vi "Rb_HSRL_v1.0_15m_res.vi"() -> ()   [LabVIEW 2012]
uses:
  C:/Users/H2ODial/Desktop/Shared Telescope WV DIAL Code/Libraries and VIs/PowerMeterCommands.dll
  Shared Telescope WV DIAL Code/Libraries and VIs/PowerMeterCommands.dll
  <vilib>/DAQmx/write.llb/DAQmx Write (Digital 1D Bool NChan 1Samp 1Line).vi
  <vilib>/DAQmx/miscellaneous.llb/DAQmx Fill In Error Info.vi
  <vilib>/Analysis/baseanly.llb/Mean (DBL).vi
  NCAR_DIAL_Labview/AMCS_Data.vi
  Libraries and VIs/Scalar_Data.vi
  <vilib>/Analysis/NI_AALBase.lvlib
  Libraries and VIs/Scalar_Data_2.vi
  Libraries and VIs/Scalar_Data_4.vi
  Libraries and VIs/Scalar_Data_3.vi
  Shared Telescope WV DIAL Code/bristol/CLDevIFace.dll
panel:
  out "FileHour":i32=22
  out "L_Count":i32=314
  out "background start":u32=534
  in  "Tab Control 2":enum32{"WV ND narrow", "WV ND wide"}(tab)=enum."WV ND wide"
  out "RingBuffer offline near":dbl[][](array[numeric])
  out "RingBuffer aerosol near":dbl[][](array[numeric])
  in  "?":T1(tab)=enum."NRB combined"
  out "NRB":dbl[][](graph) caption="Water Vapor Number Density"
  out "NRB 2":dbl[][](graph)=[[0.0006041726529339577, 3.7193787603040805e-05, 3.074896066816216e-05, 4.770145553696684e-05, 7.251392535345536e-05, 0.00010516026017191158, 0.00015207278442684095, 0.00021703896370834744, 0.0002984480988834696, 0.0004093343578366007, 0.0005470560080267362, 0.0007198538987867779, 0.0009396502763554047, 0.0012021835436913518, 0.0015364865779630445, 0.0019279361150240316, 0.0024003604564710023, 0.0029556420530327627, 0.0035799089491286695, 0.004304541171244636, 0.005152810472118787, 0.006171071816967221, 0.007336763695905082, 0.008707520567026136, 0.01017449514748215, 0.011772772340331295, 0.013524884389137577, 0.015341812039428549, 0.017348824658566273, 0.019475636480752727, 0.021601086546037672, 0.02380481304574997, 0.02608445492869741, 0.028360551643139206, 0.030718590319288325, 0.03312680937217094, 0.03549024795270195, 0.03783837645383283, 0.04012219712763372, 0.04250981000176668, 0.044828450558781714, 0.04728053416880318, 0.04984268526006494, 0.0521315574013464, 0.054573984158249905, 0.056762556916223, 0.05892610037044928, 0.06119757571231991, 0.06332053027960594, 0.06531927169904322, 0.06723106201969582, 0.06903054395432445, 0.07061647240492175, 0.07213854154224807, 0.07357196076661428, 0.07475226903500741, 0.07624919928103521, 0.07759010121579418, 0.07885548967938193, 0.08021621669987343, 0.08124765580213601, 0.08236653158699134, 0.08351094727159601, 0.08432126957213373, 0.08514676662031577, 0.08597626589255665, 0.08673988804567571, 0.08759949974634346, 0.08848399450328287, 0.08900381219190334, 0.08964787073734286, 0.09025115411555623, 0.0905283068966542, 0.09100012458273404, 0.09150901738585414, 0.09198604872632336, 0.0926586625260569, 0.09306452132773692, 0.093021602216273, 0.09320383514439438, 0.09329282371608977, 0.09357354518332203, 0.09398320828554164, 0.09438699769115352, 0.09413753694666852, 0.0948052588692632, 0.09497790750110588, 0.09484330743286604, 0.09549799508818226, 0.09539843311384517, 0.0952913565982388, 0.09554342190445454, 0.09553947780494176, 0.09582968317978471, 0.09564115749371307, 0.09505642155282434, 0.09429336706098984, 0.09303860704925615, 0.09201905868900799, 0.09062923434706588, 0.08859052388200775, 0.086006286091639, 0.08369404052031999, 0.081904721905929, 0.08004872100022047, 0.07932582904533776, 0.07850488045233898, 0.07784248370481489, 0.07829820113146535, 0.07817718456168067, 0.07868973099619218, 0.07879420259145382, 0.07842026241447664, 0.07835326207404376, 0.07809468028201165, 0.0790833403261559, 0.08104750888680619, 0.08316741131844003, 0.08645617173459792, 0.08894810268275583, 0.09069525008709582, 0.09186830492409764, 0.09167542640721689, 0.09117907609911939, 0.09078044847825219, 0.0904888883269004, 0.0912124641535658, 0.09221245667395658, 0.09271218317409123, 0.09268672550587362, 0.09164929678500609, 0.08909246838104862, 0.08740150716625646, 0.08551898874896055, 0.08341063493914702, 0.08382395459947903, 0.08281486876215985, 0.08138348106905442, 0.0805959394968051, 0.07742003267120832, 0.07494432120303063, 0.07401315583274465, 0.07247425509566857, 0.07240541265691175, 0.07215582852133233, 0.07207907831538843, 0.07189867090225423, 0.0718332040569795, 0.07213153070685697, 0.07161625534702555, 0.07195959596703647, 0.07149272375067008, 0.07135829810518599, 0.07136001159711242, 0.06990104011744806, 0.06987630922547103, 0.06884467447215356, 0.06823257080581079, 0.06883796260577212, 0.06847144325865764, 0.06734517260711312, 0.06723714193820494, 0.06649908929073146, 0.0674060028804214, 0.06927035231342661, 0.06945789501223798, 0.06966274036787448, 0.0681759990175523, 0.06646660267888853, 0.06525933579552161, 0.06363030761253068, 0.0636144997860727, 0.06369191189378652, 0.06441653257646081, 0.06368179845135223, 0.06213643625440458, 0.06089832506358413, 0.058320573481011655, 0.05967725558532747, 0.05856115358251668, 0.059599703986508296, 0.06033573116455784, 0.058409429492027175, 0.058959839825009026, 0.05696379786517486, 0.05560617195512912, 0.056196112405437204, 0.05634353266040761, 0.05628868456217053, 0.05702440299877362, 0.057239692366992695, 0.05587078750756856, 0.05534171474675636, 0.055016014721345825, 0.05398698695389306, 0.0524964636530886, 0.05166880356011147, 0.05003552152440533, 0.049562020331489515, 0.051877112560926565, 0.052172088817809284, 0.053955908621857, 0.052575656190183465, 0.052057255845492936, 0.0507955882759869, 0.04955602257520721, 0.04952174173150179, 0.049791947433534794, 0.05217084485092792, 0.05144685259985514, 0.05331642431809782, 0.05177469378292136, 0.0487257070373867, 0.04890825602438813, 0.048007045410234074, 0.04818622012199576, 0.04925269626343131, 0.04986393338341831, 0.04860105322071905, 0.04921830012224699, 0.047579260972547464, 0.04679108166071056, 0.0467185509232381, 0.04452202248017214, 0.04540124359150138, 0.04585235124493015, 0.04346851158339598, 0.044830276331367304, 0.04543989298598568, 0.046021190551811586, 0.05002834379151057, 0.05047225805881103, 0.04992168026796387, 0.05085616627991155, 0.05200288053238239, 0.05056443855849414, 0.05122981806572211, 0.048885205277262665, 0.04850397541077456, 0.049441989710825654, 0.05049665877316022, 0.05028550089234136, 0.04661988565933452, 0.046645547880938255, 0.04409610958554134, 0.04525258959471702, 0.04696949495607038, 0.04345277024830872, 0.04512310015573092, 0.045748802174906754, 0.04352087638982649, 0.04574143111706206, 0.04373205593808596, 0.04099138210775028, 0.04224107988946424, 0.0395090076562992, 0.04089183484076426, 0.039065056758817274, 0.03448044280507904, 0.036642233230026584, 0.037975871955755, 0.03841786645234208, 0.04211606108025334, 0.04010127474954111, 0.03315324269857886, 0.03494805507331391, 0.03495744695494245, 0.03731190452688696, 0.042163250407491894, 0.04046697866940592, 0.041967686312648037, 0.037319330850630696, 0.036587053106327226, 0.035683334046114845, 0.03445271926835893, 0.03868934714245255, 0.035046751585014836, 0.03685275429097781, 0.03175210231453753, 0.030612837961132663, 0.03176195345327498, 0.027334033309638617, 0.029180900182185707, 0.02865840834546146, 0.024692599756547362, 0.028846881603003485, 0.027710252601683617, 0.0271463616451785, 0.033031871807972034, 0.031118426063762063, 0.035516450652314735, 0.0317593270937277, 0.02880259484360031, 0.02686866254588606, 0.02147381320339014, 0.02149965025192153, 0.022990151503239253, 0.026388513939612456, 0.02545578038086694, 0.025429119622728674, 0.025822281802900048, 0.02524468180256883, 0.02599054050380181, 0.02516669386087913, 0.02551090205112066, 0.0203265957298277, 0.021475081022554975, 0.021043561469039938, 0.018364628869036184, 0.018720587552500965, 0.019901261768221604, 0.02518438548755014, 0.023718103872757065, 0.024130962125967614, 0.019356525904050494, 0.019242576033774845, 0.01957557879878532, 0.019690045998715985, 0.025537381219061506, 0.024257920468234218, 0.024400361376299314, 0.027260112185394682, 0.027839296598898382, 0.023670078435408172, 0.026458849617683574, 0.02633082198123516, 0.022440984172402617, 0.025358281578316287, 0.02435685979145898, 0.02086607078842593, 0.02210307355877256, 0.01943913047031024, 0.01620527149342513, 0.015202754031733812, 0.01257869794949909, 0.015539979726883455, 0.020184590849572564, 0.017759487388499917, 0.018095561255307153, 0.019384571063333245, 0.01416927084808891, 0.022379157570552637, 0.021876468088369096, 0.02077252637847875, 0.02169764331999801, 0.01876314467011202, 0.0209715149156249, 0.017664916654813154, 0.01546464729070044, 0.01566523945804065, 0.014033903002535698, 0.015233910748532533, 0.012385388752067525, 0.009629681175184958, 0.013262514404387455, 0.01472585101517507, 0.022860933244986854, 0.01748948056632007, 0.016504772276149934, 0.014739152225579666, 0.013476648779599306, 0.01845678009403428, 0.018438586402626633, 0.01851612245573369, 0.01511492613370712, 0.020725919810791443, 0.021614056828372277, 0.021868012999440557, 0.023056145435887954, 0.019819022220186062, 0.016583566922346558, 0.014259915677188135, 0.014781268644322328, 0.011182714408497697, 0.011242594967649835, 0.011534969341718871, 0.011972716867189292, 0.013145154589079836, 0.0030906909114922, 0.004609917525458331, 0.0023149795690942843, 0.009454679429801037, 0.020204932639349964, 0.020539446622713443, 0.02466588261751272, 0.011530946627061736, 0.010373812669827698, 0.005177157268376568, 0.003228309463408691, 0.006730392042262006, 0.011105804742031536, 0.01586251718023354, 0.01935602818797239, 0.019936541321503114, 0.008129118486826823, 0.00778377301546927, 0.0003695124616010089, 0.0028732570424632874, 0.012698627123804679, 0.01267471247361873, 0.016643302663523693, 0.019205150480841312, 0.017684577735701913, 0.014449418836640792, 0.01857936241213829, 0.016534205784404298, 0.018657449525901922, 0.01680389187275702, 0.012839133123909214, 0.018074054220304253, 0.014337587540227013, 0.019196167150429416, 0.02017712086168147, 0.007772012350720519, 0.0059856542235612225, 0.0038658020976381434, -0.001211610038685749, 0.0026588266984640006, 0.002847873136112622, 0.002249503156204727, 0.008668141762090026, 0.00846548962847913, 0.01304702938436645, 0.015423065838504587, 0.010911465180731727, 0.0033580279321079533, 0.003590210561130783, 0.0030718746874166254, 0.007018008289627999, 0.012689008733428571, 0.007456705774423298, 0.01200651375887071, 0.008501755137950942, 0.00984800132224176, 0.00951336801095635, 0.008255509107674029, 0.006602229251177009, 0.014846995387272353, 0.010322551017957794, 0.00957424583546323, 0.008570230825333694, -0.0007369830016869763, 0.00680268776517046, 0.004007758037186643, 0.006954645963076217, 0.01081781398041212, 0.007108510226707795, 0.012325990209815242, 0.0018346543299594294, -0.00037566565141508926, 0.004190834566108668, -0.0011997075029852179, 0.00673857284784521, 0.010833018626010922, 0.010616180758992915, 0.015351985425832304, 0.017135478061334263, 0.01203975331201191, 0.011880803878362706, 0.011256476345111953, 0.013963647147185716, 0.017863253979310968, 0.01966297280690196, 0.009625081362139031, 0.009192833987779899, 0.015358617240372094, 0.0105862084342294, 0.014150967427764961, 0.012243469345682755, 0.005579922613068284, 0.008803739750438582, 0.004976648336493482, -0.007196315088714143, -0.002796200190110646, -0.0037143500570671287, -0.009521900470303567, -0.0035795151876628945, -0.004554081320388369, -0.00821791805383435, 0.0026015707836290103, 0.009097049423122174, 0.010831762895684778, 0.0109619495385428, 0.011927030178565896, 0.008991275634743796, -0.011478753776895502, -0.01247874025183937, -0.011029890702884463, -0.003565405364506508, 0.011895765754890056, 0.011372105838269473, 0.015263863660221434, 0.006383491336105966, 0.010130143622349968, 0.006882790646430292, -0.004858604026684928, 0.0064874976298614625, -0.004128047613836712, -0.009509548145192852, -0.009502053209695252, -0.022234993005451315, -0.01931000662420272, -0.005874456818578927, -0.006315267117716475, -0.008994568192146921, -0.015201162198915527, -0.022184083454656965, -0.020457589329755464, -0.014696020060882452, -0.024180811697773256, -0.011593475504387623, -0.006086556637311528, -0.009618166637100878, 0.009543898366423168, 0.000282820096403412, -0.0068626538978823195, -0.0008862976099987548, 0.0006290824873365674, 0.009509153013947958, 0.020803085654100693, 0.020932738797131138, 0.02051562415751724, 0.016898339042232292, 0.0055821066209041465, -0.0019204781033461552, 0.003907145183148379, 0.0072943343329344035, 0.0166375814124623, 0.019281108318633014, 0.005223412722166723, -0.007293186459080129, -0.011118978208631936, -0.009345301699687556, -0.003757171178932974, -0.004215485642780951, -0.009162281740601998, -0.007827510266829383, -0.009415758624697988, -0.0006715741260478119, 0.012237677793137763, 0.007980966893190502, 0.00637449302918737, -0.0031311666539790184, -0.005196056738576728, -0.009120032689758912, -0.013698691351727845, -0.006455449361784827, -0.009988370510691364, -0.0028155123857298227, 0.0040232697379379186, 0.01775830173503018, 0.014095098329617138, 0.019981436111423515, 0.013777111307489744, -0.0016681673270184326, 0.0, 0.0, 0.0, 0.0, 0.0]] caption="Water Vapor Number Density"
  out "raw counts":dbl[][](graph) caption="Water Vapor Number Density"
  out "raw counts near":dbl[][](graph)=[[34181.4, 389.4, 74.39999999999998, 49.39999999999998, 69.39999999999998, 41.39999999999998, 4.399999999999977, 78.39999999999998, 56.39999999999998, 68.39999999999998, 86.39999999999998, 87.39999999999998, 85.39999999999998, 91.39999999999998, 89.39999999999998, 124.39999999999998, 116.39999999999998, 123.39999999999998, 174.39999999999998, 149.39999999999998, 134.39999999999998, 203.39999999999998, 221.39999999999998, 214.39999999999998, 233.39999999999998, 280.4, 299.4, 303.4, 334.4, 322.4, 349.4, 397.4, 334.4, 436.4, 350.4, 392.4, 421.4, 412.4, 467.4, 451.4, 448.4, 474.4, 461.4, 416.4, 460.4, 484.4, 416.4, 476.4, 478.4, 449.4, 450.4, 422.4, 451.4, 425.4, 432.4, 412.4, 430.4, 379.4, 396.4, 386.4, 358.4, 346.4, 334.4, 335.4, 331.4, 319.4, 313.4, 329.4, 280.4, 275.4, 282.4, 302.4, 302.4, 294.4, 263.4, 285.4, 264.4, 317.4, 242.39999999999998, 221.39999999999998, 240.39999999999998, 273.4, 213.39999999999998, 228.39999999999998, 218.39999999999998, 212.39999999999998, 240.39999999999998, 180.39999999999998, 209.39999999999998, 199.39999999999998, 198.39999999999998, 200.39999999999998, 162.39999999999998, 180.39999999999998, 227.39999999999998, 199.39999999999998, 148.39999999999998, 151.39999999999998, 146.39999999999998, 178.39999999999998, 144.39999999999998, 158.39999999999998, 146.39999999999998, 120.39999999999998, 132.39999999999998, 125.39999999999998, 140.39999999999998, 94.39999999999998, 78.39999999999998, 106.39999999999998, 128.39999999999998, 114.39999999999998, 93.39999999999998, 89.39999999999998, 78.39999999999998, 78.39999999999998, 80.39999999999998, 102.39999999999998, 107.39999999999998, 86.39999999999998, 64.39999999999998, 84.39999999999998, 74.39999999999998, 84.39999999999998, 79.39999999999998, 123.39999999999998, 104.39999999999998, 59.39999999999998, 98.39999999999998, 99.39999999999998, 65.39999999999998, 77.39999999999998, 95.39999999999998, 47.39999999999998, 56.39999999999998, 51.39999999999998, 83.39999999999998, 59.39999999999998, 91.39999999999998, 59.39999999999998, 55.39999999999998, 37.39999999999998, 43.39999999999998, 38.39999999999998, 58.39999999999998, 73.39999999999998, 50.39999999999998, 77.39999999999998, 38.39999999999998, 70.39999999999998, 46.39999999999998, 27.399999999999977, 53.39999999999998, 31.399999999999977, 44.39999999999998, 66.39999999999998, 42.39999999999998, -0.6000000000000227, 31.399999999999977, 21.399999999999977, 54.39999999999998, 34.39999999999998, 41.39999999999998, 22.399999999999977, 41.39999999999998, 73.39999999999998, 22.399999999999977, 67.39999999999998, 21.399999999999977, 12.399999999999977, 29.399999999999977, 57.39999999999998, 79.39999999999998, 46.39999999999998, 11.399999999999977, 48.39999999999998, 3.3999999999999773, 16.399999999999977, 43.39999999999998, 43.39999999999998, 18.399999999999977, 39.39999999999998, 50.39999999999998, 10.399999999999977, 30.399999999999977, 37.39999999999998, 32.39999999999998, 26.399999999999977, 2.3999999999999773, 3.3999999999999773, 17.399999999999977, -3.6000000000000227, 19.399999999999977, 25.399999999999977, 18.399999999999977, 16.399999999999977, -6.600000000000023, 45.39999999999998, 30.399999999999977, 39.39999999999998, 38.39999999999998, 34.39999999999998, 0.39999999999997726, 17.399999999999977, 35.39999999999998, 9.399999999999977, 23.399999999999977, 9.399999999999977, 11.399999999999977, 10.399999999999977, 33.39999999999998, 41.39999999999998, 13.399999999999977, 25.399999999999977, 23.399999999999977, 17.399999999999977, -6.600000000000023, 7.399999999999977, 1.3999999999999773, 2.3999999999999773, 19.399999999999977, -1.6000000000000227, 9.399999999999977, 7.399999999999977, 30.399999999999977, -8.600000000000023, 50.39999999999998, 18.399999999999977, -4.600000000000023, 23.399999999999977, 45.39999999999998, 18.399999999999977, 24.399999999999977, 25.399999999999977, 20.399999999999977, -2.6000000000000227, 15.399999999999977, 22.399999999999977, 11.399999999999977, 6.399999999999977, 18.399999999999977, -7.600000000000023, 11.399999999999977, 7.399999999999977, -2.6000000000000227, 21.399999999999977, 55.39999999999998, 1.3999999999999773, -9.600000000000023, 5.399999999999977, 22.399999999999977, 8.399999999999977, 26.399999999999977, 19.399999999999977, 1.3999999999999773, 20.399999999999977, 10.399999999999977, 10.399999999999977, 16.399999999999977, 32.39999999999998, 8.399999999999977, -6.600000000000023, 27.399999999999977, 1.3999999999999773, -4.600000000000023, 5.399999999999977, 28.399999999999977, 18.399999999999977, -5.600000000000023, 17.399999999999977, 0.39999999999997726, -0.6000000000000227, 3.3999999999999773, 21.399999999999977, 17.399999999999977, -7.600000000000023, 16.399999999999977, 32.39999999999998, 48.39999999999998, 23.399999999999977, 4.399999999999977, 8.399999999999977, 14.399999999999977, 14.399999999999977, -1.6000000000000227, 22.399999999999977, -8.600000000000023, -9.600000000000023, 14.399999999999977, 5.399999999999977, 3.3999999999999773, 12.399999999999977, -25.600000000000023, 3.3999999999999773, -11.600000000000023, 6.399999999999977, 4.399999999999977, 12.399999999999977, -2.6000000000000227, 3.3999999999999773, 25.399999999999977, 55.39999999999998, -3.6000000000000227, 1.3999999999999773, 3.3999999999999773, -2.6000000000000227, -2.6000000000000227, -13.600000000000023, 5.399999999999977, 16.399999999999977, 30.399999999999977, 42.39999999999998, -11.600000000000023, 6.399999999999977, 9.399999999999977, 55.39999999999998, 8.399999999999977, -23.600000000000023, 13.399999999999977, 10.399999999999977, -23.600000000000023, -7.600000000000023, -6.600000000000023, 1.3999999999999773, 23.399999999999977, 10.399999999999977, -5.600000000000023, 3.3999999999999773, -35.60000000000002, 28.399999999999977, -19.600000000000023, -10.600000000000023, 9.399999999999977, -26.600000000000023, 8.399999999999977, -15.600000000000023, -9.600000000000023, 17.399999999999977, 3.3999999999999773, 3.3999999999999773, -8.600000000000023, 41.39999999999998, 24.399999999999977, -2.6000000000000227, 31.399999999999977, 19.399999999999977, 9.399999999999977, -8.600000000000023, -19.600000000000023, 3.3999999999999773, -20.600000000000023, -8.600000000000023, -17.600000000000023, 12.399999999999977, -14.600000000000023, -34.60000000000002, 24.399999999999977, 17.399999999999977, 5.399999999999977, 5.399999999999977, 15.399999999999977, 3.3999999999999773, 4.399999999999977, 12.399999999999977, 6.399999999999977, -18.600000000000023, 2.3999999999999773, -17.600000000000023, 15.399999999999977, 39.39999999999998, 20.399999999999977, -8.600000000000023, 2.3999999999999773, 15.399999999999977, 21.399999999999977, 3.3999999999999773, 6.399999999999977, 6.399999999999977, 15.399999999999977, -17.600000000000023, -33.60000000000002, -2.6000000000000227, 0.39999999999997726, 3.3999999999999773, -19.600000000000023, -3.6000000000000227, 23.399999999999977, 15.399999999999977, 0.39999999999997726, -10.600000000000023, -2.6000000000000227, 6.399999999999977, 0.39999999999997726, 6.399999999999977, -8.600000000000023, 9.399999999999977, -14.600000000000023, -8.600000000000023, -3.6000000000000227, 2.3999999999999773, 9.399999999999977, 15.399999999999977, 0.39999999999997726, -6.600000000000023, 9.399999999999977, -19.600000000000023, -28.600000000000023, 16.399999999999977, 38.39999999999998, 26.399999999999977, 2.3999999999999773, -30.600000000000023, -5.600000000000023, -3.6000000000000227, -5.600000000000023, 9.399999999999977, -6.600000000000023, 2.3999999999999773, 5.399999999999977, -13.600000000000023, 17.399999999999977, -0.6000000000000227, 4.399999999999977, -22.600000000000023, 5.399999999999977, -23.600000000000023, 14.399999999999977, -9.600000000000023, -44.60000000000002, -12.600000000000023, -3.6000000000000227, -14.600000000000023, 3.3999999999999773, -14.600000000000023, -3.6000000000000227, -6.600000000000023, 19.399999999999977, 47.39999999999998, 28.399999999999977, 26.399999999999977, -12.600000000000023, 5.399999999999977, -47.60000000000002, 19.399999999999977, 14.399999999999977, 47.39999999999998, -35.60000000000002, -25.600000000000023, -9.600000000000023, -19.600000000000023, -23.600000000000023, 8.399999999999977, 2.3999999999999773, -4.600000000000023, -10.600000000000023, 6.399999999999977, 0.39999999999997726, -22.600000000000023, 2.3999999999999773, 29.399999999999977, 20.399999999999977, 23.399999999999977, 20.399999999999977, 2.3999999999999773, -6.600000000000023, 10.399999999999977, 2.3999999999999773, -16.600000000000023, -18.600000000000023, -7.600000000000023, -29.600000000000023, 21.399999999999977, -7.600000000000023, -27.600000000000023, 3.3999999999999773, 18.399999999999977, 31.399999999999977, 2.3999999999999773, -29.600000000000023, 29.399999999999977, -15.600000000000023, 18.399999999999977, 44.39999999999998, -31.600000000000023, 16.399999999999977, 0.39999999999997726, -32.60000000000002, 5.399999999999977, -19.600000000000023, -5.600000000000023, -12.600000000000023, -12.600000000000023, 20.399999999999977, -39.60000000000002, 16.399999999999977, -1.6000000000000227, 26.399999999999977, 23.399999999999977, -24.600000000000023, 12.399999999999977, 18.399999999999977, 9.399999999999977, -8.600000000000023, 7.399999999999977, 8.399999999999977, 5.399999999999977, 6.399999999999977, -0.6000000000000227, -4.600000000000023, -12.600000000000023, 16.399999999999977, -3.6000000000000227, -31.600000000000023, -23.600000000000023, 17.399999999999977, 25.399999999999977, 17.399999999999977, 11.399999999999977, -7.600000000000023, -14.600000000000023, 6.399999999999977, 3.3999999999999773, 20.399999999999977, 12.399999999999977, -5.600000000000023, -26.600000000000023, -31.600000000000023, 11.399999999999977, 26.399999999999977, -19.600000000000023, -14.600000000000023, 8.399999999999977, 6.399999999999977, 2.3999999999999773, -16.600000000000023, 17.399999999999977, 10.399999999999977, 0.39999999999997726, -4.600000000000023, 27.399999999999977, -20.600000000000023, -1.6000000000000227, 40.39999999999998, 16.399999999999977, -22.600000000000023, -22.600000000000023, -22.600000000000023, -14.600000000000023, -19.600000000000023, -1.6000000000000227, 18.399999999999977, -23.600000000000023, -10.600000000000023, 12.399999999999977, -3.6000000000000227, 4.399999999999977, -10.600000000000023, 39.39999999999998, 8.399999999999977, 0.0]] caption="Water Vapor Number Density"
  out "HSRL combined Smoothed":dbl[](array[numeric])=[8698.912832369948, 146.95618497109825, 54.04867052023122, 47.1671676300578, 45.88971098265895, 46.214855491329466, 49.099248554913295, 53.648381502890174, 58.2856647398844, 64.74809248554915, 71.50965317919076, 79.06167630057804, 87.92728323699421, 96.98797687861271, 107.9691907514451, 119.05734104046243, 131.28855491329483, 144.17728323699424, 156.71052023121388, 170.0356647398844, 184.5920231213873, 201.3940462427746, 219.0284393063584, 238.69028901734106, 256.98797687861276, 274.87236994219654, 292.76832369942196, 308.74953757225427, 325.4200578034682, 341.3087861271676, 354.47930635838145, 366.5631213872831, 377.6483815028902, 386.7668786127167, 395.29289017341034, 402.8969364161849, 408.60069364161836, 412.9894219653178, 415.7350867052022, 418.71341040462414, 420.26832369942184, 422.39115606936406, 424.8001156069363, 424.3434682080924, 424.6989595375722, 422.7423121387282, 420.3897109826588, 418.60069364161836, 415.63682080924843, 411.7943352601154, 407.40705202312125, 402.39838150289006, 396.28132947976866, 389.99375722543346, 383.43739884393057, 375.8290173410404, 370.04433526011553, 363.7032947976878, 357.23508670520226, 351.4084971098265, 344.3781502890173, 337.9720809248554, 331.89693641618493, 324.7509826589595, 317.940289017341, 311.404161849711, 304.882485549133, 298.93306358381506, 293.27988439306364, 286.65416184971104, 280.6700578034683, 274.78132947976883, 268.1440462427746, 262.32179190751447, 256.8160115606937, 251.42005780346824, 246.73508670520232, 241.51543352601158, 235.3463583815029, 229.9619653179191, 224.54578034682083, 219.77265895953764, 215.4576300578035, 211.2712138728324, 205.79578034682083, 202.47063583815032, 198.2119653179191, 193.46774566473994, 190.45618497109828, 186.06167630057809, 181.79867052023124, 178.3449132947977, 174.52988439306358, 171.36080924855494, 167.4489595375723, 162.98364161849713, 158.36658959537573, 153.09491329479772, 148.38104046242773, 143.23942196531792, 137.26687861271677, 130.67150289017343, 124.70907514450869, 119.71341040462428, 114.78855491329479, 111.61947976878612, 108.41283236994221, 105.51976878612717, 104.20040462427747, 102.1584971098266, 100.98508670520232, 99.32323699421967, 97.11225433526013, 95.33624277456647, 93.37815028901736, 92.93739884393064, 93.62381502890173, 94.45040462427747, 96.54000000000002, 97.67294797687862, 97.95184971098269, 97.59924855491332, 95.81890173410406, 93.77121387283239, 91.87526011560695, 90.13393063583814, 89.43017341040462, 89.00387283236994, 88.1050289017341, 86.7321965317919, 84.45907514450866, 80.86658959537573, 78.14549132947977, 75.32757225433525, 72.38826589595377, 71.68161849710984, 69.79000000000002, 67.5949132947977, 65.98219653179193, 62.482196531791935, 59.63104046242776, 58.064566473988464, 56.06601156069365, 55.23797687861273, 54.29144508670521, 53.493757225433534, 52.63682080924856, 51.88104046242774, 51.39982658959537, 50.355028901734094, 49.92872832369941, 48.95473988439305, 48.226416184971086, 47.60358381502889, 46.03132947976877, 45.427283236994214, 44.18884393063583, 43.24375722543351, 43.08046242774566, 42.317456647398835, 41.10647398843929, 40.53566473988438, 39.600693641618484, 39.65271676300577, 40.256763005780336, 39.881040462427734, 39.52121387283236, 38.219190751445076, 36.82179190751444, 35.729306358381486, 34.43161849710981, 34.024104046242755, 33.67294797687859, 33.66572254335258, 32.90271676300576, 31.740867052023102, 30.758208092485532, 29.12670520231212, 29.472080924855476, 28.600693641618484, 28.787109826589578, 28.82323699421964, 27.59924855491328, 27.557341040462415, 26.337687861271668, 25.434508670520227, 25.43017341040462, 25.226416184971093, 24.93595375722543, 24.996647398843926, 24.82901734104046, 23.98364161849711, 23.511098265895953, 23.132485549132944, 22.46774566473988, 21.625260115606935, 21.068901734104045, 20.19751445086705, 19.805895953757222, 20.524104046242776, 20.435953757225434, 20.925838150289017, 20.19028901734104, 19.79578034682081, 19.128150289017345, 18.480751445086707, 18.29, 18.213410404624277, 18.901271676300578, 18.461965317919077, 18.95184971098266, 18.230751445086707, 16.996647398843933, 16.901271676300578, 16.435953757225434, 16.34491329479769, 16.55300578034682, 16.605028901734105, 16.037109826589592, 16.09346820809248, 15.417167630057804, 15.025549132947976, 14.868034682080925, 14.042890173410404, 14.193179190751442, 14.207630057803465, 13.350693641618497, 13.648381502890173, 13.713410404624277, 13.768323699421968, 14.837687861271679, 14.840578034682085, 14.553005780346824, 14.698959537572257, 14.902716763005781, 14.368034682080925, 14.43450867052023, 13.658497109826587, 13.438843930635837, 13.584797687861272, 13.75965317919075, 13.589132947976879, 12.495202312138726, 12.399826589595376, 11.626705202312138, 11.834797687861274, 12.184508670520232, 11.181618497109827, 11.518323699421964, 11.584797687861272, 10.93306358381503, 11.399826589595378, 10.813121387283237, 10.055895953757226, 10.281329479768786, 9.5414450867052, 9.798670520231212, 9.288554913294798, 8.135375722543353, 8.579017341040462, 8.823236994219654, 8.85791907514451, 9.636820809248555, 9.106473988439305, 7.47208092485549, 7.817456647398842, 7.761098265895953, 8.222080924855492, 9.22208092485549, 8.785664739884393, 9.044335260115606, 7.983641618497109, 7.769768786127167, 7.522658959537571, 7.210520231213872, 8.038554913294796, 7.2293063583815025, 7.547225433526012, 6.456184971098265, 6.180173410404624, 6.3665895953757214, 5.44028901734104, 5.766878612716763, 5.623815028901734, 4.811676300578035, 5.581907514450867, 5.324682080924855, 5.180173410404623, 6.25965317919075, 5.856473988439305, 6.638265895953755, 5.895491329479768, 5.310231213872832, 4.920057803468207, 3.905606936416185, 3.88393063583815, 4.125260115606936, 4.703294797687861, 4.506763005780346, 4.47208092485549, 4.511098265895953, 4.381040462427745, 4.480751445086704, 4.310231213872831, 4.34057803468208, 3.4359537572254326, 3.6064739884393053, 3.511098265895953, 3.0443352601156066, 3.083352601156069, 3.2567630057803467, 4.0949132947976885, 3.8319075144508674, 3.873815028901734, 3.0876878612716756, 3.0501156069364157, 3.0833526011560686, 3.0819075144508665, 3.9720809248554914, 3.7495375722543347, 3.7480924855491327, 4.161387283236994, 4.223526011560693, 3.5689017341040463, 3.964855491329479, 3.921502890173409, 3.32179190751445, 3.7307514450867045, 3.561676300578034, 3.0327745664739876, 3.193179190751444, 2.7914450867052016, 2.313121387283236, 2.1570520231213863, 1.7741040462427735, 2.178728323699421, 2.8131213872832372, 2.460520231213873, 2.492312138728324, 2.6541618497109827, 1.928728323699421, 3.028439306358381, 2.9431791907514446, 2.778439306358381, 2.885375722543352, 2.4807514450867045, 2.7567630057803463, 2.308786127167629, 2.0096531791907504, 2.0241040462427735, 1.80300578034682, 1.9460693641618487, 1.5732369942196525, 1.216300578034681, 1.6657225433526004, 1.8391329479768779, 2.8391329479768777, 2.159942196531791, 2.0269942196531776, 1.8001156069364148, 1.6368208092485537, 2.2293063583815016, 2.2148554913294785, 2.211965317919074, 1.7957803468208082, 2.4489595375722537, 2.5399999999999996, 2.555895953757225, 2.6801734104046235, 2.291445086705201, 1.9070520231213859, 1.6310404624277446, 1.6816184971098254, 1.2654335260115595, 1.2654335260115595, 1.291445086705201, 1.3333526011560681, 1.4561849710982648, 0.34057803468208026, 0.505317919075144, 0.25242774566473924, 1.0255491329479767, 2.1801734104046235, 2.204739884393063, 2.6339306358381496, 1.2249710982658948, 1.0963583815028892, 0.5443352601156056, 0.33768786127167505, 0.7004046242774554, 1.1498265895953745, 1.6339306358381491, 1.983641618497109, 2.0327745664739876, 0.8246820809248548, 0.7856647398843923, 0.03710982658959415, 0.28710982658959416, 1.262543352601155, 1.2538728323699408, 1.638265895953756, 1.8810404624277444, 1.7235260115606925, 1.401271676300577, 1.7928901734104037, 1.5876878612716754, 1.7827745664739876, 1.5978034682080917, 1.2148554913294785, 1.7018497109826582, 1.343468208092485, 1.7899999999999994, 1.8723699421965312, 0.7177456647398832, 0.5501156069364149, 0.35358381502890057, -0.11028901734104167, 0.24086705202312014, 0.2567630057803456, 0.20184971098265772, 0.7741040462427735, 0.7524277456647388, 1.1541618497109816, 1.3579190751445076, 0.9561849710982646, 0.29289017341040346, 0.31167630057803347, 0.2654335260115595, 0.6035838150289005, 1.0862427745664727, 0.6353757225433513, 1.018323699421964, 0.7177456647398832, 0.827572254335259, 0.7957803468208081, 0.6873988439306347, 0.5472254335260104, 1.2249710982658946, 0.8478034682080914, 0.7827745664739871, 0.6975144508670509, -0.059710982658960646, 0.5486705202312125, 0.32179190751444964, 0.5558959537572241, 0.8608092485549121, 0.5631213872832358, 0.9720809248554901, 0.14404624277456524, -0.029364161849712148, 0.3261271676300566, -0.09294797687861393, 0.5197687861271664, 0.8319075144508659, 0.8116763005780334, 1.1686127167630045, 1.2986705202312128, 0.9084971098265884, 0.8926011560693629, 0.842023121387282, 1.0399999999999987, 1.3246820809248543, 1.4518497109826578, 0.7076300578034669, 0.6729479768786115, 1.1194797687861262, 0.7683236994219643, 1.0226589595375712, 0.8810404624277448, 0.39982658959537454, 0.6281502890173398, 0.35358381502890046, -0.5091329479768798, -0.19699421965318042, -0.2605780346820822, -0.6652023121387295, -0.24901734104046358, -0.31549132947977, -0.5669364161849723, 0.17872832369942074, 0.6223699421965305, 0.7379768786127158, 0.743757225433525, 0.8058959537572246, 0.6050289017341031, -0.7692485549132959, -0.8328323699421976, -0.7331213872832381, -0.2360115606936427, 0.7842196531791895, 0.7466473988439294, 0.9980924855491318, 0.41572254335259995, 0.6570520231213861, 0.4446242774566462, -0.3126011560693654, 0.41572254335259995, -0.2634682080924868, -0.604508670520232, -0.6016184971098275, -1.4021965317919085, -1.2128901734104056, -0.36751445086705326, -0.39352601156069483, -0.5582658959537584, -0.9397687861271687, -1.3660693641618509, -1.2547976878612728, -0.8978612716763018, -1.4715606936416195, -0.7027745664739893, -0.3675144508670528, -0.5784971098265903, 0.5717919075144497, 0.016878612716761776, -0.40797687861271803, -0.0524855491329492, 0.037109826589594136, 0.5587861271676288, 1.2177456647398832, 1.2206358381502878, 1.1917341040462417, 0.9778612716762993, 0.32179190751444964, -0.11028901734104168, 0.2235260115606924, 0.41572254335259995, 0.9446242774566462, 1.0905780346820797, 0.29433526011560573, -0.4094219653179203, -0.6218497109826602, -0.5206936416184984, -0.20855491329479886, -0.23312138728323822, -0.504797687861273, -0.42965317919075263, -0.5149132947976891, -0.03658959537572379, 0.6642774566473977, 0.43161849710982536, 0.3434682080924843, -0.16809248554913425, -0.2779190751445099, -0.4860115606936429, -0.727341040462429, -0.3415028901734116, -0.5264739884393075, -0.14786127167630178, 0.21052023121387162, 0.9258381502890162, 0.7321965317919064, 1.0342196531791896, 0.7105202312138718, -0.0857225433526024]
  out "HSRL combined":dbl[](array[numeric])=[8700.534921465967, 148.02575916230356, 54.68642670157071, 48.36803664921469, 46.66548429319374, 47.40795811518327, 50.00808900523563, 53.89945026178015, 58.77379581151838, 64.78721204188487, 71.63505235602099, 79.05651832460737, 87.69755235602096, 97.21424083769634, 108.05390052356017, 119.27608638743452, 131.62065445026175, 144.76823298429318, 157.34480366492153, 171.9154842931938, 186.94918848167544, 202.46653141361264, 220.06273560209425, 238.01626963350787, 256.41352094240835, 274.43773560209416, 292.1386518324606, 309.2695418848166, 325.5741884816751, 341.67562827225095, 355.7276570680624, 368.3045549738215, 379.9374083769629, 389.7620157068058, 398.64486910994714, 406.1612303664916, 412.1811910994759, 416.97405759162257, 421.1370157068058, 424.00121727748643, 425.7302748691095, 427.1327617801042, 427.53852094240784, 427.44002617800993, 426.87850785340265, 425.7551439790571, 424.18511780104666, 422.1641753926697, 419.192971204188, 415.2862303664916, 410.56502617800993, 405.65763089005185, 399.4681675392665, 393.6082198952875, 387.2957198952875, 380.28950261780057, 374.59807591622985, 368.10691099476384, 361.8889790575911, 356.0303403141356, 349.29473821989484, 342.43577225130855, 335.6314528795809, 328.4233376963349, 321.78164921465947, 315.36934554973806, 308.57582460732965, 302.14290575916215, 295.55749999999983, 289.22831151832446, 283.2927748691098, 276.9020680628271, 270.29866492146584, 264.31306282722505, 258.0525916230367, 252.55291884816756, 247.75252617801047, 242.33531413612565, 237.26332460732988, 232.08204188481676, 227.0381937172775, 222.06306282722514, 217.32418848167535, 212.73125654450257, 207.86607329842928, 204.05717277486912, 199.5653534031414, 195.2027879581152, 191.2283115183247, 186.66450261780113, 183.03688481675402, 179.05226439790584, 175.33171465968593, 171.63047120418852, 167.68871727748694, 163.6566492146597, 159.17268324607332, 154.23485602094246, 148.95573298429326, 143.51397905759165, 137.4756937172775, 131.7335471204188, 126.44853403141354, 121.4825654450261, 117.31797120418842, 113.227002617801, 109.52117801047117, 106.67693717277484, 104.20704188481672, 102.45147905759158, 100.49205497382195, 98.4933638743455, 96.95573298429316, 95.54212041884817, 95.18446335078535, 95.7387827225131, 96.78982984293194, 98.14617801047119, 100.12850785340312, 101.38341623036648, 101.96947643979055, 101.88603403141359, 100.43609947643976, 98.48191099476438, 96.40075916230364, 94.29899214659687, 92.42890052356022, 90.72569371727752, 87.99238219895292, 85.29015706806288, 81.83891361256552, 78.135052356021, 75.56077225130896, 73.17628272251314, 71.21456806282728, 69.53721204188487, 67.79081151832466, 65.56895287958122, 63.62000000000006, 61.32484293193723, 59.36509162303672, 57.96195026178016, 56.20769633507858, 55.336295811518376, 54.32091623036654, 53.30324607329847, 52.79670157068067, 52.1144371727749, 51.280013089005266, 50.230929319371754, 49.23649214659689, 48.18544502617804, 47.12000000000003, 46.3971596858639, 45.472748691099504, 44.45769633507855, 43.701151832460745, 43.11149214659687, 42.834332460733, 42.30553664921467, 41.73092931937173, 40.884397905759165, 39.962931937172776, 39.5244502617801, 39.03001308900524, 38.582041884816746, 37.86836387434555, 37.12785340314136, 36.50448952879581, 36.107238219895294, 35.611819371727755, 34.96391361256545, 34.30979057591624, 33.462277486911, 32.58400523560209, 31.833678010471207, 30.992709424083774, 30.568298429319377, 30.19297120418848, 29.993363874345555, 29.7090052356021, 28.86901832460733, 28.326806282722515, 27.5673167539267, 26.94002617801047, 26.738455497382194, 26.401740837696334, 26.01103403141361, 25.61967277486911, 24.974712041884807, 24.475693717277473, 24.39061518324606, 23.882761780104698, 23.498599476439782, 23.47078534031413, 22.50416230366492, 22.25252617801047, 22.050301047120417, 21.472748691099476, 21.55684554973822, 21.611164921465967, 21.25318062827225, 20.75547120418848, 20.395196335078538, 20.11116492146597, 19.68740837696335, 19.63734293193717, 19.740418848167536, 19.108874345549737, 18.785248691099476, 18.309136125654447, 18.019541884816746, 17.91352094240837, 18.157630890052353, 18.12785340314136, 17.66319371727748, 17.166793193717275, 16.85200261780104, 16.499253926701567, 16.64486910994764, 16.571897905759158, 16.067971204188478, 15.925628272251306, 15.224057591623033, 15.109528795811514, 14.935445026178005, 14.232238219895287, 14.11836387434555, 14.009397905759162, 13.93282722513089, 14.277395287958113, 14.505471204188478, 14.32746073298429, 14.427264397905756, 14.38603403141361, 14.196897905759162, 14.164829842931939, 13.643232984293196, 13.87098167539267, 13.69657068062827, 13.832696335078534, 14.041465968586387, 13.581714659685863, 13.238782722513088, 12.775431937172772, 12.465876963350786, 12.159267015706806, 11.912539267015708, 11.65435863874346, 11.586295811518331, 11.469476439790581, 11.203769633507857, 10.766924083769634, 10.462604712041884, 10.081387434554973, 10.092185863874342, 10.345130890052355, 10.157303664921464, 9.909267015706806, 9.633416230366493, 9.207369109947644, 8.854620418848167, 8.946897905759162, 8.75678010471204, 8.778704188481676, 9.008416230366493, 8.841858638743457, 8.941335078534031, 8.822552356020942, 8.74859947643979, 8.80455497382199, 8.48714659685864, 8.3569109947644, 8.132107329842933, 8.021832460732986, 8.224057591623039, 8.008416230366493, 7.714568062827226, 7.342840314136127, 7.087604712041886, 7.282303664921468, 7.138324607329844, 6.8614921465968575, 6.732565445026175, 6.0254319371727725, 5.94526178010471, 5.876871727748691, 5.729620418848169, 5.885706806282724, 5.831714659685863, 6.335314136125655, 6.232565445026178, 6.096112565445026, 5.912866492146596, 5.4534424083769615, 5.585968586387433, 5.935117801047119, 6.033612565445026, 5.7427094240837695, 5.232565445026176, 4.967840314136122, 4.801282722513085, 4.8929057591623, 4.58204188481675, 4.609201570680625, 4.558808900523557, 4.738128272251305, 5.137997382198949, 4.859528795811514, 4.678573298429315, 4.178246073298426, 3.8978141361256506, 3.6661387434554933, 3.6196727748691053, 3.9393717277486866, 4.286230366492142, 4.380143979057587, 4.1442146596858604, 3.726675392670153, 3.449188481675389, 3.1023298429319337, 3.2957198952879554, 3.539175392670154, 3.4046858638743416, 3.764306282722509, 3.7593979057591578, 3.5849869109947594, 3.802591623036644, 3.2852486910994725, 2.9887827225130854, 2.9691492146596827, 2.5699345549738193, 2.929882198952876, 3.0244502617801, 3.3143717277486866, 3.5201963350785292, 3.6779188481675344, 3.7158769633507807, 3.539175392670153, 3.4020680628272215, 3.023141361256541, 3.085314136125651, 3.1343979057591578, 3.183481675392666, 3.0463743455497343, 3.0234685863874304, 2.9603141361256506, 2.585968586387431, 2.734528795811515, 2.89388743455497, 2.6870811518324578, 2.9534424083769597, 2.7250392670157035, 2.2067146596858627, 2.400431937172773, 2.51037958115183, 2.5437565445026147, 2.6952617801047087, 2.618036649214657, 2.212931937172774, 2.462277486910993, 2.469803664921464, 2.2306020942408358, 2.1429057591623017, 2.0290314136125644, 2.1645026178010456, 2.160248691099475, 2.234201570680627, 2.1396335078534023, 1.9269371727748685, 1.8860340314136117, 1.9747120418848156, 1.8395680628272242, 1.6759554973821984, 1.737801047120418, 1.705405759162303, 1.8071727748691089, 1.7669240837696327, 1.5467015706806284, 1.408612565445027, 1.2633246073298443, 1.2927748691099485, 1.5499738219895294, 1.6445418848167537, 2.0270680628272233, 2.033285340314135, 1.6232722513088995, 1.255471204188481, 1.0535732984293196, 1.2031151832460731, 1.409267015706806, 1.5120157068062823, 1.476348167539267, 1.1507591623036648, 1.1847905759162305, 1.2832853403141367, 1.1003664921465977, 1.1537041884816766, 0.6864267015706816, 0.8408769633507862, 0.9828926701570679, 1.4390445026177998, 1.8146989528795803, 1.3899607329842922, 1.1834816753926702, 0.7636518324607341, 0.8611649214659693, 1.1586125654450272, 1.245000000000001, 1.7122774869109945, 1.460641361256544, 1.386361256544502, 1.5588089005235588, 1.1150916230366492, 1.263979057591623, 1.3951963350785344, 1.3755628272251308, 1.3133900523560207, 1.2803403141361254, 1.283285340314136, 1.1098560209424089, 1.1412696335078538, 1.0071073298429325, 1.1890445026178007, 1.3572382198952875, 1.0283769633507849, 1.0323036649214652, 0.68217277486911, 0.49172774869109975, 0.9900916230366493, 1.0957853403141362, 1.4292277486910994, 1.3611649214659687, 1.364437172774869, 1.2626701570680625, 1.0928403141361254, 1.169738219895288, 0.8048821989528799, 0.542120418848168, 0.44264397905759206, 0.5254319371727751, 0.7083507853403146, 1.2230759162303666, 1.3035732984293193, 1.096439790575916, 1.0977486910994765, 0.5745157068062832, 0.5434293193717283, 0.28492146596858703, 0.3559293193717281, 0.9590052356020944, 0.8441492146596857, 1.3412041884816754, 0.9138481675392668, 0.698534031413613, 0.6085471204188485, 0.23518324607329866, 0.622945026178011, 0.737801047120419, 0.3003010471204191, 0.6694109947643979, 0.6301439790575916, 0.6170549738219899, 0.961623036649215, 0.7358376963350796, 0.7456544502617811, 0.4472251308900531, 0.7214397905759171, 0.6991884816753933, 0.7597251308900528, 0.9004319371727756, 0.822879581151833, 0.7086780104712047, 0.6432329842931941, 0.6157460732984297, 0.4207198952879582, 0.5535732984293196, 0.6599214659685868, 0.5313219895287962, 0.5735340314136129, 0.6445418848167543, 0.43577225130890074, 0.3114267015706809, 0.17922774869109975, 0.29146596858638796, 0.310772251308901, 0.36541884816753967, 0.6298167539267021, 0.4459162303664925, 0.5431020942408382, 0.9066492146596867, 1.135052356020943, 0.8166623036649218, 0.6955890052356023, 0.3974869109947642, 0.03753926701570678, 0.5352486910994768, 0.6291623036649219, 0.7862303664921471, 0.9050130890052361, 0.8343324607329846, 0.8205890052356023, 0.7829581151832467, 0.7456544502617806, 0.30062827225130934, -0.15617801047120328, -0.3227356020942403, -0.22096858638743397, 0.13407068062827276, 0.41384816753926723, 0.4128664921465971, 0.14912303664921486, 0.1900261780104715, 0.2643062827225134, 0.19035340314136154, 0.2656151832460736, 0.23256544502617804, 0.2973560209424084, 0.5810602094240841, 0.7472905759162309, 0.9940183246073303, 0.9223560209424089, 1.068298429319372, 0.8811256544502618, 0.3549476439790577, 0.28786649214659693, 0.3392408376963343, 0.5120157068062817, 0.9285732984293185, 1.0925130890052348, 0.8824345549738221, 0.6985340314136127, 0.40763089005235625, 0.19166230366492157, -0.23471204188481642, -0.421557591623036, 0.0002356020942409498, 0.10854712041884829, 0.5574999999999999, 0.7322382198952877, 0.3726178010471207, 0.47896596858638774, 0.12719895287958116, 0.09643979057591623, 0.028704188481675292, -0.05146596858638755, 0.30815445026178045, 0.45442408376963384, 0.04964659685863909, 0.049319371727749015, -0.22653141361256546, -0.4294109947643979, -0.2589267015706806, -0.543939790575916, -0.2998298429319365]
  out "Off-Line Bin Readings 2":dbl[](array[numeric])=[34447.0, 655.0, 340.0, 315.0, 335.0, 307.0, 270.0, 344.0, 322.0, 334.0, 352.0, 353.0, 351.0, 357.0, 355.0, 390.0, 382.0, 389.0, 440.0, 415.0, 400.0, 469.0, 487.0, 480.0, 499.0, 546.0, 565.0, 569.0, 600.0, 588.0, 615.0, 663.0, 600.0, 702.0, 616.0, 658.0, 687.0, 678.0, 733.0, 717.0, 714.0, 740.0, 727.0, 682.0, 726.0, 750.0, 682.0, 742.0, 744.0, 715.0, 716.0, 688.0, 717.0, 691.0, 698.0, 678.0, 696.0, 645.0, 662.0, 652.0, 624.0, 612.0, 600.0, 601.0, 597.0, 585.0, 579.0, 595.0, 546.0, 541.0, 548.0, 568.0, 568.0, 560.0, 529.0, 551.0, 530.0, 583.0, 508.0, 487.0, 506.0, 539.0, 479.0, 494.0, 484.0, 478.0, 506.0, 446.0, 475.0, 465.0, 464.0, 466.0, 428.0, 446.0, 493.0, 465.0, 414.0, 417.0, 412.0, 444.0, 410.0, 424.0, 412.0, 386.0, 398.0, 391.0, 406.0, 360.0, 344.0, 372.0, 394.0, 380.0, 359.0, 355.0, 344.0, 344.0, 346.0, 368.0, 373.0, 352.0, 330.0, 350.0, 340.0, 350.0, 345.0, 389.0, 370.0, 325.0, 364.0, 365.0, 331.0, 343.0, 361.0, 313.0, 322.0, 317.0, 349.0, 325.0, 357.0, 325.0, 321.0, 303.0, 309.0, 304.0, 324.0, 339.0, 316.0, 343.0, 304.0, 336.0, 312.0, 293.0, 319.0, 297.0, 310.0, 332.0, 308.0, 265.0, 297.0, 287.0, 320.0, 300.0, 307.0, 288.0, 307.0, 339.0, 288.0, 333.0, 287.0, 278.0, 295.0, 323.0, 345.0, 312.0, 277.0, 314.0, 269.0, 282.0, 309.0, 309.0, 284.0, 305.0, 316.0, 276.0, 296.0, 303.0, 298.0, 292.0, 268.0, 269.0, 283.0, 262.0, 285.0, 291.0, 284.0, 282.0, 259.0, 311.0, 296.0, 305.0, 304.0, 300.0, 266.0, 283.0, 301.0, 275.0, 289.0, 275.0, 277.0, 276.0, 299.0, 307.0, 279.0, 291.0, 289.0, 283.0, 259.0, 273.0, 267.0, 268.0, 285.0, 264.0, 275.0, 273.0, 296.0, 257.0, 316.0, 284.0, 261.0, 289.0, 311.0, 284.0, 290.0, 291.0, 286.0, 263.0, 281.0, 288.0, 277.0, 272.0, 284.0, 258.0, 277.0, 273.0, 263.0, 287.0, 321.0, 267.0, 256.0, 271.0, 288.0, 274.0, 292.0, 285.0, 267.0, 286.0, 276.0, 276.0, 282.0, 298.0, 274.0, 259.0, 293.0, 267.0, 261.0, 271.0, 294.0, 284.0, 260.0, 283.0, 266.0, 265.0, 269.0, 287.0, 283.0, 258.0, 282.0, 298.0, 314.0, 289.0, 270.0, 274.0, 280.0, 280.0, 264.0, 288.0, 257.0, 256.0, 280.0, 271.0, 269.0, 278.0, 240.0, 269.0, 254.0, 272.0, 270.0, 278.0, 263.0, 269.0, 291.0, 321.0, 262.0, 267.0, 269.0, 263.0, 263.0, 252.0, 271.0, 282.0, 296.0, 308.0, 254.0, 272.0, 275.0, 321.0, 274.0, 242.0, 279.0, 276.0, 242.0, 258.0, 259.0, 267.0, 289.0, 276.0, 260.0, 269.0, 230.0, 294.0, 246.0, 255.0, 275.0, 239.0, 274.0, 250.0, 256.0, 283.0, 269.0, 269.0, 257.0, 307.0, 290.0, 263.0, 297.0, 285.0, 275.0, 257.0, 246.0, 269.0, 245.0, 257.0, 248.0, 278.0, 251.0, 231.0, 290.0, 283.0, 271.0, 271.0, 281.0, 269.0, 270.0, 278.0, 272.0, 247.0, 268.0, 248.0, 281.0, 305.0, 286.0, 257.0, 268.0, 281.0, 287.0, 269.0, 272.0, 272.0, 281.0, 248.0, 232.0, 263.0, 266.0, 269.0, 246.0, 262.0, 289.0, 281.0, 266.0, 255.0, 263.0, 272.0, 266.0, 272.0, 257.0, 275.0, 251.0, 257.0, 262.0, 268.0, 275.0, 281.0, 266.0, 259.0, 275.0, 246.0, 237.0, 282.0, 304.0, 292.0, 268.0, 235.0, 260.0, 262.0, 260.0, 275.0, 259.0, 268.0, 271.0, 252.0, 283.0, 265.0, 270.0, 243.0, 271.0, 242.0, 280.0, 256.0, 221.0, 253.0, 262.0, 251.0, 269.0, 251.0, 262.0, 259.0, 285.0, 313.0, 294.0, 292.0, 253.0, 271.0, 218.0, 285.0, 280.0, 313.0, 230.0, 240.0, 256.0, 246.0, 242.0, 274.0, 268.0, 261.0, 255.0, 272.0, 266.0, 243.0, 268.0, 295.0, 286.0, 289.0, 286.0, 268.0, 259.0, 276.0, 268.0, 249.0, 247.0, 258.0, 236.0, 287.0, 258.0, 238.0, 269.0, 284.0, 297.0, 268.0, 236.0, 295.0, 250.0, 284.0, 310.0, 234.0, 282.0, 266.0, 233.0, 271.0, 246.0, 260.0, 253.0, 253.0, 286.0, 226.0, 282.0, 264.0, 292.0, 289.0, 241.0, 278.0, 284.0, 275.0, 257.0, 273.0, 274.0, 271.0, 272.0, 265.0, 261.0, 253.0, 282.0, 262.0, 234.0, 242.0, 283.0, 291.0, 283.0, 277.0, 258.0, 251.0, 272.0, 269.0, 286.0, 278.0, 260.0, 239.0, 234.0, 277.0, 292.0, 246.0, 251.0, 274.0, 272.0, 268.0, 249.0, 283.0, 276.0, 266.0, 261.0, 293.0, 245.0, 264.0, 306.0, 282.0, 243.0, 243.0, 243.0, 251.0, 246.0, 264.0, 284.0, 242.0, 255.0, 278.0, 262.0, 270.0, 255.0, 305.0, 274.0]
  out "HSRL molecular Smoothed":dbl[](array[numeric])=[795.0727407407404, 21.774592592592594, 19.25607407407408, 19.56903703703704, 19.55792592592593, 20.594962962962963, 23.276444444444444, 25.220888888888883, 28.232, 30.087555555555554, 33.28014814814814, 37.15237037037037, 39.87274074074074, 43.743111111111105, 46.85977777777777, 49.80792592592593, 54.2394074074074, 58.09125925925925, 62.459777777777774, 67.03014814814814, 69.90977777777778, 73.05422222222222, 75.91348148148147, 80.28200000000001, 84.29866666666668, 89.65977777777779, 93.99496296296297, 97.59496296296298, 102.38200000000002, 105.87088888888891, 109.54125925925928, 112.38200000000002, 115.4671851851852, 118.04866666666669, 119.86162962962966, 122.50977777777781, 123.50237037037041, 123.54866666666669, 125.40051851851855, 126.91348148148151, 127.61718518518522, 129.53570370370375, 129.28200000000004, 128.52644444444448, 129.20051851851855, 128.28570370370375, 127.68570370370375, 127.02088888888892, 125.46162962962968, 124.28385185185189, 123.0375555555556, 120.25422222222227, 119.13385185185189, 116.59681481481485, 114.51162962962967, 113.62459259259262, 111.70792592592595, 111.594962962963, 111.1097777777778, 110.15792592592595, 108.39311111111112, 106.08755555555558, 103.9597777777778, 101.58940740740742, 99.36533333333335, 98.28940740740742, 97.7708888888889, 95.84866666666667, 94.58570370370371, 92.0708888888889, 89.34311111111111, 87.52088888888889, 84.83385185185186, 83.33385185185186, 80.71533333333333, 79.70051851851852, 78.3394074074074, 76.38014814814815, 74.87088888888889, 73.09125925925926, 71.71162962962961, 70.50607407407406, 70.26162962962962, 68.73014814814815, 67.62274074074074, 66.46903703703703, 64.8357037037037, 63.38755555555555, 62.7782962962963, 60.60607407407407, 58.90237037037037, 57.06718518518518, 55.00237037037036, 53.5894074074074, 51.80237037037036, 51.50792592592592, 50.21533333333333, 49.22829629629629, 48.587555555555554, 47.29125925925925, 46.78199999999999, 45.97829629629629, 45.130148148148145, 43.431999999999995, 41.483851851851846, 40.05422222222222, 38.498666666666665, 37.59311111111111, 36.64311111111111, 36.86903703703703, 36.53014814814814, 35.965333333333334, 36.05977777777778, 34.830148148148155, 34.04125925925926, 33.38014814814815, 32.75051851851852, 33.20422222222222, 31.782000000000004, 31.65792592592593, 30.846814814814813, 30.031999999999996, 30.833851851851847, 30.21348148148148, 29.89311111111111, 28.38385185185185, 27.85237037037037, 27.032, 27.80237037037037, 27.89311111111111, 27.1282962962963, 26.530148148148147, 23.704222222222224, 22.141259259259257, 21.217185185185187, 20.833851851851854, 20.90977777777778, 21.09866666666667, 21.811629629629632, 21.96903703703704, 22.50607407407407, 22.526444444444447, 21.64866666666667, 21.57088888888889, 20.715333333333337, 19.732000000000003, 19.40237037037037, 18.894962962962964, 19.00237037037037, 18.515333333333334, 18.15237037037037, 17.328296296296298, 16.743111111111112, 16.889407407407408, 16.617185185185186, 17.26162962962963, 17.306074074074075, 17.037555555555553, 16.637555555555554, 15.046814814814814, 13.633851851851853, 13.50051851851852, 13.417185185185186, 13.732000000000003, 14.037555555555558, 13.954222222222224, 13.543111111111115, 13.24866666666667, 13.60607407407408, 13.572740740740745, 13.085703703703707, 12.872740740740744, 10.972740740740743, 10.143111111111114, 9.707925925925927, 10.282000000000004, 11.639407407407411, 12.41903703703704, 12.983851851851854, 11.237555555555558, 11.174592592592594, 9.533851851851853, 8.550518518518519, 9.398666666666667, 8.909777777777778, 9.478296296296296, 10.593111111111114, 9.707925925925927, 9.452370370370373, 10.967185185185189, 9.335703703703704, 10.60792592592593, 10.452370370370373, 8.837555555555557, 10.078296296296298, 8.769037037037037, 8.087555555555555, 7.4468148148148146, 6.66162962962963, 6.256074074074074, 7.159777777777778, 7.633851851851851, 7.006074074074075, 7.139407407407408, 6.106074074074075, 5.482000000000001, 6.026444444444445, 6.87088888888889, 8.126444444444445, 8.482000000000001, 8.348666666666666, 7.728296296296296, 6.0153333333333325, 5.976444444444444, 6.0079259259259254, 5.517185185185185, 6.361629629629629, 5.96162962962963, 5.785703703703703, 6.559777777777777, 6.341259259259259, 6.328296296296296, 6.209777777777777, 5.185703703703704, 5.607925925925926, 5.004222222222222, 4.767185185185186, 5.615333333333334, 4.928296296296297, 5.959777777777778, 5.378296296296297, 4.765333333333334, 3.806074074074074, 3.594962962962964, 4.024592592592593, 3.856074074074075, 4.093111111111112, 4.246814814814815, 4.080148148148149, 4.150518518518519, 4.663481481481482, 4.543111111111113, 4.361629629629631, 3.4986666666666677, 3.19125925925926, 1.8597777777777786, 1.7431111111111117, 1.9375555555555561, 2.0486666666666675, 3.31162962962963, 3.372740740740741, 3.1560740740740747, 2.7820000000000005, 1.4616296296296305, 1.443111111111112, 2.944962962962964, 3.8282962962962968, 4.659777777777778, 4.4431111111111115, 3.9097777777777782, 3.8708888888888895, 4.407925925925926, 4.785703703703704, 3.933851851851852, 3.119037037037037, 1.8579259259259264, 1.1820000000000008, 2.3708888888888895, 2.9764444444444456, 3.2357037037037046, 4.448666666666667, 3.4394074074074075, 3.8245925925925928, 4.394962962962963, 3.987555555555556, 4.585703703703705, 4.306074074074075, 4.482, 4.557925925925926, 4.500518518518518, 3.894962962962963, 3.0486666666666675, 2.9153333333333338, 2.3801481481481486, 2.574592592592593, 2.9838518518518526, 3.2338518518518518, 3.7412592592592593, 4.691259259259259, 5.324592592592593, 3.6468148148148156, 3.54125925925926, 2.7227407407407416, 2.032000000000001, 2.667185185185186, 2.8097777777777786, 2.2153333333333345, 1.7579259259259266, 2.150518518518519, 1.2838518518518527, 1.7116296296296305, 2.180148148148149, 1.9857037037037044, 1.8708888888888895, 1.9671851851851858, 1.8597777777777784, 1.717185185185186, 1.139407407407408, 0.35792592592592676, -0.058740740740739955, 0.6838518518518528, 1.32088888888889, 2.485703703703705, 1.8134814814814826, 1.017185185185186, 1.4968148148148157, 0.29125925925926, 0.5616296296296305, 1.9079259259259267, 1.619037037037038, 2.5116296296296303, 2.7523703703703712, 1.4245925925925933, 1.1616296296296305, 0.9708888888888897, 0.5523703703703713, 1.293111111111112, 1.4486666666666674, 0.9949629629629637, 1.3412592592592603, 1.2838518518518527, 1.069037037037038, 0.33940740740740816, 0.45977777777777856, -0.669851851851851, -0.9050370370370362, -0.6476296296296288, 0.35051851851851934, -0.3828148148148143, -0.16985185185185128, -0.38466666666666616, -1.3883703703703698, -0.2902222222222215, -0.38096296296296217, -0.20874074074074, 0.17459259259259335, 0.4264444444444452, 1.043111111111112, 1.9023703703703712, 1.6820000000000008, 1.9838518518518526, 1.5616296296296304, 1.2986666666666675, 0.8060740740740749, 0.504222222222223, 1.39125925925926, 1.0579259259259268, 1.8542222222222229, 2.9542222222222225, 1.6764444444444448, 2.898666666666667, 1.878296296296297, 0.4190370370370379, 1.0875555555555565, 0.3634814814814823, 1.3560740740740749, 1.4171851851851858, 0.6227407407407415, 0.028296296296297097, -1.2976296296296288, -0.5494814814814809, 0.6857037037037043, 0.8449629629629636, 0.7468148148148154, -0.0642962962962954, -0.014296296296295363, 0.13200000000000092, 1.265333333333334, 1.54125925925926, 1.1820000000000008, 1.517185185185186, 2.0153333333333343, 1.6116296296296304, 1.6357037037037045, 1.206074074074075, 1.813481481481482, 1.8023703703703706, 1.1468148148148154, 0.7690370370370375, -1.380962962962962, -0.5772592592592584, -0.09762962962962879, 0.9282962962962973, 2.3986666666666676, 3.035703703703705, 3.3097777777777786, 2.435703703703705, 2.0171851851851863, 0.5690370370370379, 0.24311111111111192, 0.7579259259259268, 0.42088888888888965, 0.3523703703703712, 0.74125925925926, 1.3245925925925932, 1.665333333333334, 2.0597777777777786, 2.9431111111111115, 2.2282962962962967, 2.270888888888889, 1.4412592592592595, 0.8745925925925929, 0.7431111111111115, 0.19311111111111146, 0.613481481481482, -0.27170370370370295, 0.1560740740740748, 0.7005185185185192, 1.1375555555555563, 1.554222222222223, 2.4338518518518524, 1.8486666666666673, 1.876444444444445, 1.4949629629629635, 0.35237037037037117, 0.49866666666666737, 1.2245925925925931, 0.5801481481481487, 0.1986666666666671, 0.6338518518518523, -0.6402222222222215, 0.03570370370370449, 0.9894074074074082, 0.9042222222222229, 1.8338518518518525, 1.3634814814814822, 0.8431111111111118, 0.4912592592592601, 0.004222222222223071, 0.05792592592592674, -0.595777777777777, -0.2976296296296289, -0.016148148148147468, 0.25792592592592667, 1.4931111111111117, 0.8486666666666675, 0.5449629629629638, 0.7727407407407415, -0.4920740740740733, -0.24022222222222145, -0.12725925925925846, 0.13200000000000084, 1.1338518518518526, 1.4505185185185194, 1.419037037037038, 1.1616296296296302, 0.7190370370370379, 0.5931111111111119, 0.3912592592592601, -0.014296296296295516, 0.4949629629629637, 0.7820000000000008, 0.5727407407407415, 0.9579259259259267, 0.9690370370370379, 0.7134814814814823, 1.5227407407407414, 0.9097777777777785, 0.17644444444444515, 0.7634814814814823, 0.4560740740740749, 1.4949629629629637, 1.5857037037037045, 1.0468148148148158, 1.8931111111111125, 0.998666666666668, -0.267999999999999, -0.43837037037036947, -0.7902222222222217, -0.4605925925925922, 1.1820000000000008, 0.9060740740740749, 0.09681481481481555, 0.01348148148148226, 0.4394074074074082, 0.5894074074074082, 0.9486666666666674, 0.9523703703703711, 0.03570370370370446, 0.8523703703703711, -0.24948148148148075, -0.12911111111111037, 0.21903703703703778, -0.49948148148148075, -0.24948148148148064, -1.0142962962962954, -0.4605925925925918, -0.26244444444444365, 0.7153333333333342, 1.1486666666666674, -0.042074074074073264, -0.5105925925925918, -0.4217037037037029, 0.23570370370370441, 0.6857037037037044, 1.6782962962962968, 2.11162962962963, 1.937555555555556, 1.9745925925925931, 2.013481481481482, 1.3875555555555563, 1.067185185185186, 1.467185185185186, 0.6357037037037045, -0.2883703703703696, -0.23837037037036957, -1.332814814814814, -1.295777777777777, -1.1161481481481474, -0.8365185185185178, -0.30318518518518445, 0.13385185185185267, 1.143111111111112, 0.8986666666666676, 1.7745925925925934, 1.0968148148148158, 1.228296296296297, 0.628296296296297, 0.037555555555556175, 0.178296296296297, -1.160592592592592, -0.1865185185185178, -0.6346666666666658, -0.582814814814814, 0.9208888888888895, 0.9134814814814822, 1.3949629629629636, 1.137555555555556, -0.1531851851851843, -0.956888888888888, -1.2772592592592584, -0.5865185185185178, 0.4653333333333341, 0.4653333333333341, 0.3653333333333342, -0.019851851851851066, -1.2531851851851843, -0.8365185185185177, -1.1791111111111103, -0.5531851851851843, 0.48200000000000076, 0.1931111111111119, 1.3560740740740749, 1.254222222222223, 0.20051851851851932]
  out "On-Line Bin Readings 2":dbl[](array[numeric])=[3592.0, 538.0, 475.0, 472.0, 501.0, 508.0, 483.0, 476.0, 494.0, 546.0, 543.0, 505.0, 531.0, 525.0, 520.0, 503.0, 503.0, 503.0, 553.0, 489.0, 527.0, 520.0, 575.0, 550.0, 570.0, 561.0, 574.0, 621.0, 579.0, 532.0, 619.0, 596.0, 578.0, 630.0, 637.0, 629.0, 623.0, 646.0, 578.0, 612.0, 609.0, 642.0, 540.0, 589.0, 622.0, 582.0, 625.0, 608.0, 596.0, 609.0, 616.0, 621.0, 607.0, 606.0, 623.0, 615.0, 575.0, 637.0, 610.0, 600.0, 592.0, 584.0, 581.0, 575.0, 586.0, 573.0, 594.0, 578.0, 585.0, 609.0, 613.0, 603.0, 589.0, 562.0, 585.0, 590.0, 590.0, 578.0, 523.0, 540.0, 573.0, 561.0, 548.0, 548.0, 540.0, 494.0, 507.0, 518.0, 549.0, 540.0, 513.0, 531.0, 567.0, 541.0, 541.0, 548.0, 543.0, 503.0, 566.0, 538.0, 518.0, 499.0, 539.0, 511.0, 541.0, 518.0, 492.0, 570.0, 498.0, 501.0, 477.0, 510.0, 531.0, 512.0, 512.0, 531.0, 499.0, 489.0, 559.0, 519.0, 492.0, 496.0, 536.0, 522.0, 518.0, 525.0, 498.0, 510.0, 496.0, 515.0, 512.0, 518.0, 485.0, 520.0, 514.0, 542.0, 535.0, 457.0, 505.0, 503.0, 484.0, 489.0, 528.0, 511.0, 522.0, 501.0, 474.0, 522.0, 556.0, 507.0, 467.0, 516.0, 522.0, 509.0, 480.0, 499.0, 499.0, 520.0, 487.0, 522.0, 532.0, 510.0, 486.0, 488.0, 499.0, 473.0, 510.0, 489.0, 502.0, 479.0, 495.0, 493.0, 458.0, 517.0, 495.0, 546.0, 475.0, 463.0, 494.0, 495.0, 493.0, 505.0, 503.0, 511.0, 494.0, 489.0, 470.0, 481.0, 446.0, 501.0, 492.0, 471.0, 477.0, 506.0, 511.0, 451.0, 505.0, 449.0, 534.0, 501.0, 475.0, 539.0, 476.0, 502.0, 480.0, 510.0, 462.0, 501.0, 484.0, 520.0, 469.0, 461.0, 447.0, 478.0, 487.0, 496.0, 480.0, 478.0, 487.0, 484.0, 452.0, 483.0, 495.0, 473.0, 531.0, 484.0, 486.0, 495.0, 493.0, 522.0, 482.0, 480.0, 508.0, 479.0, 514.0, 470.0, 499.0, 459.0, 461.0, 481.0, 469.0, 511.0, 493.0, 491.0, 495.0, 495.0, 482.0, 493.0, 532.0, 503.0, 484.0, 491.0, 503.0, 500.0, 491.0, 468.0, 488.0, 458.0, 506.0, 501.0, 507.0, 486.0, 510.0, 515.0, 464.0, 496.0, 506.0, 480.0, 470.0, 498.0, 473.0, 495.0, 490.0, 449.0, 496.0, 481.0, 460.0, 464.0, 520.0, 464.0, 488.0, 458.0, 515.0, 498.0, 471.0, 511.0, 475.0, 476.0, 468.0, 452.0, 502.0, 498.0, 472.0, 452.0, 496.0, 456.0, 461.0, 500.0, 493.0, 468.0, 487.0, 502.0, 509.0, 509.0, 477.0, 456.0, 451.0, 520.0, 498.0, 469.0, 479.0, 515.0, 466.0, 520.0, 462.0, 454.0, 506.0, 473.0, 492.0, 508.0, 507.0, 478.0, 456.0, 500.0, 501.0, 513.0, 508.0, 507.0, 497.0, 431.0, 463.0, 489.0, 496.0, 477.0, 441.0, 451.0, 509.0, 519.0, 448.0, 473.0, 525.0, 479.0, 465.0, 498.0, 458.0, 508.0, 464.0, 472.0, 475.0, 503.0, 479.0, 464.0, 483.0, 484.0, 511.0, 481.0, 462.0, 474.0, 476.0, 466.0, 496.0, 502.0, 510.0, 502.0, 502.0, 480.0, 489.0, 475.0, 455.0, 518.0, 520.0, 469.0, 490.0, 458.0, 498.0, 486.0, 483.0, 454.0, 464.0, 460.0, 472.0, 481.0, 488.0, 445.0, 453.0, 480.0, 519.0, 512.0, 485.0, 472.0, 480.0, 494.0, 482.0, 457.0, 526.0, 470.0, 485.0, 452.0, 497.0, 521.0, 480.0, 510.0, 467.0, 477.0, 520.0, 497.0, 496.0, 492.0, 442.0, 473.0, 505.0, 459.0, 491.0, 466.0, 475.0, 481.0, 470.0, 485.0, 462.0, 492.0, 475.0, 515.0, 491.0, 460.0, 513.0, 494.0, 472.0, 461.0, 495.0, 480.0, 496.0, 505.0, 496.0, 476.0, 487.0, 480.0, 505.0, 501.0, 472.0, 476.0, 461.0, 487.0, 467.0, 478.0, 463.0, 499.0, 466.0, 519.0, 497.0, 486.0, 454.0, 470.0, 516.0, 476.0, 459.0, 492.0, 501.0, 498.0, 477.0, 442.0, 465.0, 444.0, 487.0, 455.0, 450.0, 500.0, 497.0, 498.0, 473.0, 496.0, 503.0, 500.0, 494.0, 484.0, 460.0, 492.0, 486.0, 477.0, 484.0, 469.0, 511.0, 474.0, 494.0, 462.0, 474.0, 511.0, 504.0, 481.0, 476.0, 510.0, 485.0, 457.0, 510.0, 483.0, 507.0, 438.0, 438.0, 462.0, 505.0, 492.0, 486.0, 496.0, 479.0, 467.0, 477.0, 481.0, 488.0, 462.0, 435.0, 462.0, 501.0, 468.0, 495.0, 457.0, 468.0, 463.0, 506.0, 476.0, 503.0, 456.0, 421.0, 479.0, 478.0, 465.0, 449.0, 483.0, 471.0, 493.0, 511.0, 491.0, 551.0, 488.0, 463.0, 458.0, 477.0, 504.0, 484.0, 472.0, 463.0, 532.0, 439.0, 481.0, 490.0, 440.0, 484.0, 504.0, 459.0, 505.0, 526.0, 497.0, 468.0, 482.0, 516.0, 434.0, 477.0, 488.0, 478.0, 478.0, 500.0]
  in  "stop":bool
  in  "Reset Average":bool=TRUE
  in  "Save Data?":bool=TRUE
  in  "Collect Data?":bool=TRUE
  in  "ILX Address":i32=6 min=0 step=1
  in  "Lambda On DBR Current":dbl=171.13999999999868
  in  "Lambda Off DBR Current":dbl=172.9499999999997
  in  "Tab Control":T2(tab)=enum."NRB"
  out "NRB plot":cluster{"Y":dbl[], "Y":dbl[]}[](graph)=[{"Y"=[0.0, 0.0, 0.0, 0.0, 0.0, 0.0, 0.0, 0.0, 0.0, 0.0, 0.0, 0.0, 0.0, 0.0, 0.0, 0.0, 0.0, 0.0, 0.0, 0.0, 0.0, 0.0, 0.0, 0.0, 0.0, 0.0, 0.0, 0.0, 0.0, 0.0, 0.0, 0.0, 0.0, 0.0, 0.0, 0.0, 0.0, 0.0, 0.0, 0.0, 0.0, 0.0, 0.0, 0.0, 0.0, 0.0, 0.0, 0.0, 0.0, 0.0, 0.0, 0.0, 0.0, 0.0, 0.0, 0.0, 0.0, 0.0, 0.0, 0.0, 0.0, 0.0, 0.0, 0.0, 0.0, 0.0, 0.0, 0.0, 0.0, 0.0, 0.0, 0.0, 0.0, 0.0, 0.0, 0.0, 0.0, 0.0, 0.0, 0.0, 0.0, 0.0, 0.0, 0.0, 0.0, 0.0, 0.0, 0.0, 0.0, 0.0, 0.0, 0.0, 0.0, 0.0, 0.0, 0.0, 0.0, 0.0, 0.0, 0.0, 0.0, 0.0, 0.0, 0.0, 0.0, 0.0, 0.0, 0.0, 0.0, 0.0, 0.0, 0.0, 0.0, 0.0, 0.0, 0.0, 0.0, 0.0, 0.0, 0.0, 0.0, 0.0, 0.0, 0.0, 0.0, 0.0, 0.0, 0.0, 0.0, 0.0, 0.0, 0.0, 0.0, 0.0, 0.0, 0.0, 0.0, 0.0, 0.0, 0.0, 0.0, 0.0, 0.0, 0.0, 0.0, 0.0, 0.0, 0.0, 0.0, 0.0, 0.0, 0.0, 0.0, 0.0, 0.0, 0.0, 0.0, 0.0, 0.0, 0.0, 0.0, 0.0, 0.0, 0.0, 0.0, 0.0, 0.0, 0.0, 0.0, 0.0, 0.0, 0.0, 0.0, 0.0, 0.0, 0.0, 0.0, 0.0, 0.0, 0.0, 0.0, 0.0, 0.0, 0.0, 0.0, 0.0, 0.0, 0.0, 0.0, 0.0, 0.0, 0.0, 0.0, 0.0, 0.0, 0.0, 0.0, 0.0, 0.0, 0.0, 0.0, 0.0, 0.0, 0.0, 0.0, 0.0, 0.0, 0.0, 0.0, 0.0, 0.0, 0.0, 0.0, 0.0, 0.0, 0.0, 0.0, 0.0, 0.0, 0.0, 0.0, 0.0, 0.0, 0.0, 0.0, 0.0, 0.0, 0.0, 0.0, 0.0, 0.0, 0.0, 0.0, 0.0, 0.0, 0.0, 0.0, 0.0, 0.0, 0.0, 0.0, 0.0, 0.0, 0.0, 0.0, 0.0, 0.0, 0.0, 0.0, 0.0, 0.0, 0.0, 0.0, 0.0, 0.0, 0.0, 0.0, 0.0, 0.0, 0.0, 0.0, 0.0, 0.0, 0.0, 0.0, 0.0, 0.0, 0.0, 0.0, 0.0, 0.0, 0.0, 0.0, 0.0, 0.0, 0.0, 0.0, 0.0, 0.0, 0.0, 0.0, 0.0, 0.0, 0.0, 0.0, 0.0, 0.0, 0.0, 0.0, 0.0, 0.0, 0.0, 0.0, 0.0, 0.0, 0.0, 0.0, 0.0, 0.0, 0.0, 0.0, 0.0, 0.0, 0.0, 0.0, 0.0, 0.0, 0.0, 0.0, 0.0, 0.0, 0.0, 0.0, 0.0, 0.0, 0.0, 0.0, 0.0, 0.0, 0.0, 0.0, 0.0, 0.0, 0.0, 0.0, 0.0, 0.0, 0.0, 0.0, 0.0, 0.0, 0.0, 0.0, 0.0, 0.0, 0.0, 0.0, 0.0, 0.0, 0.0, 0.0, 0.0, 0.0, 0.0, 0.0, 0.0, 0.0, 0.0, 0.0, 0.0, 0.0, 0.0, 0.0, 0.0, 0.0, 0.0, 0.0, 0.0, 0.0, 0.0, 0.0, 0.0, 0.0, 0.0, 0.0, 0.0, 0.0, 0.0, 0.0, 0.0, 0.0, 0.0, 0.0, 0.0, 0.0, 0.0, 0.0, 0.0, 0.0, 0.0, 0.0, 0.0, 0.0, 0.0, 0.0, 0.0, 0.0, 0.0, 0.0, 0.0, 0.0, 0.0, 0.0, 0.0, 0.0, 0.0, 0.0, 0.0, 0.0, 0.0, 0.0, 0.0, 0.0, 0.0, 0.0, 0.0, 0.0, 0.0, 0.0, 0.0, 0.0, 0.0, 0.0, 0.0, 0.0, 0.0, 0.0, 0.0, 0.0, 0.0, 0.0, 0.0, 0.0, 0.0, 0.0, 0.0, 0.0, 0.0, 0.0, 0.0, 0.0, 0.0, 0.0, 0.0, 0.0, 0.0, 0.0, 0.0, 0.0, 0.0, 0.0, 0.0, 0.0, 0.0, 0.0, 0.0, 0.0, 0.0, 0.0, 0.0, 0.0, 0.0, 0.0, 0.0, 0.0, 0.0, 0.0, 0.0, 0.0, 0.0, 0.0, 0.0, 0.0, 0.0, 0.0, 0.0, 0.0, 0.0, 0.0, 0.0, 0.0, 0.0, 0.0, 0.0, 0.0, 0.0, 0.0, 0.0, 0.0, 0.0, 0.0, 0.0, 0.0, 0.0, 0.0, 0.0, 0.0, 0.0, 0.0, 0.0, 0.0, 0.0, 0.0, 0.0, 0.0, 0.0, 0.0, 0.0, 0.0, 0.0, 0.0, 0.0, 0.0, 0.0, 0.0, 0.0, 0.0, 0.0, 0.0, 0.0, 0.0, 0.0, 0.0, 0.0, 0.0, 0.0, 0.0, 0.0, 0.0, 0.0, 0.0, 0.0, 0.0, 0.0, 0.0, 0.0, 0.0, 0.0, 0.0, 0.0, 0.0, 0.0, 0.0, 0.0, 0.0, 0.0, 0.0, 0.0, 0.0, 0.0, 0.0, 0.0, 0.0, 0.0, 0.0, 0.0, 0.0, 0.0, 0.0, 0.0, 0.0, 0.0, 0.0, 0.0, 0.0], "Y"=[0.0375, 0.075, 0.11249999999999999, 0.15, 0.1875, 0.225, 0.26249999999999996, 0.3, 0.33749999999999997, 0.37499999999999994, 0.4125, 0.44999999999999996, 0.48749999999999993, 0.525, 0.5625, 0.6, 0.6375, 0.6749999999999999, 0.7124999999999999, 0.75, 0.7875, 0.825, 0.8624999999999999, 0.8999999999999999, 0.9374999999999999, 0.975, 1.0125, 1.05, 1.0875000000000001, 1.125, 1.1625, 1.2, 1.2375, 1.2750000000000001, 1.3125, 1.35, 1.3875, 1.425, 1.4625000000000001, 1.5, 1.5375, 1.575, 1.6125, 1.6500000000000001, 1.6875, 1.725, 1.7625, 1.8, 1.8375, 1.875, 1.9125, 1.95, 1.9875, 2.025, 2.0625, 2.1, 2.1375, 2.175, 2.2125, 2.25, 2.2875, 2.325, 2.3625, 2.4, 2.4375, 2.475, 2.5125, 2.55, 2.5875, 2.625, 2.6625, 2.7, 2.7375, 2.775, 2.8125, 2.85, 2.8875, 2.925, 2.9625, 3.0, 3.0375, 3.075, 3.1125, 3.15, 3.1875, 3.225, 3.2625, 3.3, 3.3375, 3.375, 3.4125, 3.45, 3.4875, 3.525, 3.5625, 3.6, 3.6374999999999997, 3.675, 3.7125, 3.75, 3.7875, 3.8249999999999997, 3.8625, 3.9, 3.9375, 3.975, 4.012499999999999, 4.05, 4.0874999999999995, 4.124999999999999, 4.1625, 4.199999999999999, 4.2375, 4.2749999999999995, 4.312499999999999, 4.35, 4.387499999999999, 4.425, 4.4624999999999995, 4.499999999999999, 4.5375, 4.574999999999999, 4.6125, 4.6499999999999995, 4.687499999999999, 4.725, 4.762499999999999, 4.8, 4.8374999999999995, 4.874999999999999, 4.9125, 4.949999999999999, 4.9875, 5.0249999999999995, 5.062499999999999, 5.1, 5.137499999999999, 5.175, 5.2124999999999995, 5.249999999999999, 5.2875, 5.324999999999999, 5.3625, 5.3999999999999995, 5.437499999999999, 5.475, 5.512499999999999, 5.55, 5.5874999999999995, 5.624999999999999, 5.6625, 5.699999999999999, 5.7375, 5.7749999999999995, 5.812499999999999, 5.85, 5.887499999999999, 5.925, 5.9624999999999995, 5.999999999999999, 6.0375, 6.074999999999999, 6.1125, 6.1499999999999995, 6.187499999999999, 6.225, 6.262499999999999, 6.3, 6.3374999999999995, 6.374999999999999, 6.4125, 6.449999999999999, 6.4875, 6.5249999999999995, 6.562499999999999, 6.6, 6.637499999999999, 6.675, 6.7124999999999995, 6.749999999999999, 6.7875, 6.824999999999999, 6.8625, 6.8999999999999995, 6.937499999999999, 6.975, 7.012499999999999, 7.05, 7.0874999999999995, 7.124999999999999, 7.1625, 7.199999999999999, 7.237499999999999, 7.2749999999999995, 7.312499999999999, 7.35, 7.387499999999999, 7.424999999999999, 7.4624999999999995, 7.499999999999999, 7.5375, 7.574999999999999, 7.612499999999999, 7.6499999999999995, 7.687499999999999, 7.725, 7.762499999999999, 7.799999999999999, 7.8374999999999995, 7.874999999999999, 7.9125, 7.949999999999999, 7.987499999999999, 8.025, 8.0625, 8.1, 8.1375, 8.174999999999999, 8.212499999999999, 8.25, 8.2875, 8.325, 8.362499999999999, 8.399999999999999, 8.4375, 8.475, 8.5125, 8.549999999999999, 8.587499999999999, 8.625, 8.6625, 8.7, 8.737499999999999, 8.774999999999999, 8.8125, 8.85, 8.8875, 8.924999999999999, 8.962499999999999, 9.0, 9.0375, 9.075, 9.112499999999999, 9.149999999999999, 9.1875, 9.225, 9.2625, 9.299999999999999, 9.337499999999999, 9.375, 9.4125, 9.45, 9.487499999999999, 9.524999999999999, 9.5625, 9.6, 9.6375, 9.674999999999999, 9.712499999999999, 9.75, 9.7875, 9.825, 9.862499999999999, 9.899999999999999, 9.9375, 9.975, 10.0125, 10.049999999999999, 10.087499999999999, 10.125, 10.1625, 10.2, 10.237499999999999, 10.274999999999999, 10.3125, 10.35, 10.3875, 10.424999999999999, 10.462499999999999, 10.5, 10.5375, 10.575, 10.612499999999999, 10.649999999999999, 10.6875, 10.725, 10.7625, 10.799999999999999, 10.837499999999999, 10.875, 10.9125, 10.95, 10.987499999999999, 11.024999999999999, 11.0625, 11.1, 11.1375, 11.174999999999999, 11.212499999999999, 11.25, 11.2875, 11.325, 11.362499999999999, 11.399999999999999, 11.4375, 11.475, 11.5125, 11.549999999999999, 11.587499999999999, 11.625, 11.6625, 11.7, 11.737499999999999, 11.774999999999999, 11.8125, 11.85, 11.8875, 11.924999999999999, 11.962499999999999, 12.0, 12.0375, 12.075, 12.112499999999999, 12.149999999999999, 12.1875, 12.225, 12.2625, 12.299999999999999, 12.337499999999999, 12.375, 12.4125, 12.45, 12.487499999999999, 12.524999999999999, 12.5625, 12.6, 12.6375, 12.674999999999999, 12.712499999999999, 12.75, 12.7875, 12.825, 12.862499999999999, 12.899999999999999, 12.9375, 12.975, 13.0125, 13.049999999999999, 13.087499999999999, 13.125, 13.1625, 13.2, 13.237499999999999, 13.274999999999999, 13.3125, 13.35, 13.3875, 13.424999999999999, 13.462499999999999, 13.5, 13.5375, 13.575, 13.612499999999999, 13.649999999999999, 13.6875, 13.725, 13.7625, 13.799999999999999, 13.837499999999999, 13.875, 13.9125, 13.95, 13.987499999999999, 14.024999999999999, 14.0625, 14.1, 14.1375, 14.174999999999999, 14.212499999999999, 14.25, 14.2875, 14.325, 14.362499999999999, 14.399999999999999, 14.437499999999998, 14.475, 14.5125, 14.549999999999999, 14.587499999999999, 14.624999999999998, 14.6625, 14.7, 14.737499999999999, 14.774999999999999, 14.812499999999998, 14.85, 14.8875, 14.924999999999999, 14.962499999999999, 14.999999999999998, 15.0375, 15.075, 15.112499999999999, 15.149999999999999, 15.187499999999998, 15.225, 15.2625, 15.299999999999999, 15.337499999999999, 15.374999999999998, 15.4125, 15.45, 15.487499999999999, 15.524999999999999, 15.562499999999998, 15.6, 15.6375, 15.674999999999999, 15.712499999999999, 15.749999999999998, 15.7875, 15.825, 15.862499999999999, 15.899999999999999, 15.937499999999998, 15.975, 16.0125, 16.05, 16.087500000000002, 16.125, 16.1625, 16.2, 16.2375, 16.275000000000002, 16.3125, 16.35, 16.3875, 16.425, 16.462500000000002, 16.5, 16.5375, 16.575, 16.6125, 16.650000000000002, 16.6875, 16.725, 16.7625, 16.8, 16.837500000000002, 16.875, 16.9125, 16.95, 16.9875, 17.025000000000002, 17.0625, 17.1, 17.1375, 17.175, 17.212500000000002, 17.25, 17.2875, 17.325, 17.3625, 17.400000000000002, 17.4375, 17.475, 17.5125, 17.55, 17.587500000000002, 17.625, 17.6625, 17.7, 17.7375, 17.775000000000002, 17.8125, 17.85, 17.8875, 17.925, 17.962500000000002, 18.0, 18.0375, 18.075, 18.1125, 18.150000000000002, 18.1875, 18.225, 18.2625, 18.3, 18.337500000000002, 18.375, 18.4125, 18.45, 18.4875, 18.525000000000002, 18.5625, 18.6, 18.6375, 18.675, 18.712500000000002, 18.75, 18.7875, 18.825, 18.8625, 18.900000000000002, 18.9375, 18.975, 19.0125, 19.05, 19.087500000000002, 19.125, 19.1625, 19.2, 19.2375, 19.275000000000002, 19.3125, 19.35, 19.3875, 19.425, 19.462500000000002, 19.5, 19.5375, 19.575, 19.6125, 19.650000000000002, 19.6875, 19.725, 19.7625, 19.8, 19.837500000000002, 19.875, 19.9125, 19.95, 19.9875, 20.025000000000002, 20.0625, 20.1, 20.1375, 20.175, 20.212500000000002, 20.25, 20.2875, 20.325, 20.3625, 20.400000000000002, 20.4375, 20.475, 20.5125, 20.55, 20.587500000000002, 20.625, 20.6625, 20.7, 20.7375, 20.775000000000002, 20.8125, 20.85, 20.8875, 20.925, 20.962500000000002, 21.0]}, ...(2 in all)]
  in  "background length":i32=25
  out "Correction":cluster{"Y":dbl[], "Y":dbl[]}[](graph)=[{"Y"=[1.0, 1.0, 1.0, 1.0, 1.0, 1.0, 1.0, 1.0, 1.0, 1.0, 1.0, 1.0, 1.0, 1.0, 1.0, 1.0, 1.0, 1.0, 1.0, 1.0, 1.0, 1.0, 1.0, 1.0, 1.0, 1.0, 1.0, 1.0, 1.0, 1.0, 1.0, 1.0, 1.0, 1.0, 1.0, 1.0, 1.0, 1.0, 1.0, 1.0, 1.0, 1.0, 1.0, 1.0, 1.0, 1.0, 1.0, 1.0, 1.0, 1.0, 1.0, 1.0, 1.0, 1.0, 1.0, 1.0, 1.0, 1.0, 1.0, 1.0, 1.0, 1.0, 1.0, 1.0, 1.0, 1.0, 1.0, 1.0, 1.0, 1.0, 1.0, 1.0, 1.0, 1.0, 1.0, 1.0, 1.0, 1.0, 1.0, 1.0, 1.0, 1.0, 1.0, 1.0, 1.0, 1.0, 1.0, 1.0, 1.0, 1.0, 1.0, 1.0, 1.0, 1.0, 1.0, 1.0, 1.0, 1.0, 1.0, 1.0, 1.0, 1.0, 1.0, 1.0, 1.0, 1.0, 1.0, 1.0, 1.0, 1.0, 1.0, 1.0, 1.0, 1.0, 1.0, 1.0, 1.0, 1.0, 1.0, 1.0, 1.0, 1.0, 1.0, 1.0, 1.0, 1.0, 1.0, 1.0, 1.0, 1.0, 1.0, 1.0, 1.0, 1.0, 1.0, 1.0, 1.0, 1.0, 1.0, 1.0, 1.0, 1.0, 1.0, 1.0, 1.0, 1.0, 1.0, 1.0, 1.0, 1.0, 1.0, 1.0, 1.0, 1.0, 1.0, 1.0, 1.0, 1.0, 1.0, 1.0, 1.0, 1.0, 1.0, 1.0, 1.0, 1.0, 1.0, 1.0, 1.0, 1.0, 1.0, 1.0, 1.0, 1.0, 1.0, 1.0, 1.0, 1.0, 1.0, 1.0, 1.0, 1.0, 1.0, 1.0, 1.0, 1.0, 1.0, 1.0, 1.0, 1.0, 1.0, 1.0, 1.0, 1.0, 1.0, 1.0, 1.0, 1.0, 1.0, 1.0, 1.0, 1.0, 1.0, 1.0, 1.0, 1.0, 1.0, 1.0, 1.0, 1.0, 1.0, 1.0, 1.0, 1.0, 1.0, 1.0, 1.0, 1.0, 1.0, 1.0, 1.0, 1.0, 1.0, 1.0, 1.0, 1.0, 1.0, 1.0, 1.0, 1.0, 1.0, 1.0, 1.0, 1.0, 1.0, 1.0, 1.0, 1.0, 1.0, 1.0, 1.0, 1.0, 1.0, 1.0, 1.0, 1.0, 1.0, 1.0, 1.0, 1.0, 1.0, 1.0, 1.0, 1.0, 1.0, 1.0, 1.0, 1.0, 1.0, 1.0, 1.0, 1.0, 1.0, 1.0, 1.0, 1.0, 1.0, 1.0, 1.0, 1.0, 1.0, 1.0, 1.0, 1.0, 1.0, 1.0, 1.0, 1.0, 1.0, 1.0, 1.0, 1.0, 1.0, 1.0, 1.0, 1.0, 1.0, 1.0, 1.0, 1.0, 1.0, 1.0, 1.0, 1.0, 1.0, 1.0, 1.0, 1.0, 1.0, 1.0, 1.0, 1.0, 1.0, 1.0, 1.0, 1.0, 1.0, 1.0, 1.0, 1.0, 1.0, 1.0, 1.0, 1.0, 1.0, 1.0, 1.0, 1.0, 1.0, 1.0, 1.0, 1.0, 1.0, 1.0, 1.0, 1.0, 1.0, 1.0, 1.0, 1.0, 1.0, 1.0, 1.0, 1.0, 1.0, 1.0, 1.0, 1.0, 1.0, 1.0, 1.0, 1.0, 1.0, 1.0, 1.0, 1.0, 1.0, 1.0, 1.0, 1.0, 1.0, 1.0, 1.0, 1.0, 1.0, 1.0, 1.0, 1.0, 1.0, 1.0, 1.0, 1.0, 1.0, 1.0, 1.0, 1.0, 1.0, 1.0, 1.0, 1.0, 1.0, 1.0, 1.0, 1.0, 1.0, 1.0, 1.0, 1.0, 1.0, 1.0, 1.0, 1.0, 1.0, 1.0, 1.0, 1.0, 1.0, 1.0, 1.0, 1.0, 1.0, 1.0, 1.0, 1.0, 1.0, 1.0, 1.0, 1.0, 1.0, 1.0, 1.0, 1.0, 1.0, 1.0, 1.0, 1.0, 1.0, 1.0, 1.0, 1.0, 1.0, 1.0, 1.0, 1.0, 1.0, 1.0, 1.0, 1.0, 1.0, 1.0, 1.0, 1.0, 1.0, 1.0, 1.0, 1.0, 1.0, 1.0, 1.0, 1.0, 1.0, 1.0, 1.0, 1.0, 1.0, 1.0, 1.0, 1.0, 1.0, 1.0, 1.0, 1.0, 1.0, 1.0, 1.0, 1.0, 1.0, 1.0, 1.0, 1.0, 1.0, 1.0, 1.0, 1.0, 1.0, 1.0, 1.0, 1.0, 1.0, 1.0, 1.0, 1.0, 1.0, 1.0, 1.0, 1.0, 1.0, 1.0, 1.0, 1.0, 1.0, 1.0, 1.0, 1.0, 1.0, 1.0, 1.0, 1.0, 1.0, 1.0, 1.0, 1.0, 1.0, 1.0, 1.0, 1.0, 1.0, 1.0, 1.0, 1.0, 1.0, 1.0, 1.0, 1.0, 1.0, 1.0, 1.0, 1.0, 1.0, 1.0, 1.0, 1.0, 1.0, 1.0, 1.0, 1.0, 1.0, 1.0, 1.0, 1.0, 1.0, 1.0, 1.0, 1.0, 1.0, 1.0, 1.0, 1.0, 1.0, 1.0, 1.0, 1.0, 1.0, 1.0, 1.0, 1.0, 1.0, 1.0, 1.0, 1.0, 1.0, 1.0, 1.0, 1.0, 1.0, 1.0, 1.0, 1.0, 1.0, 1.0, 1.0, 1.0, 1.0, 1.0, 1.0, 1.0, 1.0, 1.0, 1.0, 1.0, 1.0, 1.0, 1.0, 1.0, 1.0], "Y"=[0.0375, 0.075, 0.11249999999999999, 0.15, 0.1875, 0.225, 0.26249999999999996, 0.3, 0.33749999999999997, 0.37499999999999994, 0.4125, 0.44999999999999996, 0.48749999999999993, 0.525, 0.5625, 0.6, 0.6375, 0.6749999999999999, 0.7124999999999999, 0.75, 0.7875, 0.825, 0.8624999999999999, 0.8999999999999999, 0.9374999999999999, 0.975, 1.0125, 1.05, 1.0875000000000001, 1.125, 1.1625, 1.2, 1.2375, 1.2750000000000001, 1.3125, 1.35, 1.3875, 1.425, 1.4625000000000001, 1.5, 1.5375, 1.575, 1.6125, 1.6500000000000001, 1.6875, 1.725, 1.7625, 1.8, 1.8375, 1.875, 1.9125, 1.95, 1.9875, 2.025, 2.0625, 2.1, 2.1375, 2.175, 2.2125, 2.25, 2.2875, 2.325, 2.3625, 2.4, 2.4375, 2.475, 2.5125, 2.55, 2.5875, 2.625, 2.6625, 2.7, 2.7375, 2.775, 2.8125, 2.85, 2.8875, 2.925, 2.9625, 3.0, 3.0375, 3.075, 3.1125, 3.15, 3.1875, 3.225, 3.2625, 3.3, 3.3375, 3.375, 3.4125, 3.45, 3.4875, 3.525, 3.5625, 3.6, 3.6374999999999997, 3.675, 3.7125, 3.75, 3.7875, 3.8249999999999997, 3.8625, 3.9, 3.9375, 3.975, 4.012499999999999, 4.05, 4.0874999999999995, 4.124999999999999, 4.1625, 4.199999999999999, 4.2375, 4.2749999999999995, 4.312499999999999, 4.35, 4.387499999999999, 4.425, 4.4624999999999995, 4.499999999999999, 4.5375, 4.574999999999999, 4.6125, 4.6499999999999995, 4.687499999999999, 4.725, 4.762499999999999, 4.8, 4.8374999999999995, 4.874999999999999, 4.9125, 4.949999999999999, 4.9875, 5.0249999999999995, 5.062499999999999, 5.1, 5.137499999999999, 5.175, 5.2124999999999995, 5.249999999999999, 5.2875, 5.324999999999999, 5.3625, 5.3999999999999995, 5.437499999999999, 5.475, 5.512499999999999, 5.55, 5.5874999999999995, 5.624999999999999, 5.6625, 5.699999999999999, 5.7375, 5.7749999999999995, 5.812499999999999, 5.85, 5.887499999999999, 5.925, 5.9624999999999995, 5.999999999999999, 6.0375, 6.074999999999999, 6.1125, 6.1499999999999995, 6.187499999999999, 6.225, 6.262499999999999, 6.3, 6.3374999999999995, 6.374999999999999, 6.4125, 6.449999999999999, 6.4875, 6.5249999999999995, 6.562499999999999, 6.6, 6.637499999999999, 6.675, 6.7124999999999995, 6.749999999999999, 6.7875, 6.824999999999999, 6.8625, 6.8999999999999995, 6.937499999999999, 6.975, 7.012499999999999, 7.05, 7.0874999999999995, 7.124999999999999, 7.1625, 7.199999999999999, 7.237499999999999, 7.2749999999999995, 7.312499999999999, 7.35, 7.387499999999999, 7.424999999999999, 7.4624999999999995, 7.499999999999999, 7.5375, 7.574999999999999, 7.612499999999999, 7.6499999999999995, 7.687499999999999, 7.725, 7.762499999999999, 7.799999999999999, 7.8374999999999995, 7.874999999999999, 7.9125, 7.949999999999999, 7.987499999999999, 8.025, 8.0625, 8.1, 8.1375, 8.174999999999999, 8.212499999999999, 8.25, 8.2875, 8.325, 8.362499999999999, 8.399999999999999, 8.4375, 8.475, 8.5125, 8.549999999999999, 8.587499999999999, 8.625, 8.6625, 8.7, 8.737499999999999, 8.774999999999999, 8.8125, 8.85, 8.8875, 8.924999999999999, 8.962499999999999, 9.0, 9.0375, 9.075, 9.112499999999999, 9.149999999999999, 9.1875, 9.225, 9.2625, 9.299999999999999, 9.337499999999999, 9.375, 9.4125, 9.45, 9.487499999999999, 9.524999999999999, 9.5625, 9.6, 9.6375, 9.674999999999999, 9.712499999999999, 9.75, 9.7875, 9.825, 9.862499999999999, 9.899999999999999, 9.9375, 9.975, 10.0125, 10.049999999999999, 10.087499999999999, 10.125, 10.1625, 10.2, 10.237499999999999, 10.274999999999999, 10.3125, 10.35, 10.3875, 10.424999999999999, 10.462499999999999, 10.5, 10.5375, 10.575, 10.612499999999999, 10.649999999999999, 10.6875, 10.725, 10.7625, 10.799999999999999, 10.837499999999999, 10.875, 10.9125, 10.95, 10.987499999999999, 11.024999999999999, 11.0625, 11.1, 11.1375, 11.174999999999999, 11.212499999999999, 11.25, 11.2875, 11.325, 11.362499999999999, 11.399999999999999, 11.4375, 11.475, 11.5125, 11.549999999999999, 11.587499999999999, 11.625, 11.6625, 11.7, 11.737499999999999, 11.774999999999999, 11.8125, 11.85, 11.8875, 11.924999999999999, 11.962499999999999, 12.0, 12.0375, 12.075, 12.112499999999999, 12.149999999999999, 12.1875, 12.225, 12.2625, 12.299999999999999, 12.337499999999999, 12.375, 12.4125, 12.45, 12.487499999999999, 12.524999999999999, 12.5625, 12.6, 12.6375, 12.674999999999999, 12.712499999999999, 12.75, 12.7875, 12.825, 12.862499999999999, 12.899999999999999, 12.9375, 12.975, 13.0125, 13.049999999999999, 13.087499999999999, 13.125, 13.1625, 13.2, 13.237499999999999, 13.274999999999999, 13.3125, 13.35, 13.3875, 13.424999999999999, 13.462499999999999, 13.5, 13.5375, 13.575, 13.612499999999999, 13.649999999999999, 13.6875, 13.725, 13.7625, 13.799999999999999, 13.837499999999999, 13.875, 13.9125, 13.95, 13.987499999999999, 14.024999999999999, 14.0625, 14.1, 14.1375, 14.174999999999999, 14.212499999999999, 14.25, 14.2875, 14.325, 14.362499999999999, 14.399999999999999, 14.437499999999998, 14.475, 14.5125, 14.549999999999999, 14.587499999999999, 14.624999999999998, 14.6625, 14.7, 14.737499999999999, 14.774999999999999, 14.812499999999998, 14.85, 14.8875, 14.924999999999999, 14.962499999999999, 14.999999999999998, 15.0375, 15.075, 15.112499999999999, 15.149999999999999, 15.187499999999998, 15.225, 15.2625, 15.299999999999999, 15.337499999999999, 15.374999999999998, 15.4125, 15.45, 15.487499999999999, 15.524999999999999, 15.562499999999998, 15.6, 15.6375, 15.674999999999999, 15.712499999999999, 15.749999999999998, 15.7875, 15.825, 15.862499999999999, 15.899999999999999, 15.937499999999998, 15.975, 16.0125, 16.05, 16.087500000000002, 16.125, 16.1625, 16.2, 16.2375, 16.275000000000002, 16.3125, 16.35, 16.3875, 16.425, 16.462500000000002, 16.5, 16.5375, 16.575, 16.6125, 16.650000000000002, 16.6875, 16.725, 16.7625, 16.8, 16.837500000000002, 16.875, 16.9125, 16.95, 16.9875, 17.025000000000002, 17.0625, 17.1, 17.1375, 17.175, 17.212500000000002, 17.25, 17.2875, 17.325, 17.3625, 17.400000000000002, 17.4375, 17.475, 17.5125, 17.55, 17.587500000000002, 17.625, 17.6625, 17.7, 17.7375, 17.775000000000002, 17.8125, 17.85, 17.8875, 17.925, 17.962500000000002, 18.0, 18.0375, 18.075, 18.1125, 18.150000000000002, 18.1875, 18.225, 18.2625, 18.3, 18.337500000000002, 18.375, 18.4125, 18.45, 18.4875, 18.525000000000002, 18.5625, 18.6, 18.6375, 18.675, 18.712500000000002, 18.75, 18.7875, 18.825, 18.8625, 18.900000000000002, 18.9375, 18.975, 19.0125, 19.05, 19.087500000000002, 19.125, 19.1625, 19.2, 19.2375, 19.275000000000002, 19.3125, 19.35, 19.3875, 19.425, 19.462500000000002, 19.5, 19.5375, 19.575, 19.6125, 19.650000000000002, 19.6875, 19.725, 19.7625, 19.8, 19.837500000000002, 19.875, 19.9125, 19.95, 19.9875, 20.025000000000002, 20.0625, 20.1, 20.1375, 20.175, 20.212500000000002, 20.25, 20.2875, 20.325, 20.3625, 20.400000000000002, 20.4375, 20.475, 20.5125, 20.55, 20.587500000000002, 20.625, 20.6625, 20.7, 20.7375, 20.775000000000002, 20.8125, 20.85, 20.8875, 20.925, 20.962500000000002, 21.0]}, ...(2 in all)]
  in  "dead time":dbl=3.7e-08
  out "RingBuffer offline far":dbl[][](array[numeric])
  out "RingBuffer aerosol far":dbl[][](array[numeric])
  in  "Weather":T3(tab)=enum."Background (Mc/s)"
  out "Temperature (C)":dbl(graph)=10.05173992673992
  out "Pressure (mb)":dbl(graph)=844.793956043956
  out "Relative Humdity (%)":dbl(graph)=16.25915750915751
  out "Pulse Energy (Micro Joule)":T4(graph)={"Online Pulse Energy"=0.01695981714285714, "Pulse Energy Offline"=0.016990764285714284}
  out "?":cluster{"mean":dbl, "mean":dbl}(graph)={"mean"=0.0, "mean"=74371.71858592931}
  out "Index":i32=315
  out "Aerosol Smoothed":dbl[](array[numeric])
  out "Off-Line  Bin Readings":dbl[](array[numeric])
  out "Off-Line Smoothed":dbl[](array[numeric])
  out "On-Line  Smoothed":dbl[](array[numeric])
  out "On-Line Bin Readings":dbl[](array[numeric])
  out "Range Corrected Altitude Array":dbl[](array[numeric])=[1406.25, 5625.0, 12656.25, 22500.0, 35156.25, 50625.0, 68906.25, 90000.0, 113906.25, 140625.0, 170156.25, 202500.0, 237656.25, 275625.0, 316406.25, 360000.0, 406406.25, 455625.0, 507656.25, 562500.0, 620156.25, 680625.0, 743906.25, 810000.0, 878906.25, 950625.0, 1025156.25, 1102500.0, 1182656.25, 1265625.0, 1351406.25, 1440000.0, 1531406.25, 1625625.0, 1722656.25, 1822500.0, 1925156.25, 2030625.0, 2138906.25, 2250000.0, 2363906.25, 2480625.0, 2600156.25, 2722500.0, 2847656.25, 2975625.0, 3106406.25, 3240000.0, 3376406.25, 3515625.0, 3657656.25, 3802500.0, 3950156.25, 4100625.0, 4253906.25, 4410000.0, 4568906.25, 4730625.0, 4895156.25, 5062500.0, 5232656.25, 5405625.0, 5581406.25, 5760000.0, 5941406.25, 6125625.0, 6312656.25, 6502500.0, 6695156.25, 6890625.0, 7088906.25, 7290000.0, 7493906.25, 7700625.0, 7910156.25, 8122500.0, 8337656.25, 8555625.0, 8776406.25, 9000000.0, 9226406.25, 9455625.0, 9687656.25, 9922500.0, 10160156.25, 10400625.0, 10643906.25, 10890000.0, 11138906.25, 11390625.0, 11645156.25, 11902500.0, 12162656.25, 12425625.0, 12691406.25, 12960000.0, 13231406.25, 13505625.0, 13782656.25, 14062500.0, 14345156.25, 14630625.0, 14918906.25, 15210000.0, 15503906.25, 15800625.0, 16100156.25, 16402500.0, 16707656.25, 17015625.0, 17326406.25, 17640000.0, 17956406.25, 18275625.0, 18597656.25, 18922500.0, 19250156.25, 19580625.0, 19913906.25, 20250000.0, 20588906.25, 20930625.0, 21275156.25, 21622500.0, 21972656.25, 22325625.0, 22681406.25, 23040000.0, 23401406.25, 23765625.0, 24132656.25, 24502500.0, 24875156.25, 25250625.0, 25628906.25, 26010000.0, 26393906.25, 26780625.0, 27170156.25, 27562500.0, 27957656.25, 28355625.0, 28756406.25, 29160000.0, 29566406.25, 29975625.0, 30387656.25, 30802500.0, 31220156.25, 31640625.0, 32063906.25, 32490000.0, 32918906.25, 33350625.0, 33785156.25, 34222500.0, 34662656.25, 35105625.0, 35551406.25, 36000000.0, 36451406.25, 36905625.0, 37362656.25, 37822500.0, 38285156.25, 38750625.0, 39218906.25, 39690000.0, 40163906.25, 40640625.0, 41120156.25, 41602500.0, 42087656.25, 42575625.0, 43066406.25, 43560000.0, 44056406.25, 44555625.0, 45057656.25, 45562500.0, 46070156.25, 46580625.0, 47093906.25, 47610000.0, 48128906.25, 48650625.0, 49175156.25, 49702500.0, 50232656.25, 50765625.0, 51301406.25, 51840000.0, 52381406.25, 52925625.0, 53472656.25, 54022500.0, 54575156.25, 55130625.0, 55688906.25, 56250000.0, 56813906.25, 57380625.0, 57950156.25, 58522500.0, 59097656.25, 59675625.0, 60256406.25, 60840000.0, 61426406.25, 62015625.0, 62607656.25, 63202500.0, 63800156.25, 64400625.0, 65003906.25, 65610000.0, 66218906.25, 66830625.0, 67445156.25, 68062500.0, 68682656.25, 69305625.0, 69931406.25, 70560000.0, 71191406.25, 71825625.0, 72462656.25, 73102500.0, 73745156.25, 74390625.0, 75038906.25, 75690000.0, 76343906.25, 77000625.0, 77660156.25, 78322500.0, 78987656.25, 79655625.0, 80326406.25, 81000000.0, 81676406.25, 82355625.0, 83037656.25, 83722500.0, 84410156.25, 85100625.0, 85793906.25, 86490000.0, 87188906.25, 87890625.0, 88595156.25, 89302500.0, 90012656.25, 90725625.0, 91441406.25, 92160000.0, 92881406.25, 93605625.0, 94332656.25, 95062500.0, 95795156.25, 96530625.0, 97268906.25, 98010000.0, 98753906.25, 99500625.0, 100250156.25, 101002500.0, 101757656.25, 102515625.0, 103276406.25, 104040000.0, 104806406.25, 105575625.0, 106347656.25, 107122500.0, 107900156.25, 108680625.0, 109463906.25, 110250000.0, 111038906.25, 111830625.0, 112625156.25, 113422500.0, 114222656.25, 115025625.0, 115831406.25, 116640000.0, 117451406.25, 118265625.0, 119082656.25, 119902500.0, 120725156.25, 121550625.0, 122378906.25, 123210000.0, 124043906.25, 124880625.0, 125720156.25, 126562500.0, 127407656.25, 128255625.0, 129106406.25, 129960000.0, 130816406.25, 131675625.0, 132537656.25, 133402500.0, 134270156.25, 135140625.0, 136013906.25, 136890000.0, 137768906.25, 138650625.0, 139535156.25, 140422500.0, 141312656.25, 142205625.0, 143101406.25, 144000000.0, 144901406.25, 145805625.0, 146712656.25, 147622500.0, 148535156.25, 149450625.0, 150368906.25, 151290000.0, 152213906.25, 153140625.0, 154070156.25, 155002500.0, 155937656.25, 156875625.0, 157816406.25, 158760000.0, 159706406.25, 160655625.0, 161607656.25, 162562500.0, 163520156.25, 164480625.0, 165443906.25, 166410000.0, 167378906.25, 168350625.0, 169325156.25, 170302500.0, 171282656.25, 172265625.0, 173251406.25, 174240000.0, 175231406.25, 176225625.0, 177222656.25, 178222500.0, 179225156.25, 180230625.0, 181238906.25, 182250000.0, 183263906.25, 184280625.0, 185300156.25, 186322500.0, 187347656.25, 188375625.0, 189406406.25, 190440000.0, 191476406.25, 192515625.0, 193557656.25, 194602500.0, 195650156.25, 196700625.0, 197753906.25, 198810000.0, 199868906.25, 200930625.0, 201995156.25, 203062500.0, 204132656.25, 205205625.0, 206281406.25, 207360000.0, 208441406.25, 209525625.0, 210612656.25, 211702500.0, 212795156.25, 213890625.0, 214988906.25, 216090000.0, 217193906.25, 218300625.0, 219410156.25, 220522500.0, 221637656.25, 222755625.0, 223876406.25, 225000000.0, 226126406.25, 227255625.0, 228387656.25, 229522500.0, 230660156.25, 231800625.0, 232943906.25, 234090000.0, 235238906.25, 236390625.0, 237545156.25, 238702500.0, 239862656.25, 241025625.0, 242191406.25, 243360000.0, 244531406.25, 245705625.0, 246882656.25, 248062500.0, 249245156.25, 250430625.0, 251618906.25, 252810000.0, 254003906.25, 255200625.0, 256400156.25, 257602500.0, 258807656.25, 260015625.0, 261226406.25, 262440000.0, 263656406.25, 264875625.0, 266097656.25, 267322500.0, 268550156.25, 269780625.0, 271013906.25, 272250000.0, 273488906.25, 274730625.0, 275975156.25, 277222500.0, 278472656.25, 279725625.0, 280981406.25, 282240000.0, 283501406.25, 284765625.0, 286032656.25, 287302500.0, 288575156.25, 289850625.0, 291128906.25, 292410000.0, 293693906.25, 294980625.0, 296270156.25, 297562500.0, 298857656.25, 300155625.0, 301456406.25, 302760000.0, 304066406.25, 305375625.0, 306687656.25, 308002500.0, 309320156.25, 310640625.0, 311963906.25, 313290000.0, 314618906.25, 315950625.0, 317285156.25, 318622500.0, 319962656.25, 321305625.0, 322651406.25, 324000000.0, 325351406.25, 326705625.0, 328062656.25, 329422500.0, 330785156.25, 332150625.0, 333518906.25, 334890000.0, 336263906.25, 337640625.0, 339020156.25, 340402500.0, 341787656.25, 343175625.0, 344566406.25, 345960000.0, 347356406.25, 348755625.0, 350157656.25, 351562500.0, 352970156.25, 354380625.0, 355793906.25, 357210000.0, 358628906.25, 360050625.0, 361475156.25, 362902500.0, 364332656.25, 365765625.0, 367201406.25, 368640000.0, 370081406.25, 371525625.0, 372972656.25, 374422500.0, 375875156.25, 377330625.0, 378788906.25, 380250000.0, 381713906.25, 383180625.0, 384650156.25, 386122500.0, 387597656.25, 389075625.0, 390556406.25, 392040000.0, 393526406.25, 395015625.0, 396507656.25, 398002500.0, 399500156.25, 401000625.0, 402503906.25, 404010000.0, 405518906.25, 407030625.0, 408545156.25, 410062500.0, 411582656.25, 413105625.0, 414631406.25, 416160000.0, 417691406.25, 419225625.0, 420762656.25, 422302500.0, 423845156.25, 425390625.0, 426938906.25, 428490000.0, 430043906.25, 431600625.0, 433160156.25, 434722500.0, 436287656.25, 437855625.0, 439426406.25, 441000000.0]
  out "Altitude Array (km)":dbl[](array[numeric])=[0.0375, 0.075, 0.11249999999999999, 0.15, 0.1875, 0.225, 0.26249999999999996, 0.3, 0.33749999999999997, 0.37499999999999994, 0.4125, 0.44999999999999996, 0.48749999999999993, 0.525, 0.5625, 0.6, 0.6375, 0.6749999999999999, 0.7124999999999999, 0.75, 0.7875, 0.825, 0.8624999999999999, 0.8999999999999999, 0.9374999999999999, 0.975, 1.0125, 1.05, 1.0875000000000001, 1.125, 1.1625, 1.2, 1.2375, 1.2750000000000001, 1.3125, 1.35, 1.3875, 1.425, 1.4625000000000001, 1.5, 1.5375, 1.575, 1.6125, 1.6500000000000001, 1.6875, 1.725, 1.7625, 1.8, 1.8375, 1.875, 1.9125, 1.95, 1.9875, 2.025, 2.0625, 2.1, 2.1375, 2.175, 2.2125, 2.25, 2.2875, 2.325, 2.3625, 2.4, 2.4375, 2.475, 2.5125, 2.55, 2.5875, 2.625, 2.6625, 2.7, 2.7375, 2.775, 2.8125, 2.85, 2.8875, 2.925, 2.9625, 3.0, 3.0375, 3.075, 3.1125, 3.15, 3.1875, 3.225, 3.2625, 3.3, 3.3375, 3.375, 3.4125, 3.45, 3.4875, 3.525, 3.5625, 3.6, 3.6374999999999997, 3.675, 3.7125, 3.75, 3.7875, 3.8249999999999997, 3.8625, 3.9, 3.9375, 3.975, 4.012499999999999, 4.05, 4.0874999999999995, 4.124999999999999, 4.1625, 4.199999999999999, 4.2375, 4.2749999999999995, 4.312499999999999, 4.35, 4.387499999999999, 4.425, 4.4624999999999995, 4.499999999999999, 4.5375, 4.574999999999999, 4.6125, 4.6499999999999995, 4.687499999999999, 4.725, 4.762499999999999, 4.8, 4.8374999999999995, 4.874999999999999, 4.9125, 4.949999999999999, 4.9875, 5.0249999999999995, 5.062499999999999, 5.1, 5.137499999999999, 5.175, 5.2124999999999995, 5.249999999999999, 5.2875, 5.324999999999999, 5.3625, 5.3999999999999995, 5.437499999999999, 5.475, 5.512499999999999, 5.55, 5.5874999999999995, 5.624999999999999, 5.6625, 5.699999999999999, 5.7375, 5.7749999999999995, 5.812499999999999, 5.85, 5.887499999999999, 5.925, 5.9624999999999995, 5.999999999999999, 6.0375, 6.074999999999999, 6.1125, 6.1499999999999995, 6.187499999999999, 6.225, 6.262499999999999, 6.3, 6.3374999999999995, 6.374999999999999, 6.4125, 6.449999999999999, 6.4875, 6.5249999999999995, 6.562499999999999, 6.6, 6.637499999999999, 6.675, 6.7124999999999995, 6.749999999999999, 6.7875, 6.824999999999999, 6.8625, 6.8999999999999995, 6.937499999999999, 6.975, 7.012499999999999, 7.05, 7.0874999999999995, 7.124999999999999, 7.1625, 7.199999999999999, 7.237499999999999, 7.2749999999999995, 7.312499999999999, 7.35, 7.387499999999999, 7.424999999999999, 7.4624999999999995, 7.499999999999999, 7.5375, 7.574999999999999, 7.612499999999999, 7.6499999999999995, 7.687499999999999, 7.725, 7.762499999999999, 7.799999999999999, 7.8374999999999995, 7.874999999999999, 7.9125, 7.949999999999999, 7.987499999999999, 8.025, 8.0625, 8.1, 8.1375, 8.174999999999999, 8.212499999999999, 8.25, 8.2875, 8.325, 8.362499999999999, 8.399999999999999, 8.4375, 8.475, 8.5125, 8.549999999999999, 8.587499999999999, 8.625, 8.6625, 8.7, 8.737499999999999, 8.774999999999999, 8.8125, 8.85, 8.8875, 8.924999999999999, 8.962499999999999, 9.0, 9.0375, 9.075, 9.112499999999999, 9.149999999999999, 9.1875, 9.225, 9.2625, 9.299999999999999, 9.337499999999999, 9.375, 9.4125, 9.45, 9.487499999999999, 9.524999999999999, 9.5625, 9.6, 9.6375, 9.674999999999999, 9.712499999999999, 9.75, 9.7875, 9.825, 9.862499999999999, 9.899999999999999, 9.9375, 9.975, 10.0125, 10.049999999999999, 10.087499999999999, 10.125, 10.1625, 10.2, 10.237499999999999, 10.274999999999999, 10.3125, 10.35, 10.3875, 10.424999999999999, 10.462499999999999, 10.5, 10.5375, 10.575, 10.612499999999999, 10.649999999999999, 10.6875, 10.725, 10.7625, 10.799999999999999, 10.837499999999999, 10.875, 10.9125, 10.95, 10.987499999999999, 11.024999999999999, 11.0625, 11.1, 11.1375, 11.174999999999999, 11.212499999999999, 11.25, 11.2875, 11.325, 11.362499999999999, 11.399999999999999, 11.4375, 11.475, 11.5125, 11.549999999999999, 11.587499999999999, 11.625, 11.6625, 11.7, 11.737499999999999, 11.774999999999999, 11.8125, 11.85, 11.8875, 11.924999999999999, 11.962499999999999, 12.0, 12.0375, 12.075, 12.112499999999999, 12.149999999999999, 12.1875, 12.225, 12.2625, 12.299999999999999, 12.337499999999999, 12.375, 12.4125, 12.45, 12.487499999999999, 12.524999999999999, 12.5625, 12.6, 12.6375, 12.674999999999999, 12.712499999999999, 12.75, 12.7875, 12.825, 12.862499999999999, 12.899999999999999, 12.9375, 12.975, 13.0125, 13.049999999999999, 13.087499999999999, 13.125, 13.1625, 13.2, 13.237499999999999, 13.274999999999999, 13.3125, 13.35, 13.3875, 13.424999999999999, 13.462499999999999, 13.5, 13.5375, 13.575, 13.612499999999999, 13.649999999999999, 13.6875, 13.725, 13.7625, 13.799999999999999, 13.837499999999999, 13.875, 13.9125, 13.95, 13.987499999999999, 14.024999999999999, 14.0625, 14.1, 14.1375, 14.174999999999999, 14.212499999999999, 14.25, 14.2875, 14.325, 14.362499999999999, 14.399999999999999, 14.437499999999998, 14.475, 14.5125, 14.549999999999999, 14.587499999999999, 14.624999999999998, 14.6625, 14.7, 14.737499999999999, 14.774999999999999, 14.812499999999998, 14.85, 14.8875, 14.924999999999999, 14.962499999999999, 14.999999999999998, 15.0375, 15.075, 15.112499999999999, 15.149999999999999, 15.187499999999998, 15.225, 15.2625, 15.299999999999999, 15.337499999999999, 15.374999999999998, 15.4125, 15.45, 15.487499999999999, 15.524999999999999, 15.562499999999998, 15.6, 15.6375, 15.674999999999999, 15.712499999999999, 15.749999999999998, 15.7875, 15.825, 15.862499999999999, 15.899999999999999, 15.937499999999998, 15.975, 16.0125, 16.05, 16.087500000000002, 16.125, 16.1625, 16.2, 16.2375, 16.275000000000002, 16.3125, 16.35, 16.3875, 16.425, 16.462500000000002, 16.5, 16.5375, 16.575, 16.6125, 16.650000000000002, 16.6875, 16.725, 16.7625, 16.8, 16.837500000000002, 16.875, 16.9125, 16.95, 16.9875, 17.025000000000002, 17.0625, 17.1, 17.1375, 17.175, 17.212500000000002, 17.25, 17.2875, 17.325, 17.3625, 17.400000000000002, 17.4375, 17.475, 17.5125, 17.55, 17.587500000000002, 17.625, 17.6625, 17.7, 17.7375, 17.775000000000002, 17.8125, 17.85, 17.8875, 17.925, 17.962500000000002, 18.0, 18.0375, 18.075, 18.1125, 18.150000000000002, 18.1875, 18.225, 18.2625, 18.3, 18.337500000000002, 18.375, 18.4125, 18.45, 18.4875, 18.525000000000002, 18.5625, 18.6, 18.6375, 18.675, 18.712500000000002, 18.75, 18.7875, 18.825, 18.8625, 18.900000000000002, 18.9375, 18.975, 19.0125, 19.05, 19.087500000000002, 19.125, 19.1625, 19.2, 19.2375, 19.275000000000002, 19.3125, 19.35, 19.3875, 19.425, 19.462500000000002, 19.5, 19.5375, 19.575, 19.6125, 19.650000000000002, 19.6875, 19.725, 19.7625, 19.8, 19.837500000000002, 19.875, 19.9125, 19.95, 19.9875, 20.025000000000002, 20.0625, 20.1, 20.1375, 20.175, 20.212500000000002, 20.25, 20.2875, 20.325, 20.3625, 20.400000000000002, 20.4375, 20.475, 20.5125, 20.55, 20.587500000000002, 20.625, 20.6625, 20.7, 20.7375, 20.775000000000002, 20.8125, 20.85, 20.8875, 20.925, 20.962500000000002, 21.0]
  out "Offline Pulse Energy":dbl=0.01693271857142857
  out "Online Pulse Energy":dbl=0.01695981714285714
  in  "Instrument Control":T5(tab)=enum."Wavemeter"
  out "Readings":T6={"OnLineTEC"=14.1685429, "OnLineLD"=0.160554692, "OffLineTEC"=23.318903, "OffLineLD"=0.00014843751, "EtalonTEC"=30.0243149, "TSOA-TEC"=19.0057316, "Pro8000"=TRUE, "OnLine TEC"=TRUE, "OnLine LD"=TRUE, "OffLine TEC"=FALSE, "OffLine LD"=FALSE, "Etalon TEC"=TRUE, "TSOA TEC"=TRUE} {"OffLineLD" format="%.4g"; "OnLineLD" format="%.4g"; "TSOA-TEC" format="%.3g"; "EtalonTEC" format="%.3g"; "OffLineTEC" format="%.3g"; "OnLineTEC" format="%.3g"}
  in  "Settings":T7={"Module"=enum."On Line TEC", "OnLineTEC"=14.167749999999609, "OnLineLD"=0.16, "OffLineTEC"=29.780200000000985, "OffLineLD"=0.173, "EtalonTEC"=30.0, "TSOA-TEC"=19.0} {"OffLineLD" min=0.0 max=0.175 step=0.001 format="%.3p"; "OnLineLD" min=0.0 max=0.175 step=0.001 format="%.3p"; "TSOA-TEC" format="%.2g"; "EtalonTEC" format="%.2g"; "OffLineTEC" min=0.0 max=30.0 step=0.1 format="%.3g"; "OnLineTEC" min=0.0 max=30.0 step=0.1 format="%.3g"}
  in  "Device In":refnum<visa-resource-name>="Pro8000"
  in  "Pulse B Polarity":enum32{"Low", "High"}(ring)=enum."High"
  in  "Pulse A Delay(ns)":u32=1040 min=80 max=327600
  in  "Pulse B Delay(ns)":u32=170000 min=80 max=327600 step=1
  in  "Accumulation Delay(ns)":u32=10 min=10 max=1270 step=1
  in  "Sync Pulse Polarity":enum32{"Low", "High"}(ring)=enum."High"
  in  "Pulse A Polarity":enum32{"Low", "High"}(ring)=enum."High"
  in  "Number of Bins":u32=560 min=2 max=4095 step=1
  in  "Number of Accumulates":u32=14285 min=1 max=32767 step=1
  in  "Time Resolution Per Bin(ns)":u32=250 min=5 max=1063 step=1
  out "AMCS_Profile":i32=1305
  in  "Lambda On Set (nm)":dbl=780.24612 format="%.5f"
  out "Lambda On Read (nm)":dbl=780.2461420023224 format="%.5f"
  out "Lambda Off Read (nm)":dbl=780.2461414438 format="%.5f"
  in  "Lambda Off Set (nm)":dbl=780.24612 format="%#.5f"
  in  "Bristol In":i32=5
  out "Bristol Out":i32
  out "WL_Difference":dbl=2.2002322339176317e-05 format="%#_3e"
  out "WL Difference off":dbl=2.1443799937514996e-05 format="%#_3e"
  out "Wavelength Lock Online":bool=TRUE
  out "Wavelength Lock Offline":bool=TRUE
  in  "calculate absorption cross sections":bool
  in  "Online_Tol":dbl=5e-05 format="%#_15g"
  in  "Cancel online":bool
  in  "Offline_Tol":dbl=0.001 format="%#_15g"
  in  "Cancel Offline":bool
  in  "y":dbl=0.0001 format="%#_6p"
  in  "Smoothing Range":dbl=150.0
  in  "Total DIAL Integration Time (Minutes)":i32=3
  in  "Data Reads (number of loops)":i32=1
  in  "Total Aerosol Integration Time (Minutes)":dbl=0.5
  in  "Scalar Wait Time":u32
  out "Smoothed Bins":dbl=4.0
  in  "NewportIn":string
  in  "logging":bool
  out "Newport Device Key":string="1918-R 15120"
  in  "SampleSize":i32=2
  out "NewportRef":refnum<k24>
  in  "Switch Comm Port":refnum<visa-resource-name>="COM3"
  out "FF_On_Ref":refnum<file>
  out "FF_On_Ptr":i64=4206512 format="%.2p"
  out "FF_Off_Ref":refnum<file>
  out "FF_Off_Ptr":i64=4206512 format="%.2p"
  out "NF_On_Ref":refnum<file>
  out "NF_On_Ptr":i64=4206512 format="%.2p"
  out "NF_Off_Ref":refnum<file>
  out "NF_Off_Ptr":i64=4206512 format="%.2p"
  out "DataOpen":bool=TRUE
  out "File Path_Far Field (out)":string="C:\\Users\\H2ODial\\Desktop\\SharedTeleWVData\\170302FF\\22"
  out "File Path_Near Field (out)":string="C:\\Users\\H2ODial\\Desktop\\SharedTeleWVData\\170302NF\\22"
  in  "Data File DIR (in)":string="C:\\Users\\H2ODial\\Desktop\\SharedTeleWVData\\"
  out "TRHP":T8={"Temp C"=10.05173992673992, "RelH %"=16.25915750915751, "Press hPa"=844.793956043956, "AbH g/m^3"=1.4346764346764347}
  in  "WS visa":refnum<visa-resource-name>="LuftWS"
  in  "WS_On/Off":bool=TRUE
  in  "bins":u32=560 min=2 max=4095 step=1
  out "y offset":u32=10
  in  "ns scale":u32=250
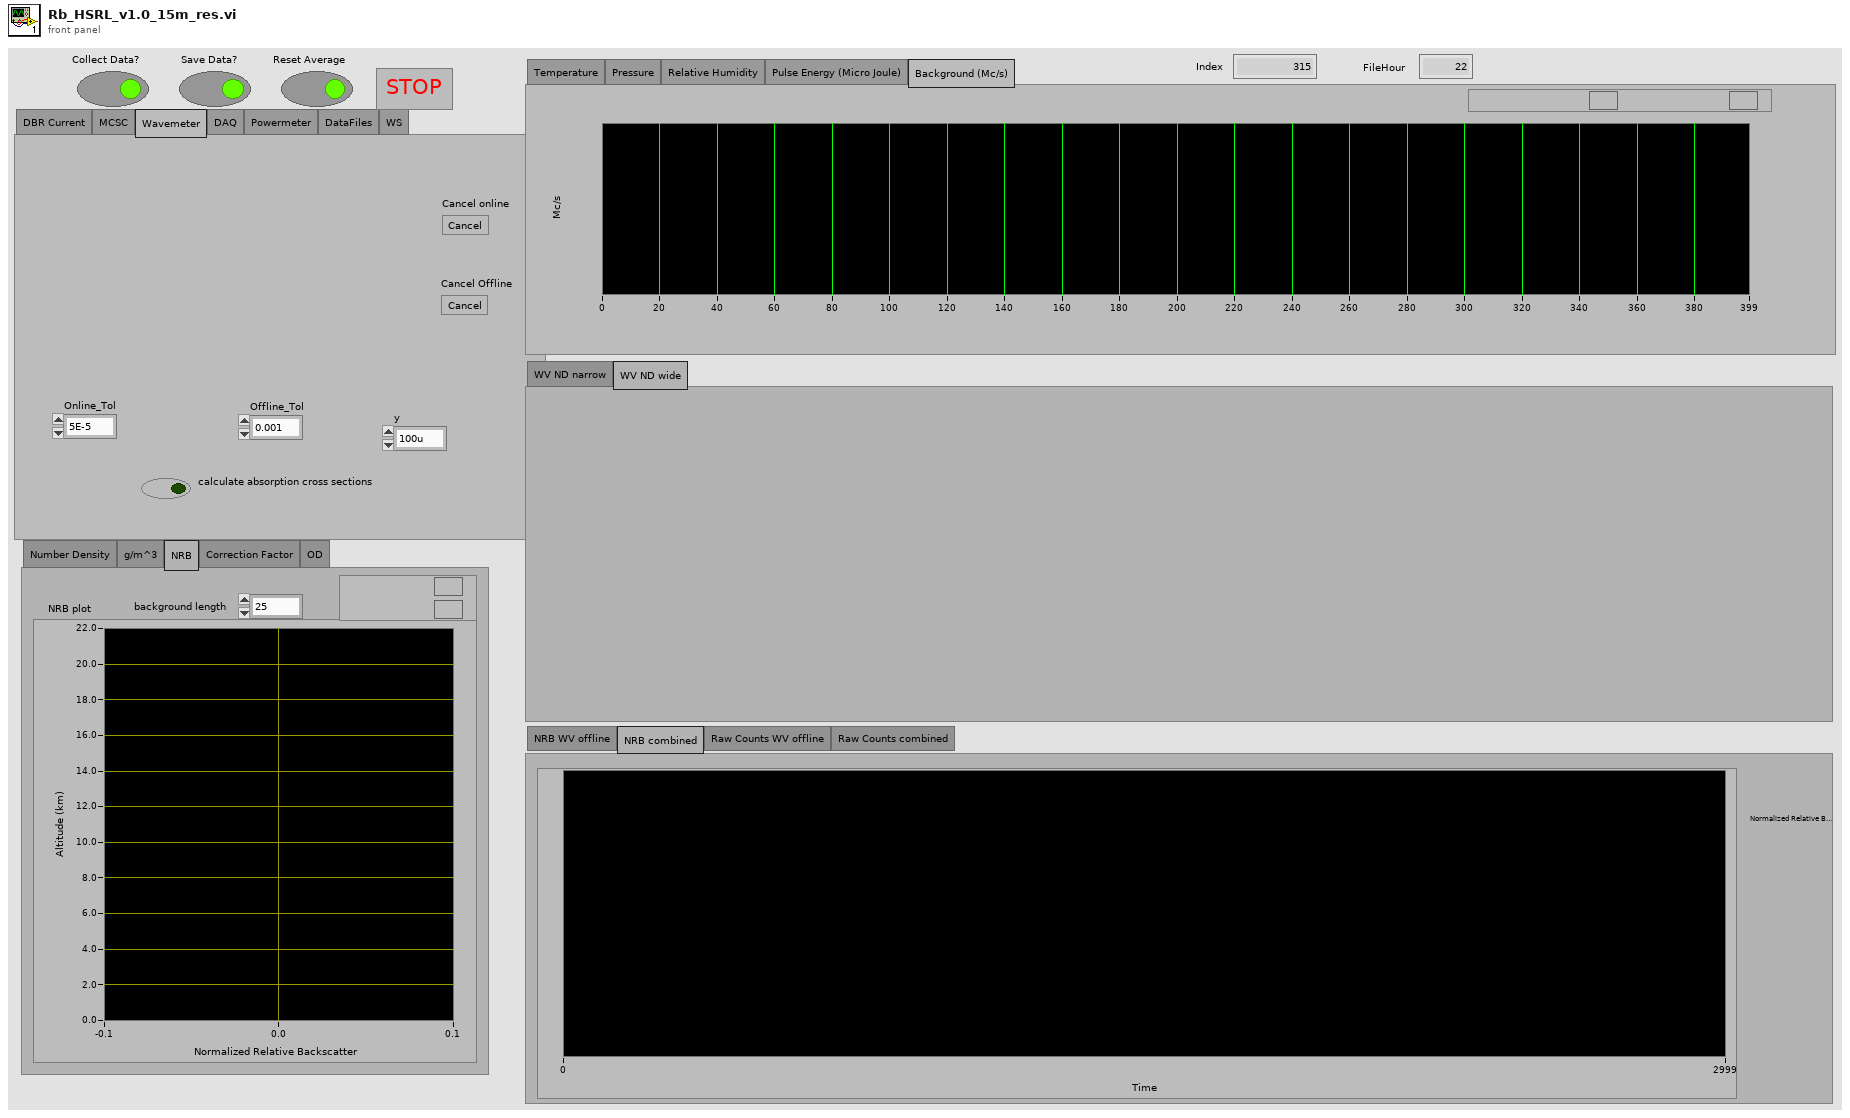
[diagram p1: front panel]
types:
  T1 = enum32{"NRB WV offline", "NRB combined", "Raw Counts WV offline", "Raw Counts combined"}
  T2 = enum32{"Number Density", "g/m^3", "NRB", "Correction Factor", "OD"}
  T3 = enum32{"Temperature", "Pressure", "Relative Humidity", "Pulse Energy (Micro Joule)", "Background (Mc/s)"}
  T4 = cluster{"Online Pulse Energy":dbl, "Pulse Energy Offline":dbl}
  T5 = enum32{"DBR Current", "MCSC", "Wavemeter", "DAQ", "Powermeter", "DataFiles", "WS"}
  T6 = cluster{"OnLineTEC":dbl, "OnLineLD":dbl, "OffLineTEC":dbl, "OffLineLD":dbl, "EtalonTEC":dbl, "TSOA-TEC":dbl, "Pro8000":bool, "OnLine TEC":bool, "OnLine LD":bool, "OffLine TEC":bool, "OffLine LD":bool, "Etalon TEC":bool, "TSOA TEC":bool}
  T7 = cluster{"Module":enum16{"On Line TEC", "On Line LD", "Off Line TEC", "Off Line LD", "Etalon TEC", "TSOA TEC"}, "OnLineTEC":dbl, "OnLineLD":dbl, "OffLineTEC":dbl, "OffLineLD":dbl, "EtalonTEC":dbl, "TSOA-TEC":dbl}
  T8 = cluster{"Temp C":dbl, "RelH %":dbl, "Press hPa":dbl, "AbH g/m^3":dbl}
  T9 = enum16{"Open_TL", "Close_TL", "Verify_ID", "TEC_Sensor", "SET", "READ", "ON", "OFF", "Set_Limits", "Read_Limits", "Enable_Status", "Read_Status"}
  T10 = enum16{"Initialize ILX", "Set ON T", "Set Off T", "Set ON I", "Set Off I", "Set On Lim", "Set Off Lim", "Read ILX", "TEC ON/OFF", "LASER ON/OFF", "Status?", "ILX OFF"}
  T11 = enum16{"open", "replace", "create", "open or create", "replace or create", "replace or create with confirmation"}
  T12 = enum16{"On Line TEC", "On Line LD", "Off Line TEC", "Off Line LD", "Etalon TEC", "TSOA TEC"}
  T13 = cluster{"Temp":dbl, "RelH":dbl, "Press":dbl, "AbH":dbl}
  T14 = typedef "LVDateTimeRec.ctl" = cluster{"fractional second":dbl, "second":i32, "minute":i32, "hour":i32, "day of month":i32, "month":i32, "year":i32, "day of week":i32, "day of year":i32, "DST":i32}
  T15 = cluster{"Online Pulse Energy":dbl, "Offline Pulse Energy":dbl}
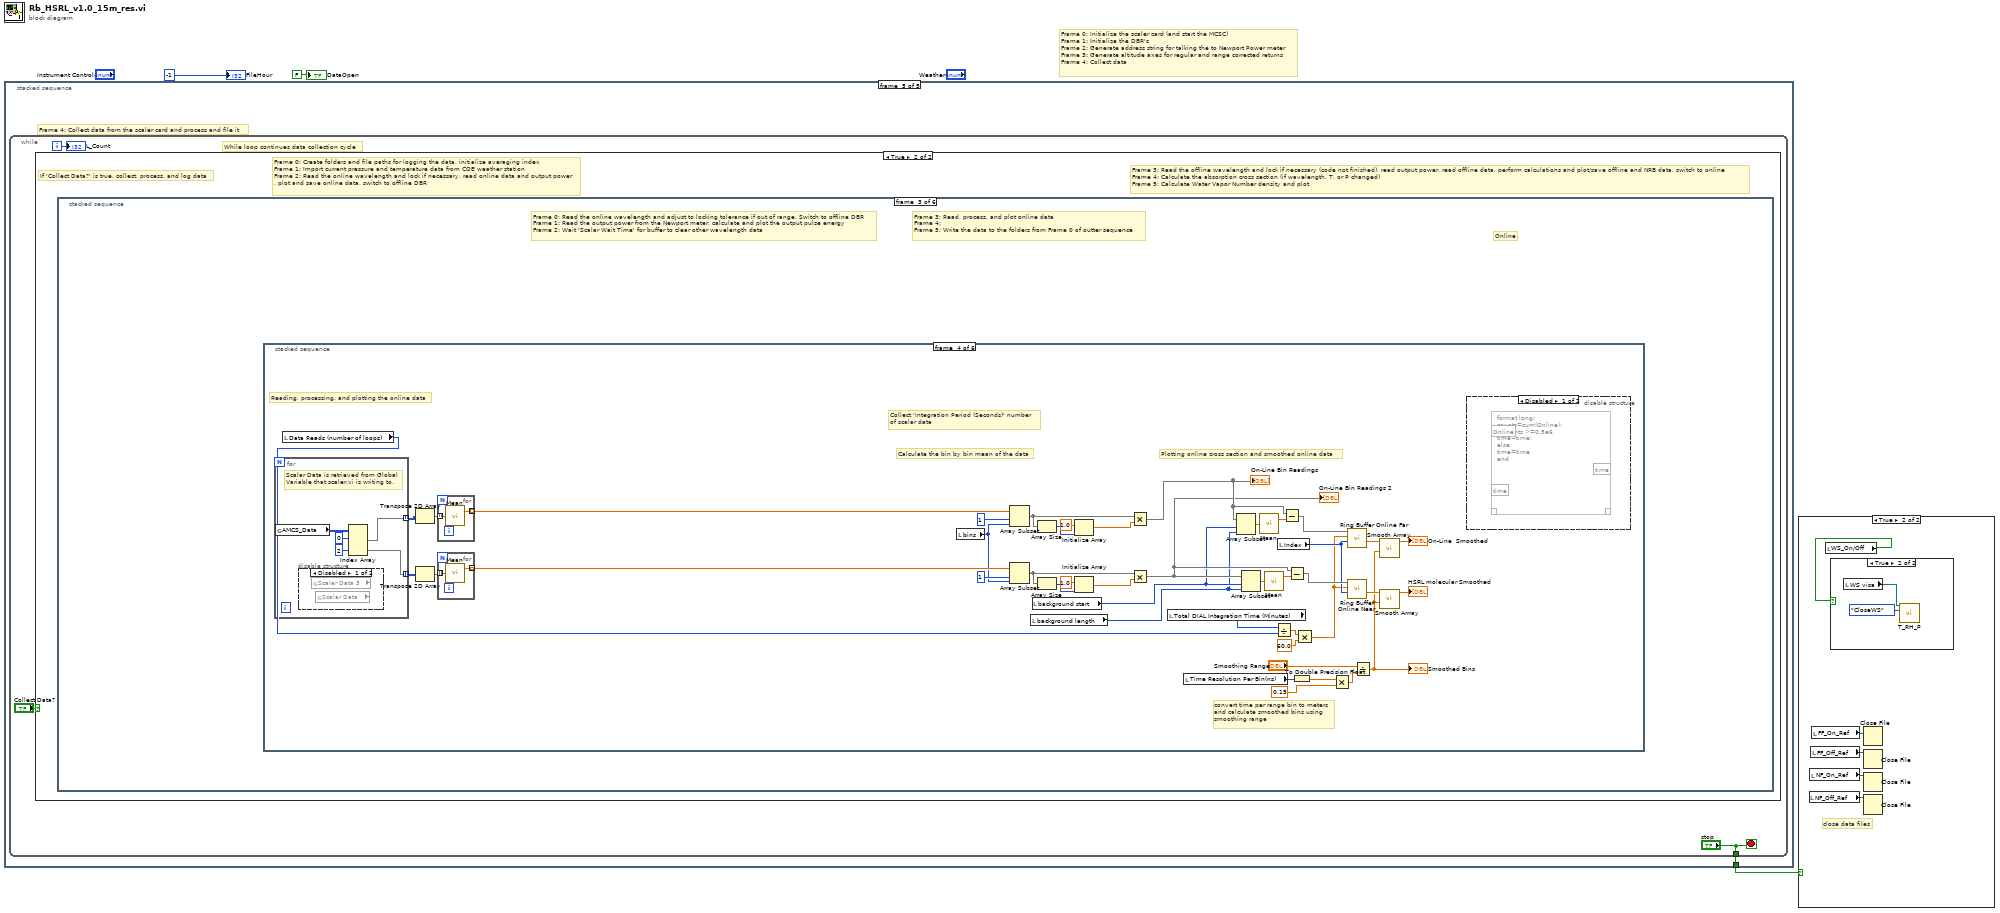
[diagram p0: block diagram]
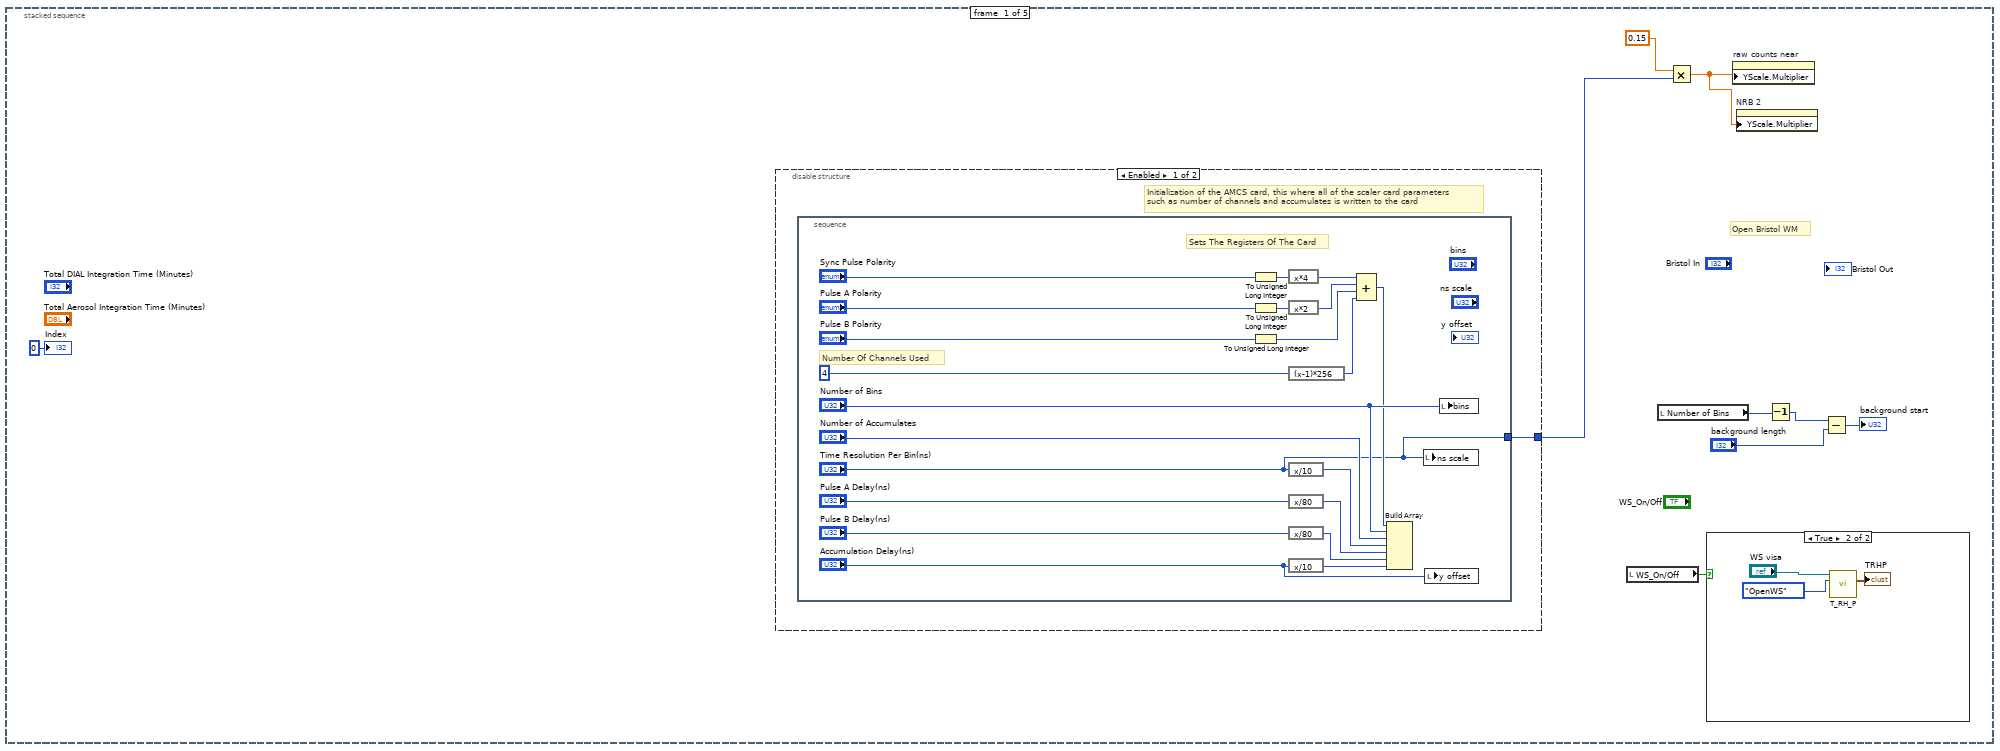
[diagram p4: hidden frame]
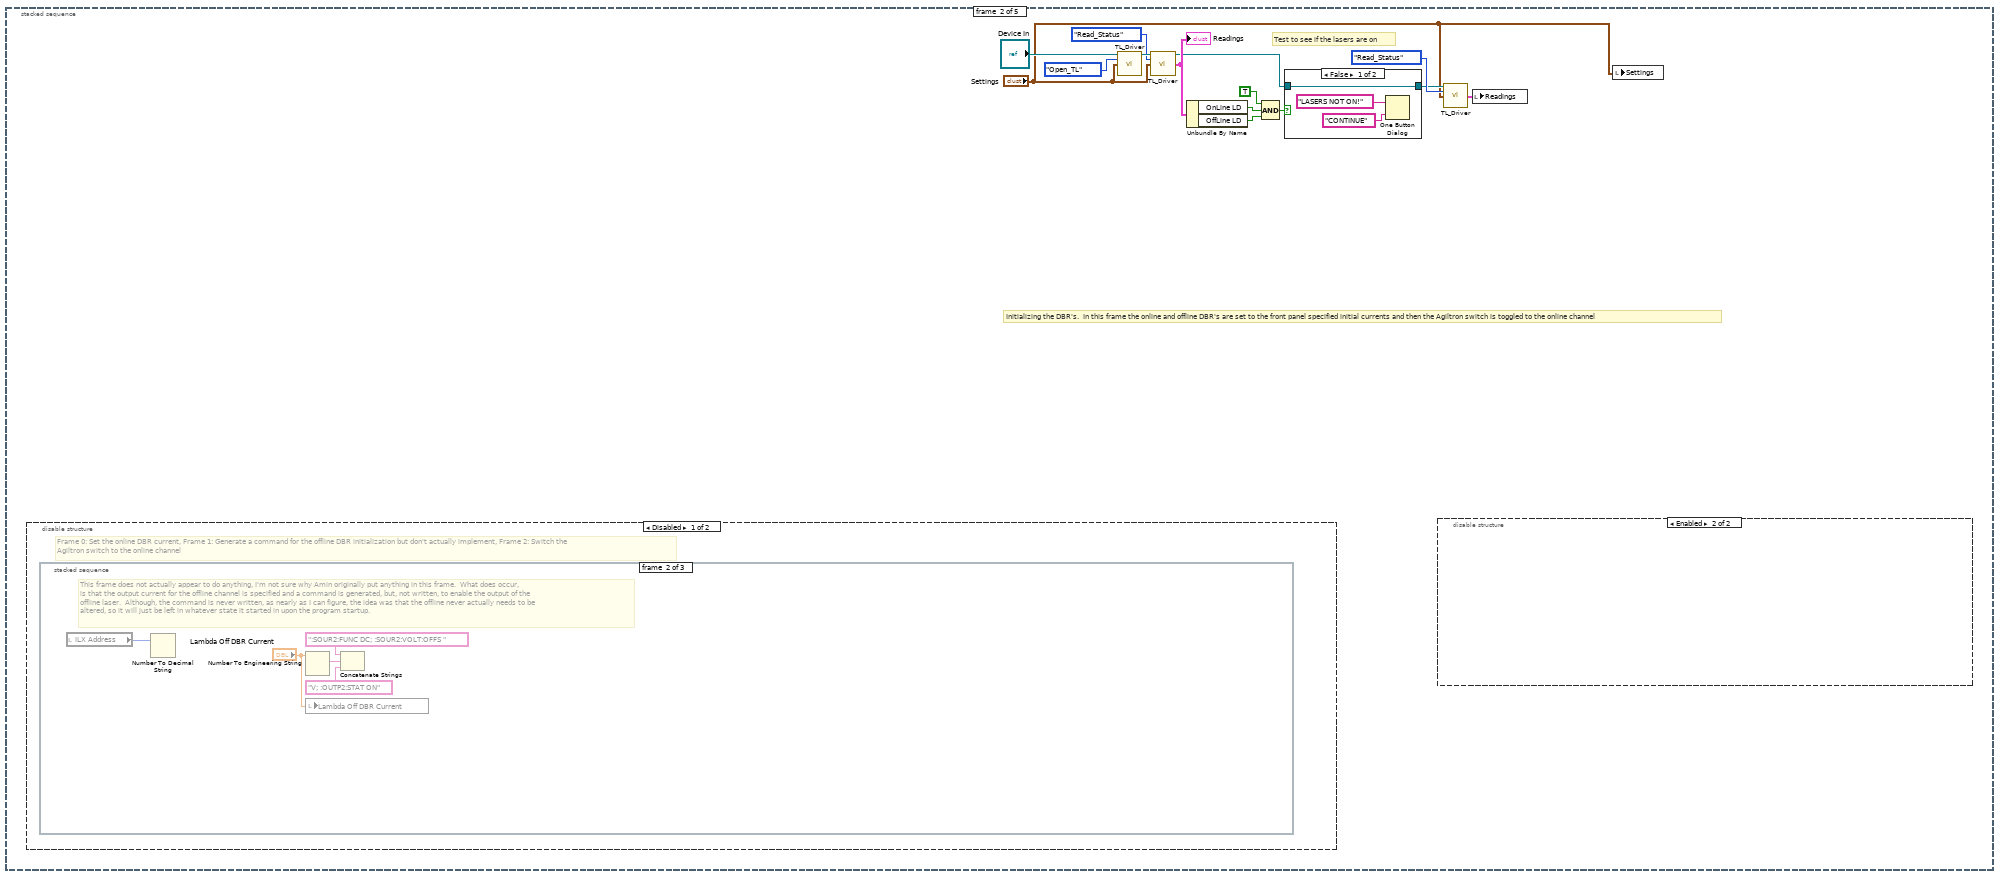
[diagram p7: hidden frame]
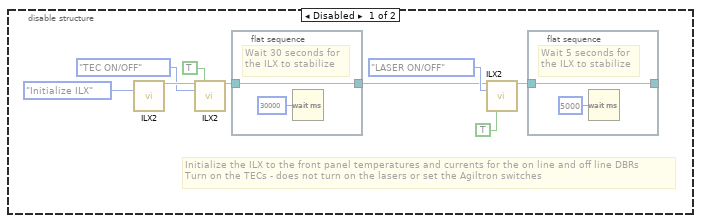
[diagram p9: hidden frame]
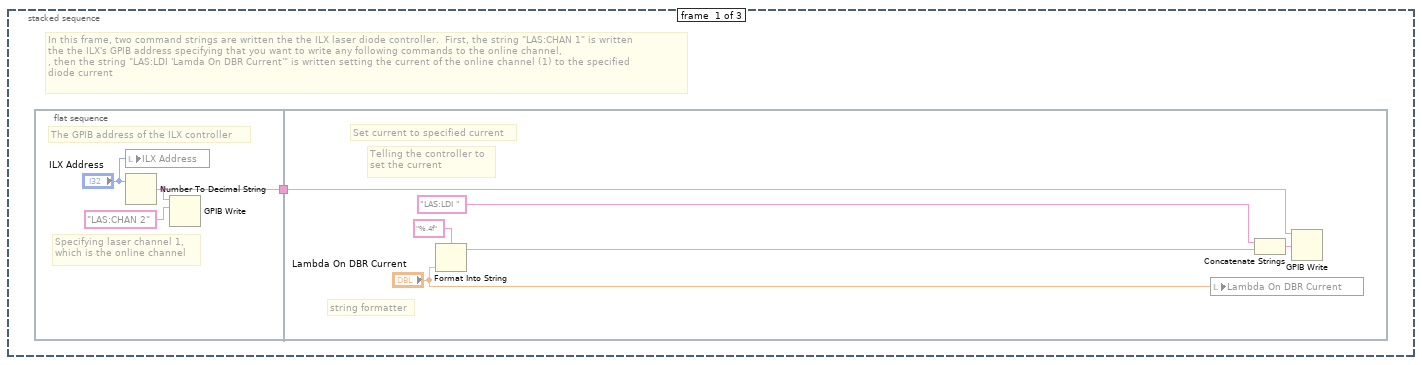
[diagram p10: hidden frame]
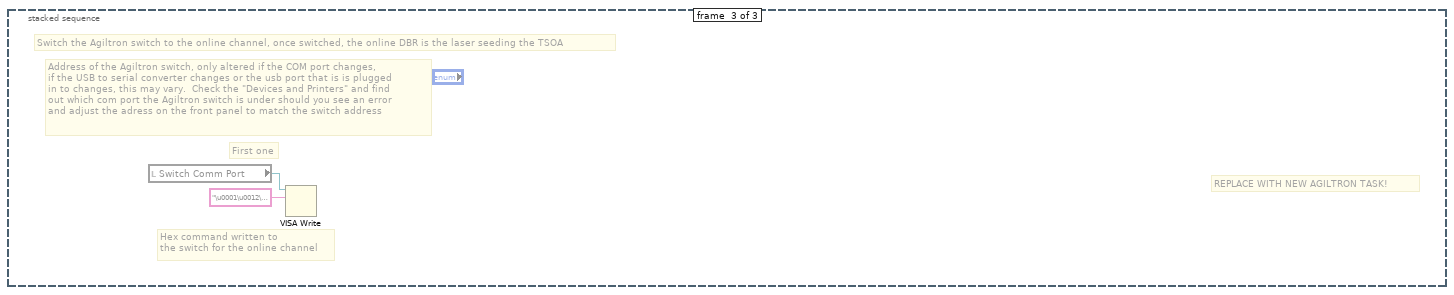
[diagram p11: hidden frame]
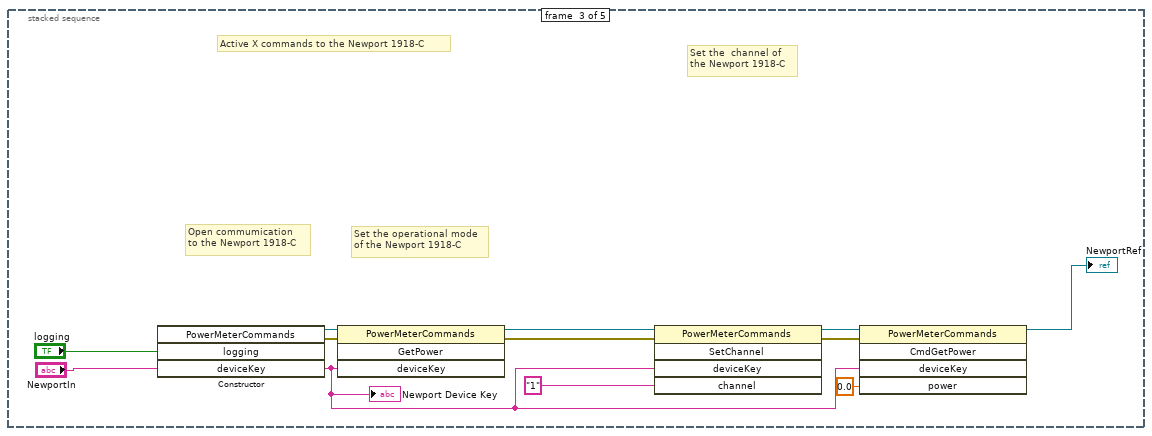
[diagram p13: hidden frame]
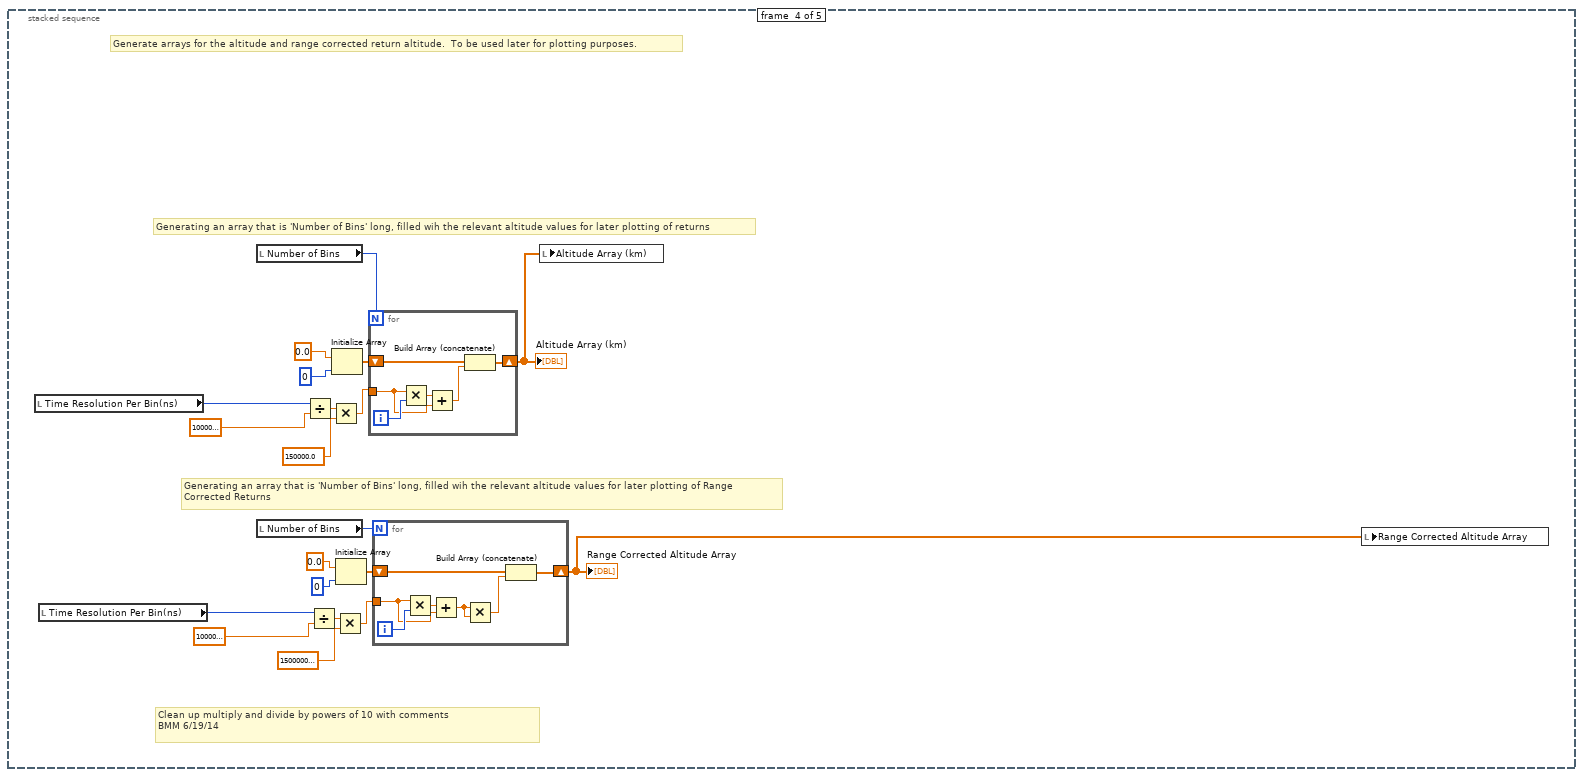
[diagram p14: hidden frame]
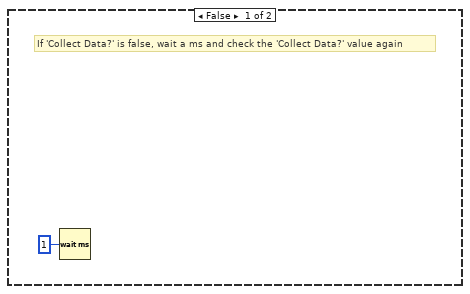
[diagram p15: hidden frame]
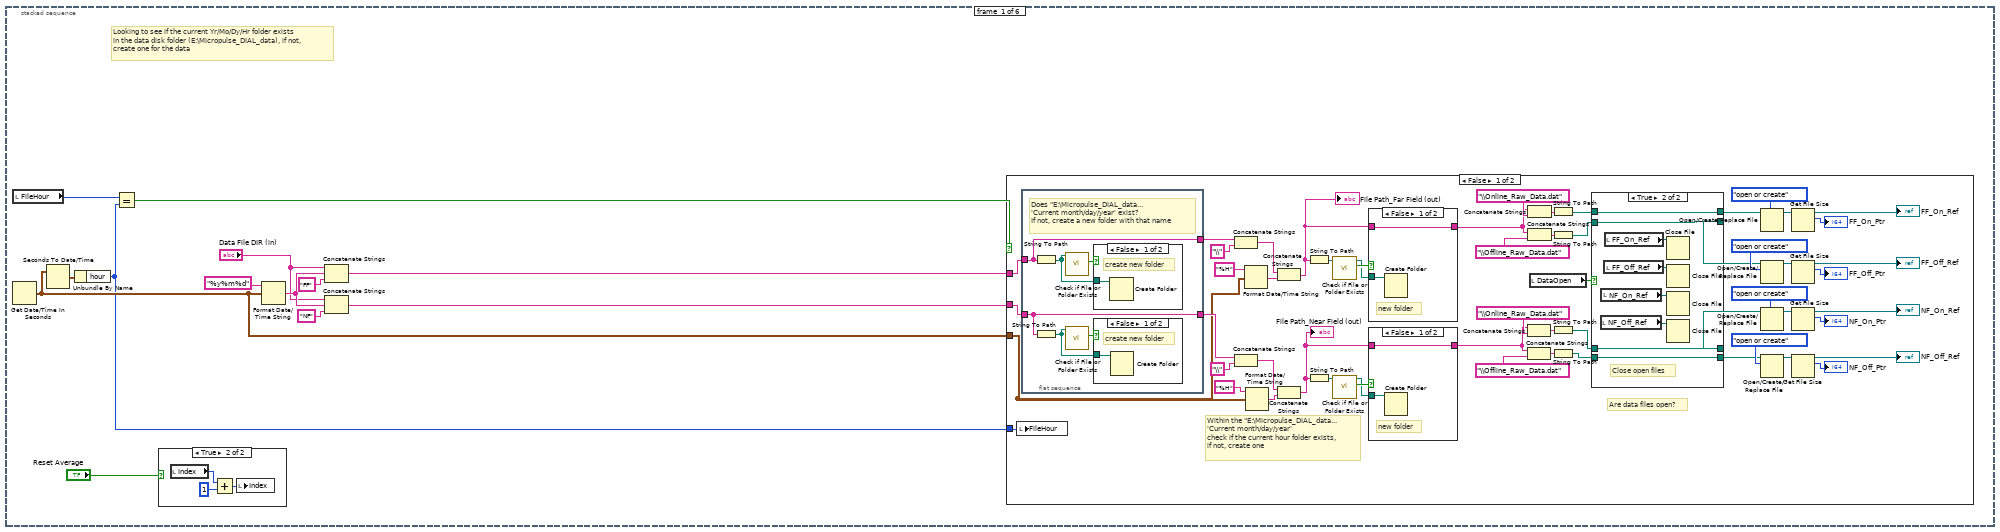
[diagram p16: hidden frame]
diagram:
  # "Frame 0: Initialize the scaler card (and start the MCSC)\nFrame 1: Initialize the DBR's\nFrame 2: Generate address string for talking the to Newport Power meter\nFrame 3: Generate altitude axes for regular and range corrected returns\nFrame 4: Collect data"
  n1 = stacked-sequence {
    tunnel: [_ _ _ _ w131] -> w3
    frame #0 {
      # "Open Bristol WM"
      n2 = disable-structure shown="Enabled" {
        disable-tunnel: [w16 _] -> w5
        frame Enabled {
          # "Initialization of the AMCS card, this where all of the scaler card parameters\nsuch as number of channels and accumulates is written to the card"
          n3 = stacked-sequence {
            tunnel: ["Time Resolution Per Bin(ns)"] -> w16
            frame #0 {
              # "Sets The Registers Of The Card"
              # "Number Of Channels Used"
              n4 = To Unsigned Long Integer(number="Sync Pulse Polarity") -> (unsigned 32bit integer=w18:u32)
              n5 = To Unsigned Long Integer(number="Pulse A Polarity") -> (unsigned 32bit integer=w22:u32)
              n6 = To Unsigned Long Integer(number="Pulse B Polarity") -> (unsigned 32bit integer=w20:u32)
              n7 = expression code="x*4"(w18) -> (w27:u32)
              n8 = expression code="x*2"(w22) -> (w26:u32)
              n9 = expression code="(x-1)*256"(u32 4 ("Number of Channels Used")) -> (w25:u32)
              n10 = expression code="x/10"("Time Resolution Per Bin(ns)") -> (w28:u32)
              n11 = expression code="x/80"("Pulse A Delay(ns)") -> (w35:u32)
              n12 = expression code="x/80"("Pulse B Delay(ns)") -> (w37:u32)
              n13 = expression code="x/10"("Accumulation Delay(ns)") -> (w36:u32)
              n14 = Compound Arithmetic op=ADD(w27, w26, w20, w25) -> (w24:u32)
              n15 = Build Array(w24, "Number of Bins", "Number of Accumulates", w28, w35, w37, w36) -> ()  [unwired: 1 out]
              n16 = local write "ns scale"("Time Resolution Per Bin(ns)") -> ()
              n17 = local write "y offset"("Accumulation Delay(ns)") -> ()
              n18 = local write "bins"("Number of Bins") -> ()
            }
          }
        }
        frame Disabled {
        }
      }
      n19 = local read "WS_On/Off"() -> (w7:bool)
      n20 = local read "Number of Bins"() -> (w11:u32)
      n21 = Multiply(x=0.15, y=w5) -> (x*y=w4:dbl)
      n22 = case shown="True" w7 {
        frame False {
        }
        frame True {
          n23 = call "T_RH_P.vi"("VISA in"="WS visa", "WS_Commands"=enum16{"OpenWS", "ReadTRHP", "CloseWS"}."OpenWS") -> ("TRHP"=→"TRHP":T13)  [unwired: 11 in, 2 out]
        }
      }
      n24 = property on="raw counts near" class="IntChart (strict)"("YScale.Multiplier"=w4) -> ()  [unwired: 2 in, 2 out]
      n25 = property on="NRB 2" class="IntChart (strict)"("YScale.Multiplier"=w4) -> ()  [unwired: 2 in, 2 out]
      n26 = Decrement(x=w11) -> (x-1=w10:u32)
      n27 = Subtract(x=w10, y="background length") -> (x-y=→"background start":u32)
      "Index" <- 0 ("Index")
    }
    frame #1 {
      # "Test to see if the lasers are on"
      # "Initializing the DBR's.  In this frame the online and offline DBR's are set to the front panel specified initial currents and then the Agiltron switch is toggled to the online channel"
      n28 = disable-structure shown="Disabled" {
        frame Disabled {
          # "Frame 0: Set the online DBR current, Frame 1: Generate a command for the offline DBR initialization but don't actually implement, Frame 2: Switch the \nAgiltron switch to the online channel"
          n29 = stacked-sequence {
            frame #0 {
              # "In this frame, two command strings are written the the ILX laser diode controller.  First, the string \"LAS:CHAN 1\" is written\nthe the ILX's GPIB address specifying that you want to write any following commands to the online channel,\n, then the string \"LAS:LDI 'Lamda On DBR Current'\" is written setting the current of the online channel (1) to the specified \ndiode current"
              n30 = flat-sequence {
                tunnel: [w71] -> w69
                tunnel: w69 -> [w73]
                frame #0 {
                  # "The GPIB address of the ILX controller"
                  # "Specifying laser channel 1,\nwhich is the online channel"
                  n31 = local write "ILX Address"("ILX Address") -> ()
                  n32 = Number To Decimal String(number="ILX Address") -> (decimal integer string=w71:string)  [unwired: 1 in]
                  n33 = GPIB Write(0:w71, 1:"LAS:CHAN 2") -> ()  [unwired: 3 in, 2 out]
                }
                frame #1 {
                  # "Telling the controller to\nset the current"
                  # "string formatter"
                  # "Set current to specified current"
                  n34 = Format Into String(format string="%.4f" ("Format String"), "Lambda On DBR Current") -> (resulting string=w76:string)  [unwired: 2 in, 1 out]
                  n35 = local write "Lambda On DBR Current"("Lambda On DBR Current") -> ()
                  n36 = Concatenate Strings("LAS:LDI ", w76) -> (w77:string)
                  n37 = GPIB Write(0:w73, 1:w77) -> ()  [unwired: 3 in, 2 out]
                }
              }
            }
            frame #1 {
              # "This frame does not actually appear to do anything, I'm not sure why Amin originally put anything in this frame.  What does occur, \nis that the output current for the offline channel is specified and a command is generated, but, not written, to enable the output of the\noffline laser.  Although, the command is never written, as nearly as I can figure, the idea was that the offline never actually needs to be \naltered, so it will just be left in whatever state it started in upon the program startup."
              n38 = local read "ILX Address"() -> (w79:i32)
              n39 = Number To Decimal String(number=w79) -> ()  [unwired: 1 in, 1 out]
              n40 = Number To Engineering String(4:"Lambda Off DBR Current") -> (0:w83:string)  [unwired: 3 in]
              n41 = local write "Lambda Off DBR Current"("Lambda Off DBR Current") -> ()
              n42 = Concatenate Strings(":SOUR2:FUNC DC; :SOUR2:VOLT:OFFS ", w83, "V; :OUTP2:STAT ON") -> ()  [unwired: 1 out]
            }
            frame #2 {
              # "REPLACE WITH NEW AGILTRON TASK!"
              # "First one"
              # "Address of the Agiltron switch, only altered if the COM port changes,\nif the USB to serial converter changes or the usb port that is is plugged\nin to changes, this may vary.  Check the \"Devices and Printers\" and find \nout which com port the Agiltron switch is under should you see an error \nand adjust the adress on the front panel to match the switch address"
              # "Hex command written to \nthe switch for the online channel"
              # "Switch the Agiltron switch to the online channel, once switched, the online DBR is the laser seeding the TSOA"
              n43 = local read "Switch Comm Port"() -> (w84:refnum<visa-resource-name>)
              n44 = VISA Write(VISA resource name=w84, write buffer="\u0001\u0012\u0000\u0002") -> ()  [unwired: 1 in, 3 out]
            }
          }
        }
        frame Enabled {
        }
      }
      n45 = call "TL_Driver.vi"("Device In"="Device In", "Commands"=T9."Open_TL", "Settings"="Settings") -> ("Device Out"=w49:refnum<visa-resource-name>)  [unwired: 9 in, 3 out]
      n46 = call "TL_Driver.vi"("Device In"=w49, "Commands"=T9."Read_Status", "Settings"="Settings") -> ("Device Out"=w46:refnum<visa-resource-name>, "Readings"=w47:T6)  [unwired: 9 in, 2 out]
      "Readings" <- w47
      n47 = Unbundle By Name(w47) -> ("OnLine LD"=w41:bool, "OffLine LD"=w42:bool)
      n48 = Compound Arithmetic op=AND(TRUE, w41, w42) -> (w40:bool)
      n49 = case shown="False" w40 {
        tunnel: w46 -> [w52 w55]
        tunnel: [w52 w55] -> w44
        frame False {
          n50 = One Button Dialog(message="LASERS NOT ON!", button name ("OK")="CONTINUE") -> ()  [unwired: 1 out]
        }
        frame True {
        }
      }
      n51 = disable-structure shown="Enabled" {
        frame Disabled {
          # "Initialize the ILX to the front panel temperatures and currents for the on line and off line DBRs\nTurn on the TECs - does not turn on the lasers or set the Agiltron switches"
          n52 = call "ILX2.vi"("ILX Command"=T10."Initialize ILX") -> ("Device Out"=w63:refnum<visa-resource-name>)  [unwired: 10 in, 4 out]
          n53 = call "ILX2.vi"("Device In"=w63, "TEC Control"=TRUE, "ILX Command"=T10."TEC ON/OFF") -> ("Device Out"=w60:refnum<visa-resource-name>)  [unwired: 8 in, 4 out]
          n54 = flat-sequence {
            tunnel: w60 -> [w67]
            tunnel: [w67] -> w57
            frame #0 {
              # "Wait 30 seconds for\nthe ILX to stabilize"
              n55 = Wait (ms)(milliseconds to wait=u32 30000) -> ()  [unwired: 1 out]
            }
          }
          n56 = call "ILX2.vi"("Device In"=w57, "ILX Command"=T10."LASER ON/OFF", "Laser Control"=TRUE ("TEC Control")) -> ("Device Out"=w56:refnum<visa-resource-name>)  [unwired: 8 in, 4 out]
          n57 = flat-sequence {
            tunnel: w56 -> [w65]
            tunnel: [w65] -> _
            frame #0 {
              # "Wait 5 seconds for\nthe ILX to stabilize"
              n58 = Wait (ms)(milliseconds to wait=u32 5000) -> ()  [unwired: 1 out]
            }
          }
        }
        frame Enabled {
        }
      }
      n59 = call "TL_Driver.vi"("Device In"=w44, "Commands"=T9."Read_Status", "Settings"="Settings") -> ("Readings"=w38:T6)  [unwired: 9 in, 3 out]
      n60 = local write "Readings"(w38) -> ()
      n61 = local write "Settings"("Settings") -> ()
    }
    frame #2 {
      # "Active X commands to the Newport 1918-C"
      # "Set the  channel of\nthe Newport 1918-C"
      # "Set the operational mode\nof the Newport 1918-C"
      # "Open commumication\nto the Newport 1918-C"
      n62 = constructor class="PowerMeterCommands"("logging"="logging", "deviceKey"="NewportIn") -> (reference out=w97:refnum<k24>, error out=w94:errorcluster, "deviceKey"=w89:string)  [unwired: 3 in, 2 out]
      "Newport Device Key" <- w89
      n63 = invoke class="PowerMeterCommands" method="GetPower"(reference=w97, error in=w94, "deviceKey"=w89) -> (reference out=w96:refnum<k24>, error out=w93:errorcluster)  [unwired: 1 in, 2 out]
      n64 = invoke class="PowerMeterCommands" method="SetChannel"(reference=w96, error in=w93, "deviceKey"=w89, "channel"="1") -> (reference out=w90:refnum<k24>, error out=w92:errorcluster)  [unwired: 1 in, 3 out]
      n65 = invoke class="PowerMeterCommands" method="CmdGetPower"(reference=w90, error in=w92, "deviceKey"=w89, "power"=sgl 0.0) -> (reference out=→"NewportRef":refnum<k24>)  [unwired: 1 in, 4 out]
    }
    frame #3 {
      # "Clean up multiply and divide by powers of 10 with comments\nBMM 6/19/14"
      # "Generating an array that is 'Number of Bins' long, filled wih the relevant altitude values for later plotting of Range \nCorrected Returns"
      # "Generating an array that is 'Number of Bins' long, filled wih the relevant altitude values for later plotting of returns"
      # "Generate arrays for the altitude and range corrected return altitude.  To be used later for plotting purposes."
      n66 = local read "Time Resolution Per Bin(ns)"() -> (w110:u32)
      n67 = local read "Time Resolution Per Bin(ns)"() -> (w100:u32)
      n68 = local read "Number of Bins"() -> (w113:u32)
      n69 = local read "Number of Bins"() -> (w103:u32)
      n70 = Divide(x=w110, y=1000000000.0) -> (x/y=w108:dbl)
      n71 = Divide(x=w100, y=1000000000.0) -> (x/y=w98:dbl)
      n72 = Multiply(x=w108, y=150000.0) -> (x*y=w111:dbl)
      n73 = Initialize Array(0.0, 0) -> (w116:dbl[])
      n74 = Multiply(x=w98, y=150000000.0) -> (x*y=w101:dbl)
      n75 = Initialize Array(0.0, 0) -> (w106:dbl[])
      n76 = for {
        N: w113 -> [_]
        shift-right: [w129] -> w114
        shift-left: w116 -> [w130]
        tunnel: w111 -> [w126]
        i -> [w128]
        n77 = Multiply(x=w126, y=w128) -> (x*y=w127:dbl)
        n78 = Add(x=w127, y=w126) -> (x+y=w125:dbl)
        n79 = Build Array (concatenate)(w130, w125) -> (w129:dbl[])
      }
      "Altitude Array (km)" <- w114
      n80 = for {
        N: w103 -> [_]
        shift-right: [w123] -> w104
        shift-left: w106 -> [w124]
        tunnel: w101 -> [w119]
        i -> [w122]
        n81 = Multiply(x=w119, y=w122) -> (x*y=w120:dbl)
        n82 = Add(x=w120, y=w119) -> (x+y=w118:dbl)
        n83 = Multiply(x=w118, y=w118) -> (x*y=w121:dbl)
        n84 = Build Array (concatenate)(w124, w121) -> (w123:dbl[])
      }
      "Range Corrected Altitude Array" <- w104
      n85 = local write "Altitude Array (km)"(w114) -> ()
      n86 = local write "Range Corrected Altitude Array"(w104) -> ()
    }
    frame #4 {
      # "Frame 4: Collect data from the scaler card and process and file it"
      n87 = while {
        tunnel: ["stop"] -> w131
        i -> [w132]
        stop <- "stop" stop-if-true
        # "While loop continues data collection cycle"
        n88 = case shown="True" "Collect Data?" {
          frame False {
            # "If 'Collect Data?' is false, wait a ms and check the 'Collect Data?' value again"
            n89 = Wait (ms)(milliseconds to wait=u32 1) -> ()  [unwired: 1 out]
          }
          frame True {
            # "Frame 3: Read the offline wavelength and lock if necessary (code not finished), read output power, read offline data, perform calculations and plot/save offline and NRB data, switch to online\nFrame 4: Calculate the absorption cross section (if wavelength, T, or P changed)\nFrame 5: Calculate Water Vapor Number density and plot"
            # "Frame 0: Create folders and file paths for logging the data, initialize averaging index\nFrame 1: Import current pressure and temperature data from COE weather station\nFrame 2: Read the online wavelength and lock if necessary, read online data and output power\n, plot and save online data, switch to offline DBR"
            # "If 'Collect Data?' is true, collect, process, and log data"
            n90 = stacked-sequence {
              frame #0 {
                # "Looking to see if the current Yr/Mo/Dy/Hr folder exists\nin the data disk folder (E:\\Micropulse_DIAL_data), if not,\ncreate one for the data"
                n91 = local read "FileHour"() -> (w145:i32)
                n92 = Get Date/Time In Seconds() -> (seconds since 1Jan1904=w137:timestamp)
                n93 = Seconds To Date/Time(time stamp (now)=w137) -> (date time rec=w147:T14)  [unwired: 1 in]
                n94 = Unbundle By Name(w147) -> ("hour"=w136:i32)
                n95 = Equal?(x=w145, y=w136) -> (x = y?=w146:bool)
                n96 = case shown="True" "Reset Average" {
                  frame False {
                    n97 = local write "Index"(0 ("Index")) -> ()
                  }
                  frame True {
                    n98 = local read "Index"() -> (w235:i32)
                    n99 = Add(x=w235, y=1) -> (x+y=w234:i32)
                    n100 = local write "Index"(w234) -> ()
                  }
                }
                n101 = Format Date/Time String(time format string (%c)="%y%m%d", seconds (now)=w137) -> (date/time string=w141:string)  [unwired: 1 in]
                n102 = Concatenate Strings("Data File DIR (in)", w141, "FF" ("string")) -> (w143:string)
                n103 = Concatenate Strings("Data File DIR (in)", w141, "NF" ("string")) -> (w138:string)
                n104 = case shown="False" w146 {
                  tunnel: w143 -> [w205 _]
                  tunnel: w138 -> [w204 _]
                  tunnel: w137 -> [w191 _]
                  tunnel: w136 -> [w167 _]
                  frame False {
                    # "Are data files open?"
                    # "Within the \"E:\\Micropulse_DIAL_data...\n'Current month/day/year' \ncheck if the current hour folder exists,\nif not, create one"
                    n105 = local write "FileHour"(w167) -> ()
                    n106 = flat-sequence {
                      tunnel: [w225] -> w192
                      tunnel: w205 -> [w224]
                      tunnel: w204 -> [w225]
                      tunnel: [w224] -> w193
                      frame #0 {
                        # "Does \"E:\\Micropulse_DIAL_data...\n'Current month/day/year' exist?\nIf not, create a new folder with that name"
                        n107 = String To Path(string=w224) -> (path=w229:path)
                        n108 = String To Path(string=w225) -> (path=w227:path)
                        n109 = call <vilib>:"Check if File or Folder Exists.vi"("path"=w229) -> ("file or folder exists?"=w228:bool)  [unwired: 8 in, 2 out]
                        n110 = call <vilib>:"Check if File or Folder Exists.vi"("path"=w227) -> ("file or folder exists?"=w226:bool)  [unwired: 8 in, 2 out]
                        n111 = case shown="False" w228 {
                          tunnel: w229 -> [w231 _]
                          frame False {
                            # "create new folder"
                            n112 = Create Folder(path (use dialog)=w231) -> ()  [unwired: 2 in, 3 out]
                          }
                          frame True {
                            # "Folder exists\ndo nothing"
                          }
                        }
                        n113 = case shown="False" w226 {
                          tunnel: w227 -> [w230 _]
                          frame False {
                            # "create new folder"
                            n114 = Create Folder(path (use dialog)=w230) -> ()  [unwired: 2 in, 3 out]
                          }
                          frame True {
                            # "Folder exists\ndo nothing"
                          }
                        }
                      }
                    }
                    n115 = Concatenate Strings(w193, "\\" ("string")) -> (w200:string)
                    n116 = Concatenate Strings(w192, "\\" ("string")) -> (w195:string)
                    n117 = Format Date/Time String(time format string (%c)="%H", seconds (now)=w191) -> (date/time string=w203:string)  [unwired: 1 in]
                    n118 = Format Date/Time String(time format string (%c)="%H", seconds (now)=w191) -> (date/time string=w198:string)  [unwired: 1 in]
                    n119 = Concatenate Strings(w200, w203) -> (w163:string)
                    "File Path_Far Field (out)" <- w163
                    n120 = Concatenate Strings(w195, w198) -> (w164:string)
                    "File Path_Near Field (out)" <- w164
                    n121 = String To Path(string=w163) -> (path=w201:path)
                    n122 = String To Path(string=w164) -> (path=w196:path)
                    n123 = call <vilib>:"Check if File or Folder Exists.vi"("path"=w201) -> ("file or folder exists?"=w190:bool, "dup path"=w188:path)  [unwired: 8 in, 1 out]
                    n124 = call <vilib>:"Check if File or Folder Exists.vi"("path"=w196) -> ("file or folder exists?"=w189:bool, "dup path"=w187:path)  [unwired: 8 in, 1 out]
                    n125 = case shown="False" w190 {
                      tunnel: w188 -> [w222 _]
                      tunnel: w163 -> [w221 w223]
                      tunnel: [w221 w223] -> w161
                      frame False {
                        # "new folder"
                        n126 = Create Folder(path (use dialog)=w222) -> ()  [unwired: 2 in, 3 out]
                      }
                      frame True {
                        # "Folder exists\ndo nothing"
                      }
                    }
                    n127 = case shown="False" w189 {
                      tunnel: w187 -> [w219 _]
                      tunnel: w164 -> [w218 w220]
                      tunnel: [w218 w220] -> w162
                      frame False {
                        # "new folder"
                        n128 = Create Folder(path (use dialog)=w219) -> ()  [unwired: 2 in, 3 out]
                      }
                      frame True {
                        # "Folder exists\ndo nothing"
                      }
                    }
                    n129 = Concatenate Strings(w162, "\\Online_Raw_Data.dat" ("string")) -> (w181:string)
                    n130 = Concatenate Strings(w162, "\\Offline_Raw_Data.dat" ("string")) -> (w180:string)
                    n131 = Concatenate Strings(w161, "\\Online_Raw_Data.dat" ("string")) -> (w186:string)
                    n132 = Concatenate Strings(w161, "\\Offline_Raw_Data.dat" ("string")) -> (w185:string)
                    n133 = local read "DataOpen"() -> (w178:bool)
                    n134 = String To Path(string=w186) -> (path=w177:path)
                    n135 = String To Path(string=w185) -> (path=w176:path)
                    n136 = String To Path(string=w181) -> (path=w175:path)
                    n137 = String To Path(string=w180) -> (path=w174:path)
                    n138 = case shown="True" w178 {
                      tunnel: w177 -> [w209 w213]
                      tunnel: [w209 w213] -> w171
                      tunnel: w176 -> [w208 w212]
                      tunnel: [w208 w212] -> w170
                      tunnel: w175 -> [w207 w211]
                      tunnel: [w207 w211] -> w169
                      tunnel: [w206 w210] -> w168
                      tunnel: w174 -> [w206 w210]
                      frame False {
                        # "No files open\ndo nothing"
                      }
                      frame True {
                        # "Close open files"
                        n139 = local read "NF_Off_Ref"() -> (w215:refnum<file>)
                        n140 = local read "NF_On_Ref"() -> (w214:refnum<file>)
                        n141 = local read "FF_Off_Ref"() -> (w217:refnum<file>)
                        n142 = local read "FF_On_Ref"() -> (w216:refnum<file>)
                        n143 = Close File(refnum=w216) -> ()  [unwired: 1 in, 2 out]
                        n144 = Close File(refnum=w217) -> ()  [unwired: 1 in, 2 out]
                        n145 = Close File(refnum=w214) -> ()  [unwired: 1 in, 2 out]
                        n146 = Close File(refnum=w215) -> ()  [unwired: 1 in, 2 out]
                      }
                    }
                    n147 = Open/Create/Replace File(file path (use dialog)=w171, operation (0:open)=T11."open or create") -> (refnum out=w157:refnum<file>)  [unwired: 4 in, 2 out]
                    n148 = Open/Create/Replace File(file path (use dialog)=w170, operation (0:open)=T11."open or create") -> (refnum out=w158:refnum<file>)  [unwired: 4 in, 2 out]
                    n149 = Open/Create/Replace File(file path (use dialog)=w169, operation (0:open)=T11."open or create") -> (refnum out=w159:refnum<file>)  [unwired: 4 in, 2 out]
                    n150 = Open/Create/Replace File(file path (use dialog)=w168, operation (0:open)=T11."open or create") -> (refnum out=w160:refnum<file>)  [unwired: 4 in, 2 out]
                    n151 = Get File Size(file=w157) -> (refnum out=→"FF_On_Ref":refnum<file>, size (in bytes)=→"FF_On_Ptr":i64)  [unwired: 1 in, 1 out]
                    n152 = Get File Size(file=w158) -> (refnum out=→"FF_Off_Ref":refnum<file>, size (in bytes)=→"FF_Off_Ptr":i64)  [unwired: 1 in, 1 out]
                    n153 = Get File Size(file=w159) -> (refnum out=→"NF_On_Ref":refnum<file>, size (in bytes)=→"NF_On_Ptr":i64)  [unwired: 1 in, 1 out]
                    n154 = Get File Size(file=w160) -> (refnum out=→"NF_Off_Ref":refnum<file>, size (in bytes)=→"NF_Off_Ptr":i64)  [unwired: 1 in, 1 out]
                  }
                  frame True {
                    # "Don't need to do anything!"
                  }
                }
              }
              frame #1 {
                # "Writing and plotting retrieved\nweather parameters"
                # "Matlab script goes online and retrieves most recent press, temp, and relative humidity data \nfrom the weather station on the roof of Cobleigh"
                # "Importing the current weather conditions from the COE weather station"
                n155 = disable-structure shown="Disabled" {
                  frame Disabled {
                    n156 = script code="%try\n%s=urlread('http://www.coe.montana.edu/ee/weather/mostCurrentCSV.php');\n%amin=textscan(s,'%s %s %s %s %s %s %s %s %s %s %s %s %s');\n%data=amin{1}{2};\n%[test remain]=strtok(data,',');\n%remain=str2num(remain);\n%press=remain(3)./1000;\n%temp=remain(5);\n%RH=remain(7);\n%catch\npress=.850;\ntemp=20;\nRH=40;\n%end"() -> ()  [unwired: 1 in, 4 out]
                  }
                  frame Enabled {
                  }
                }
                n157 = local read "WS_On/Off"() -> (w236:bool)
                n158 = case shown="True" w236 {
                  frame False {
                  }
                  frame True {
                    n159 = local read "WS visa"() -> (w241:refnum<visa-resource-name>)
                    n160 = call "T_RH_P.vi"("VISA in"=w241, "WS_Commands"=enum16{"OpenWS", "ReadTRHP", "CloseWS"}."ReadTRHP") -> ("TRHP"=w237:T13)  [unwired: 11 in, 2 out]
                    n161 = local write "TRHP"(w237) -> ()
                    n162 = Unbundle By Name(w237) -> ("Temp"=→"Temperature (C)":dbl, "RelH"=→"Relative Humdity (%)":dbl, "Press"=→"Pressure (mb)":dbl)
                  }
                }
              }
              frame #2 {
                # "Frame 3: Read, process, and plot online data\nFrame 4:\nFrame 5: Write the data to the folders from Frame 0 of outter sequence"
                # "Frame 0: Read the online wavelength and adjust to locking tolerance if out of range, Switch to offline DBR\nFrame 1: Read the output power from the Newport meter, calculate and plot the output pulse energy\nFrame 2: Wait 'Scalar Wait Time' for buffer to clear other wavelength data"
                # "Online"
                n163 = stacked-sequence {
                  frame #0 {
                    # "Read the online wavelength and continue adjusting the online DBR if outside the wavelength tolerance\nuntil it is within tolerance"
                    n164 = while {
                      i -> [w246]
                      stop <- w243 stop-if-true
                      # "Frame 2: Decrement DBR current if above tolerance\nFrame 3: Increment DBR current if below tolerance"
                      # "Frame 0: Read the current wavelength from the wavemeter\nFrame 1: Calculate the difference between desired and actual wavelength"
                      # "Continue reading and adjusting online DBR current until within locking tolerance"
                      n165 = stacked-sequence {
                        tunnel: w246 -> [w248 _ _ _ _]
                        tunnel: [_ _ w262 _ _] -> w244
                        frame #0 {
                          n166 = Equal To 0?(x=w248) -> (x = 0?=w247:bool)
                          n167 = case shown="True" w247 {
                            frame False {
                            }
                            frame True {
                              # "Set the TSOA switch to\namplify the ABSORBING\nwavelength"
                              n168 = Build Array(FALSE ("Boolean")) -> (w249:bool[])
                              n169 = call-poly <vilib>:"DAQmx Write.vi"("task/channels in"=refnum<k21> "BristolWM", "data"=w249) -> ()  [unwired: 11 in, 3 out]
                            }
                          }
                        }
                        frame #1 {
                          # "Reading the wavelength from the wavemeter"
                          n170 = flat-sequence {
                            tunnel: [w254] -> w253
                            tunnel: w253 -> [w257]
                            tunnel: [w256] -> w252
                            tunnel: w252 -> [w260]
                            frame #0 {
                              n171 = local read "Bristol In"() -> (w255:i32)
                              n172 = dll-call lib="C:/Users/H2ODial/Desktop/Shared Telescope WV DIAL Code/bristol/CLDevIface.dll" fn="CLOpenUSBSerialDevice"("commPort"=w255) -> ("return type"=w254:i32)  [unwired: 4 in, 2 out]
                            }
                            frame #1 {
                              n173 = dll-call lib="C:/Users/H2ODial/Desktop/Shared Telescope WV DIAL Code/bristol/CLDevIface.dll" fn="CLGetLambdaReading"("devHandle"=w257) -> ("return type"=→"Lambda On Read (nm)":dbl, "devHandle"=w256:i32)  [unwired: 3 in, 2 out]
                            }
                            frame #2 {
                              n174 = dll-call lib="C:/Users/H2ODial/Desktop/Shared Telescope WV DIAL Code/bristol/CLDevIface.dll" fn="CLCloseDevice"("commPort"=w260) -> ("return type"=w259:i32)  [unwired: 4 in, 2 out]
                              n175 = local write "Bristol Out"(w259) -> ()
                            }
                          }
                        }
                        frame #2 {
                          # "If WL difference is within tolerance, stop looping, and illuminate 'Wavelength Lock Online' indicator"
                          # "Calculating the difference between the actual and desired online wavelength"
                          n176 = local read "Lambda On Read (nm)"() -> (w261:dbl)
                          n177 = local read "Online_Tol"() -> (w267:dbl)
                          n178 = Multiply(x=-1.0, y=w267) -> (x*y=w268:dbl)
                          n179 = Subtract(x=w261, y="Lambda On Set (nm)") -> (x-y=w263:dbl)
                          "WL_Difference" <- w263
                          n180 = Greater?(x=w263, y=w268) -> (0:w264:bool)
                          n181 = Less?(x=w263, y=w267) -> (x < y?=w265:bool)
                          n182 = And(x=w264, y=w265) -> (x .and. y?=w262:bool)
                          "Wavelength Lock Online" <- w262
                        }
                        frame #3 {
                          # "If the wavelength difference is greater that 0.0002 nm, decrement the \nDBR current by 0.01 mA"
                          n183 = local read "WL_Difference"() -> (w272:dbl)
                          n184 = Greater Or Equal?(x=w272, y="Online_Tol") -> (x >= y?=w271:bool)
                          n185 = case shown="True" w271 {
                            frame False {
                              # "Wavelength difference is not greater than 0.0002 nm, do nothing"
                            }
                            frame True {
                              # "Generating a command string\nto decrement the current"
                              # "WL difference is greater than 0.0002 nm,\ndecrement the DBR current by 0.01 mA"
                              n186 = local read "Settings"() -> (w279:T7)
                              n187 = local read "y"() -> (w273:dbl)
                              n188 = Unbundle By Name(w279) -> ("OnLineTEC"=w277:dbl)
                              n189 = local read "Device In"() -> (w274:refnum<visa-resource-name>)
                              n190 = Subtract(x=w277, y=w273) -> (x-y=w276:dbl)
                              n191 = Bundle By Name(cluster=w279, "OnLineTEC"=w276, "Module"=T12."On Line TEC") -> (w281:T7)
                              n192 = call "TL_Driver.vi"("Device In"=w274, "Commands"=T9."SET", "Settings"=w281) -> ("Readings"=w280:T6)  [unwired: 9 in, 3 out]
                              n193 = local write "Settings"(w281) -> ()
                              n194 = local write "Readings"(w280) -> ()
                            }
                          }
                        }
                        frame #4 {
                          # "If WL difference is < 0.0002 nm, increment the DBR current"
                          n195 = local read "Online_Tol"() -> (w283:dbl)
                          n196 = local read "WL_Difference"() -> (w286:dbl)
                          n197 = Multiply(x=-1.0, y=w283) -> (x*y=w282:dbl)
                          n198 = Less Or Equal?(x=w286, y=w282) -> (x <= y?=w285:bool)
                          n199 = case shown="True" w285 {
                            frame False {
                              # "WL difference is no <= to -0.0002 nm, do nothing"
                            }
                            frame True {
                              # "WL difference is < -0.0002,\nincrement the DBR current by 0.01 mA"
                              # "Generating a command string\nto decrement the current"
                              n200 = local read "Settings"() -> (w295:T7)
                              n201 = Unbundle By Name(w295) -> ("OnLineTEC"=w291:dbl)
                              n202 = local read "y"() -> (w287:dbl)
                              n203 = local read "Device In"() -> (w288:refnum<visa-resource-name>)
                              n204 = Add(x=w291, y=w287) -> (x+y=w290:dbl)
                              n205 = Bundle By Name(cluster=w295, "OnLineTEC"=w290, "Module"=T12."On Line TEC") -> (w294:T7)
                              n206 = call "TL_Driver.vi"("Device In"=w288, "Commands"=T9."SET", "Settings"=w294) -> ("Readings"=w293:T6)  [unwired: 9 in, 3 out]
                              n207 = local write "Settings"(w294) -> ()
                              n208 = local write "Readings"(w293) -> ()
                            }
                          }
                        }
                      }
                      n209 = Or(x=w244, y="Cancel online") -> (x .or. y?=w243:bool)
                    }
                  }
                  frame #1 {
                    # "Converting to pulse energy, assumes 5 percent pickoff"
                    # "Reading the Newport Power meter"
                    # "Reading the output power of the laser transmitter from the Newport power meter, once read, convert to corresponding pulse energy and plot"
                    n210 = local read "Newport Device Key"() -> (w300:string)
                    n211 = local read "NewportRef"() -> (w296:refnum<k24>)
                    n212 = disable-structure shown="Disabled" {
                      frame Disabled {
                        # "Plotting the online and offling pulse energies"
                        n213 = local read "Online Pulse Energy"() -> (w311:dbl)
                        n214 = local read "Offline Pulse Energy"() -> (w310:dbl)
                        n215 = Bundle("Online Pulse Energy"=w311, "Offline Pulse Energy"=w310) -> (→"Pulse Energy (Micro Joule)":T15)  [unwired: 1 in]
                      }
                      frame Enabled {
                      }
                    }
                    n216 = Number To Decimal String(number="SampleSize") -> (decimal integer string=w298:string)  [unwired: 1 in]
                    n217 = invoke class="PowerMeterCommands" method="PerformDAQ"(reference=w296, "deviceKey"=w300, "interval"="1", "sampleSize"=w298) -> ("PerformDAQ"=w301:dbl[])  [unwired: 2 in, 5 out]
                    n218 = call-poly <vilib>:"Mean.vi"("X"=w301) -> ("mean"=w299:dbl)  [unwired: 1 out]
                    n219 = Multiply(x=w299, y=1000.0) -> (x*y=w307:dbl)
                    n220 = Divide(x=w307, y=0.05) -> (x/y=w305:dbl)
                    n221 = Divide(x=w305, y=7.0) -> (x/y=→"Online Pulse Energy":dbl)
                  }
                  frame #2 {
                    # "Wait 'Scalar Wait Time' for the next available batch of scalar card data"
                    n222 = local read "AMCS_Profile"() -> (w312:i32)
                    n223 = disable-structure shown="Disabled" {
                      frame Disabled {
                        # "Waiting 'Scalar Wait Time'"
                        n224 = Wait (ms)(milliseconds to wait="Scalar Wait Time") -> ()  [unwired: 1 out]
                      }
                      frame Enabled {
                      }
                    }
                    n225 = while {
                      tunnel: [w319] -> w313
                      tunnel: [w315] -> _
                      tunnel: w312 -> [w315]
                      stop <- w317 stop-if-true
                      n226 = global read "AMCS_Data.vi" "AMCS_Profile"() -> (w319:i32)
                      n227 = Wait (ms)(milliseconds to wait=u32 10) -> ()  [unwired: 1 out]
                      n228 = Equal?(x=w319, y=w315) -> (x = y?=w318:bool)
                      n229 = case shown="False" w318 {
                        tunnel: [TRUE FALSE] -> w317
                        frame False {
                        }
                        frame True {
                        }
                      }
                    }
                    "AMCS_Profile" <- w313
                  }
                  frame #3 {
                    # "convert time per range bin to meters\nand calculate smoothed bins using\nsmoothing range"
                    # "Plotting online cross section and smoothed online data"
                    # "Calculate the bin by bin mean of the data"
                    # "Collect 'Integration Period (Seconds)' number\nof scalar data"
                    # "Reading, processing, and plotting the online data"
                    n230 = local read "Data Reads (number of loops)"() -> (w347:i32)
                    n231 = for {
                      N: w347 -> [_]
                      tunnel: [w368] -> w359 mode=indexing
                      tunnel: [w367] -> w322 mode=indexing
                      # "Scalar Data is retrieved from Global \nVariable that scaler.vi is writing to,"
                      n232 = global read "AMCS_Data.vi" "AMCS_Data"() -> (w371:u16[][])
                      n233 = disable-structure shown="Disabled" {
                        frame Disabled {
                          n234 = global read "Scalar_Data_3.vi" "Scalar Data 3"() -> ()  [unwired: 1 out]
                          n235 = global read "Scalar_Data.vi" "Scalar Data"() -> ()  [unwired: 1 out]
                        }
                        frame Enabled {
                        }
                      }
                      n236 = Index Array(array=w371, index (row) #1=0 ("index (row)"), index (row) #2=2 ("index (row)")) -> (element #1=w368:u16[], element #2=w367:u16[])  [unwired: 2 in]
                    }
                    n237 = Transpose 2D Array(2D array=w359) -> (transposed array=w363:u16[][])
                    n238 = Transpose 2D Array(2D array=w322) -> (transposed array=w345:u16[][])
                    n239 = for {
                      tunnel: w363 -> [w373] mode=indexing
                      tunnel: [w372] -> w364 mode=indexing
                      n240 = call-poly <vilib>:"Mean.vi"("X"=w373) -> ("mean"=w372:dbl)  [unwired: 1 out]
                    }
                    n241 = for {
                      tunnel: w345 -> [w366] mode=indexing
                      tunnel: [w365] -> w346 mode=indexing
                      n242 = call-poly <vilib>:"Mean.vi"("X"=w366) -> ("mean"=w365:dbl)  [unwired: 1 out]
                    }
                    n243 = local read "bins"() -> (w339:u32)
                    n244 = Array Subset(array=w364, index=1 ("dimension size"), length=w339) -> (w351:dbl[])
                    n245 = Array Subset(array=w346, index=1 ("dimension size"), length=w339) -> (w343:dbl[])
                    n246 = local read "background length"() -> (w329:i32)
                    n247 = local read "background start"() -> (w330:u32)
                    n248 = Array Size(array=w351) -> (size(s)=w348:i32)
                    n249 = Array Size(array=w343) -> (size(s)=w340:i32)
                    n250 = Initialize Array(1.0 ("element"), w348) -> (w350:dbl[])
                    n251 = Initialize Array(1.0 ("element"), w340) -> (w342:dbl[])
                    n252 = Multiply(x=w351, y=w350) -> (x*y=w352:dbl[])
                    "On-Line Bin Readings" <- w352
                    n253 = Multiply(x=w343, y=w342) -> (x*y=w333:dbl[])
                    "On-Line Bin Readings 2" <- w333
                    n254 = local read "Total DIAL Integration Time (Minutes)"() -> (w355:i32)
                    n255 = local read "Time Resolution Per Bin(ns)"() -> (w325:u32)
                    n256 = Array Subset(array=w352, index=w330, length=w329) -> (w361:dbl[])
                    n257 = Array Subset(array=w333, index=w330, length=w329) -> (w335:dbl[])
                    n258 = call-poly <vilib>:"Mean.vi"("X"=w361) -> ("mean"=w360:dbl)  [unwired: 1 out]
                    n259 = call-poly <vilib>:"Mean.vi"("X"=w335) -> ("mean"=w336:dbl)  [unwired: 1 out]
                    n260 = Divide(x=w355, y=w347) -> (x/y=w353:dbl)
                    n261 = local read "Index"() -> (w334:i32)
                    n262 = Subtract(x=w352, y=w360) -> (x-y=w357:dbl[])
                    n263 = Subtract(x=w333, y=w336) -> (x-y=w337:dbl[])
                    n264 = To Double Precision Float(number=w325) -> (double precision float=w326:dbl)
                    n265 = Multiply(x=w353, y=60.0) -> (x*y=w331:dbl)
                    n266 = Multiply(x=w326, y=0.15) -> (x*y=w328:dbl)
                    n267 = call "Ring Buffer Online Far.vi"("Index"=w334, "Profiles to Average"=w331, "Input Array"=w357) -> ("AvgArray"=w356:dbl[])  [unwired: 7 in, 1 out]
                    n268 = call "Ring Buffer Online Near.vi"("Index"=w334, "Profiles to Average"=w331, "Input Array"=w337) -> ("AvgArray"=w338:dbl[])  [unwired: 7 in, 1 out]
                    n269 = Divide(x="Smoothing Range", y=w328) -> (x/y=w323:dbl)
                    "Smoothed Bins" <- w323
                    n270 = call "Smooth Arrray.vi"("smooth size"=w323, "Raw Array"=w356) -> ("Smoothed Array"=→"On-Line  Smoothed":dbl[])  [unwired: 9 in]
                    n271 = call "Smooth Arrray.vi"("smooth size"=w323, "Raw Array"=w338) -> ("Smoothed Array"=→"HSRL molecular Smoothed":dbl[])  [unwired: 9 in]
                    n272 = disable-structure shown="Disabled" {
                      frame Disabled {
                        n273 = script code="format long;\ncounts=sum(Online);\nif counts >=0.5e6\ntime=time;\nelse\ntime=time\nend"() -> ()  [unwired: 3 in, 2 out]
                      }
                      frame Enabled {
                      }
                    }
                  }
                  frame #4 {
                    # "Toggling the Agiltron switch to the offline DBR seed laser"
                    n274 = disable-structure shown="Disabled" {
                      frame Disabled {
                        n275 = flat-sequence {
                          frame #0 {
                            # "Second one"
                            # "Command the switch to switch to position 2\ncorresponding to the offline DBR"
                            # "Hex string command \ncorrespond to offline"
                            n276 = VISA Write(VISA resource name="Switch Comm Port", write buffer="\u0001\u0012\u0000\u0001") -> ()  [unwired: 1 in, 3 out]
                          }
                        }
                      }
                      frame Enabled {
                      }
                    }
                  }
                  frame #5 {
                    # "Save the recently collected online data if 'Save Data?' is true"
                    n277 = case shown="True" "Save Data?" {
                      frame False {
                        # "'Save Data?' is false, do nothing"
                      }
                      frame True {
                        # "'Save Data?' is true, save onfline data to the Data Disk"
                        # "Write only one copy of data at this time"
                        # "Retrieve Julian Date"
                        n278 = local read "Time Resolution Per Bin(ns)"() -> (w383:u32)
                        n279 = local read "Number of Accumulates"() -> (w381:u32)
                        n280 = local read "Number of Bins"() -> (w382:u32)
                        n281 = local read "Lambda On Read (nm)"() -> (w377:dbl)
                        n282 = local read "Lambda On DBR Current"() -> (w405:dbl)
                        n283 = local read "On-Line Bin Readings 2"() -> (w403:dbl[])
                        n284 = local read "On-Line Bin Readings"() -> (w407:dbl[])
                        n285 = local read "Online Pulse Energy"() -> (w404:dbl)
                        n286 = To Double Precision Float(number=w383) -> (double precision float=w378:dbl)
                        n287 = To Double Precision Float(number=w382) -> (double precision float=w379:dbl)
                        n288 = To Double Precision Float(number=w381) -> (double precision float=w380:dbl)
                        n289 = call "Julian_Date_2.vi"() -> ("Julian Date"=w406:dbl)  [unwired: 11 in]
                        n290 = Build Array (concatenate)(w406, w377, w405, w404, w378, w379, w380, w407) -> (w398:dbl[])
                        n291 = Build Array (concatenate)(w406, w377, w405, w404, w378, w379, w380, w403) -> (w388:dbl[])
                        n292 = local write "DataOpen"(TRUE ("DataOpen")) -> ()
                        n293 = local read "NF_On_Ref"() -> (w386:refnum<file>)
                        n294 = local read "FF_On_Ref"() -> (w402:refnum<file>)
                        n295 = local read "NF_On_Ptr"() -> (w387:i64)
                        n296 = local read "FF_On_Ptr"() -> (w401:i64)
                        n297 = Set File Position(offset (in bytes) (0)=w401, refnum=w402) -> (refnum out=w399:refnum<file>, error out=w396:errorcluster)  [unwired: 2 in]
                        n298 = Set File Position(offset (in bytes) (0)=w387, refnum=w386) -> (refnum out=w392:refnum<file>, error out=w390:errorcluster)  [unwired: 2 in]
                        n299 = Write to Binary File(file (use dialog)=w392, data=w388, error in=w390, 5:FALSE ("prepend array or string size? (T)")) -> (refnum out=w391:refnum<file>, error out=w389:errorcluster)  [unwired: 2 in, 1 out]
                        n300 = Write to Binary File(file (use dialog)=w399, data=w398, error in=w396, 5:FALSE ("prepend array or string size? (T)")) -> (refnum out=w397:refnum<file>, error out=w395:errorcluster)  [unwired: 2 in, 1 out]
                        n301 = Get File Position(4:w389, 7:w391) -> (2:w385:i64)  [unwired: 2 out]
                        n302 = Get File Position(4:w395, 7:w397) -> (2:w394:i64)  [unwired: 2 out]
                        n303 = local write "NF_On_Ptr"(w385) -> ()
                        n304 = local write "FF_On_Ptr"(w394) -> ()
                      }
                    }
                  }
                }
              }
              frame #3 {
                # "Frame 3: Read offline data, calculate aerosol data, and plot offline and normalized relative backscatter\nFrame 4:\nFrame 5: Save the offline data and related information"
                # "Frame 0: Read the offline wavelength and lock if necessary, Switch to online DBR\nFrame 1: Read the output power from the Newport power meter\nFrame 2: Wait 'Scalar Wait Time' for buffers to clear of online contiminated data"
                # "offline"
                n305 = stacked-sequence {
                  frame #0 {
                    # "Every 60 data collection cycles, read the offline DBR wavelength, and if outside of wavelength tolerance, adjust DBR current until within tolerance"
                    n306 = local read "L_Count"() -> (w409:i32)
                    n307 = Quotient & Remainder(x=w409, y=60.0) -> (x-y*floor(x/y)=w410:dbl)  [unwired: 1 out]
                    n308 = Equal To 0?(x=w410) -> (x = 0?=w408:bool)
                    n309 = case shown="True" w408 {
                      frame False {
                      }
                      frame True {
                        n310 = while {
                          i -> [w415]
                          stop <- w413 stop-if-true
                          # "If WL difference is within tolerance, stop looping, and illuminate 'Wavelength Lock Offline' indicator"
                          # "Frame 2: Decrement DBR current if above tolerance\nFrame 3: Increment DBR current if below tolerance"
                          # "Frame 0: Read the current wavelength from the wavemeter\nFrame 1: Calculate the difference between desired and actual wavelength"
                          # "Continue reading and adjusting offline DBR current until within locking tolerance"
                          n311 = stacked-sequence {
                            tunnel: w415 -> [w417 _ _ _ _]
                            tunnel: [_ _ w431 _ _] -> w412
                            frame #0 {
                              n312 = Equal To 0?(x=w417) -> (x = 0?=w416:bool)
                              n313 = case shown="True" w416 {
                                frame False {
                                }
                                frame True {
                                # "Set the TSOA switch to\namplify the non ABSORBING\nwavelength"
                                n314 = Build Array(TRUE ("Boolean")) -> (w419:bool[])
                                n315 = call-poly <vilib>:"DAQmx Write.vi"("task/channels in"=refnum<k21> "BristolWM", "data"=w419) -> ()  [unwired: 11 in, 3 out]
                                n316 = Wait (ms)(milliseconds to wait=u32 3200) -> ()  [unwired: 1 out]
                                }
                              }
                            }
                            frame #1 {
                              # "Reading the wavelength from the wavemeter"
                              n317 = flat-sequence {
                                tunnel: [w424] -> w423
                                tunnel: w423 -> [w427]
                                tunnel: [w426] -> w422
                                tunnel: w422 -> [w430]
                                frame #0 {
                                n318 = local read "Bristol In"() -> (w425:i32)
                                n319 = dll-call lib="C:/Users/H2ODial/Desktop/Shared Telescope WV DIAL Code/bristol/CLDevIface.dll" fn="CLOpenUSBSerialDevice"("commPort"=w425) -> ("return type"=w424:i32)  [unwired: 4 in, 2 out]
                                }
                                frame #1 {
                                n320 = dll-call lib="C:/Users/H2ODial/Desktop/Shared Telescope WV DIAL Code/bristol/CLDevIface.dll" fn="CLGetLambdaReading"("devHandle"=w427) -> ("return type"=→"Lambda Off Read (nm)":dbl, "devHandle"=w426:i32)  [unwired: 3 in, 2 out]
                                }
                                frame #2 {
                                n321 = dll-call lib="C:/Users/H2ODial/Desktop/Shared Telescope WV DIAL Code/bristol/CLDevIface.dll" fn="CLCloseDevice"("commPort"=w430) -> ("return type"=w429:i32)  [unwired: 4 in, 2 out]
                                n322 = local write "Bristol Out"(w429) -> ()
                                }
                              }
                            }
                            frame #2 {
                              # "Calculating the difference between the actual and desired online wavelength"
                              n323 = local read "Offline_Tol"() -> (w433:dbl)
                              n324 = local read "Lambda Off Read (nm)"() -> (w439:dbl)
                              n325 = Multiply(x=-1.0, y=w433) -> (x*y=w432:dbl)
                              n326 = Subtract(x=w439, y="Lambda Off Set (nm)") -> (x-y=w435:dbl)
                              "WL Difference off" <- w435
                              n327 = Greater?(x=w435, y=w432) -> (0:w436:bool)
                              n328 = Less?(x=w435, y=w433) -> (x < y?=w437:bool)
                              n329 = And(x=w436, y=w437) -> (x .and. y?=w431:bool)
                              "Wavelength Lock Offline" <- w431
                              n330 = case shown="True" w431 {
                                frame False {
                                }
                                frame True {
                                # "Set the TSOA switch to\namplify the ABSORBING\nwavelength"
                                n331 = Build Array(FALSE ("Boolean")) -> (w441:bool[])
                                n332 = call-poly <vilib>:"DAQmx Write.vi"("task/channels in"=refnum<k21> "BristolWM", "data"=w441) -> ()  [unwired: 11 in, 3 out]
                                n333 = Wait (ms)(milliseconds to wait=u32 3200) -> ()  [unwired: 1 out]
                                }
                              }
                            }
                            frame #3 {
                              # "If the wavelength difference is greater that 0.0002 nm, decrement the \nDBR current by 0.01 mA"
                              n334 = local read "WL Difference off"() -> (w446:dbl)
                              n335 = Greater Or Equal?(x=w446, y="Offline_Tol") -> (x >= y?=w445:bool)
                              n336 = case shown="True" w445 {
                                frame False {
                                # "Wavelength difference is not greater than 0.0002 nm, do nothing"
                                }
                                frame True {
                                # "Generating a command string\nto decrement the current"
                                n337 = local read "Settings"() -> (w453:T7)
                                n338 = Unbundle By Name(w453) -> ("OffLineTEC"=w450:dbl)
                                n339 = Subtract(x=w450, y="y") -> (x-y=w449:dbl)
                                n340 = local read "Device In"() -> (w447:refnum<visa-resource-name>)
                                n341 = Bundle By Name(cluster=w453, "OffLineTEC"=w449, "Module"=T12."Off Line TEC") -> (w454:T7)
                                n342 = call "TL_Driver.vi"("Device In"=w447, "Commands"=T9."SET", "Settings"=w454) -> ("Readings"=w455:T6)  [unwired: 9 in, 3 out]
                                n343 = local write "Settings"(w454) -> ()
                                n344 = local write "Readings"(w455) -> ()
                                }
                              }
                            }
                            frame #4 {
                              # "If WL difference is < 0.0002 nm, increment the DBR current"
                              n345 = local read "WL Difference off"() -> (w458:dbl)
                              n346 = Less Or Equal?(x=w458, y=-0.0001) -> (x <= y?=w456:bool)
                              n347 = case shown="True" w456 {
                                frame False {
                                # "WL difference is no <= to -0.0002 nm, do nothing"
                                }
                                frame True {
                                # "Generating a command string\nto decrement the current"
                                # "WL difference is less than 0.0002 nm,\nincrement the DBR current by 0.01 mA"
                                n348 = local read "Settings"() -> (w466:T7)
                                n349 = Unbundle By Name(w466) -> ("OffLineTEC"=w463:dbl)
                                n350 = local read "y"() -> (w459:dbl)
                                n351 = Add(x=w463, y=w459) -> (x+y=w462:dbl)
                                n352 = local read "Device In"() -> (w460:refnum<visa-resource-name>)
                                n353 = Bundle By Name(cluster=w466, "OffLineTEC"=w462, "Module"=T12."Off Line TEC") -> (w467:T7)
                                n354 = call "TL_Driver.vi"("Device In"=w460, "Commands"=T9."SET", "Settings"=w467) -> ("Readings"=w465:T6)  [unwired: 9 in, 3 out]
                                n355 = local write "Settings"(w467) -> ()
                                n356 = local write "Readings"(w465) -> ()
                                }
                              }
                            }
                          }
                          n357 = Or(x=w412, y="Cancel Offline") -> (x .or. y?=w413:bool)
                        }
                      }
                    }
                  }
                  frame #1 {
                    # "Reading the power meter"
                    # "Updating the pulse energy plot"
                    # "Converting to pulse energy"
                    # "Reading the offline output power, converting to pulse energy,  and updating the Pulse energy plot"
                    n358 = local read "SampleSize"() -> (w470:i32)
                    n359 = local read "Newport Device Key"() -> (w471:string)
                    n360 = local read "Online Pulse Energy"() -> (w477:dbl)
                    n361 = local read "Offline Pulse Energy"() -> (w476:dbl)
                    n362 = local read "NewportRef"() -> (w468:refnum<k24>)
                    n363 = Number To Decimal String(number=w470) -> (decimal integer string=w472:string)  [unwired: 1 in]
                    n364 = invoke class="PowerMeterCommands" method="PerformDAQ"(reference=w468, "deviceKey"=w471, "interval"="1", "sampleSize"=w472) -> ("PerformDAQ"=w473:dbl[])  [unwired: 2 in, 5 out]
                    n365 = Bundle("Online Pulse Energy"=w477, "Offline Pulse Energy"=w476) -> (w475:T15)  [unwired: 1 in]
                    n366 = local write "Pulse Energy (Micro Joule)"(w475) -> ()
                    n367 = call-poly <vilib>:"Mean.vi"("X"=w473) -> ("mean"=w469:dbl)  [unwired: 1 out]
                    n368 = Multiply(x=w469, y=1000.0) -> (x*y=w482:dbl)
                    n369 = Divide(x=w482, y=0.05) -> (x/y=w480:dbl)
                    n370 = Divide(x=w480, y=7.0) -> (x/y=→"Offline Pulse Energy":dbl)
                  }
                  frame #2 {
                    # "Added in the ability to interactively control the ThorLab  setting (just etalon temp for now)"
                    # "Wait 'Scalar Wait Time' for buffers to clear of online contiminated offline data"
                    n371 = disable-structure shown="Disabled" {
                      frame Disabled {
                        # "Wait 'Scalar Wait Time'"
                        n372 = local read "Scalar Wait Time"() -> (w492:u32)
                        n373 = Wait (ms)(milliseconds to wait=w492) -> ()  [unwired: 1 out]
                      }
                      frame Enabled {
                      }
                    }
                    n374 = event shown="[1] \"Settings.EtalonTEC\": Value Change" {
                      selector: _ -> [_ _]
                      dyn-events: _ -> [_ _]
                      timeout: 1 -> [_ _]
                      event Timeout {
                        n375 = event-data() -> ()  [unwired: 1 in, 2 out]
                      }
                      event "Settings.EtalonTEC": Value Change {
                        # "Generating a command string\nto update the etalon"
                        n376 = event-data() -> ()  [unwired: 1 in, 5 out]
                        n377 = local read "Settings"() -> (w488:T7)
                        n378 = Unbundle By Name(w488) -> ("EtalonTEC"=w491:dbl)
                        n379 = Bundle By Name(cluster=w488, "EtalonTEC"=w491, "Module"=T12."Etalon TEC") -> (w486:T7)
                        n380 = call "TL_Driver.vi"("Device In"=refnum<visa-resource-name> "Pro8000", "Commands"=T9."SET", "Settings"=w486) -> ("Readings"=w487:T6)  [unwired: 9 in, 3 out]
                        n381 = local write "Readings"(w487) -> ()
                        n382 = local write "Settings"(w486) -> ()
                      }
                    }
                  }
                  frame #3 {
                    w527 = 1 ("dimension size")
                    w531 = 1
                    # "Read in latest scalar card data from \n'Scalar Data' global variable that \nscaler.vi is writing to, then wait 1 sec\nfor next batch of data"
                    # "Plotting the normalized relative \nbackscatter"
                    # "Calculating the normalized relative backscatter"
                    # "Calculating/Plotting smoothed data,\ncross sections etc."
                    # "Pick off data with\nout header"
                    # "Calculate mean bin by bin mean"
                    # "Reading in 'Integration Period (Seconds)' of data"
                    # "Read the offline data from the scalar card, perform smoothing, calculate normalized relative backscatter, and plot"
                    # "File path in MATLAB script is of old dial is:\nF:\\Micropulse DIAL\\Micropulse DIAL Matlab\\\nFinal Overlap Function.mat')];"
                    # "Collects Data From Card,\nSends It To The Chart,\nAnd Saves A Copy As A\nFile If Option Selected On\nFront Panel"
                    n383 = for {
                      N: "Data Reads (number of loops)" -> [_]
                      tunnel: [w563] -> w495 mode=indexing
                      tunnel: [w562] -> w494 mode=indexing
                      n384 = global read "AMCS_Data.vi" "AMCS_Data"() -> (w564:u16[][])
                      n385 = disable-structure shown="Disabled" {
                        frame Disabled {
                          n386 = global read "Scalar_Data_4.vi" "Scalar Data 4"() -> ()  [unwired: 1 out]
                          n387 = global read "Scalar_Data_2.vi" "Scalar Data 2"() -> ()  [unwired: 1 out]
                        }
                        frame Enabled {
                        }
                      }
                      n388 = Index Array(array=w564, index (row) #1=1 ("index (row)"), index (row) #2=3 ("index (row)")) -> (element #1=w563:u16[], element #2=w562:u16[])  [unwired: 2 in]
                    }
                    n389 = local read "Total DIAL Integration Time (Minutes)"() -> (w552:i32)
                    n390 = Divide(x=w552, y="Data Reads (number of loops)") -> (x/y=w550:dbl)
                    n391 = local read "Total Aerosol Integration Time (Minutes)"() -> (w554:dbl)
                    n392 = local read "background length"() -> (w499:i32)
                    n393 = Multiply(x=w550, y=60.0) -> (x*y=w537:dbl)
                    n394 = local read "background start"() -> (w500:u32)
                    n395 = Transpose 2D Array(2D array=w495) -> (transposed array=w560:u16[][])
                    n396 = Transpose 2D Array(2D array=w494) -> (transposed array=w543:u16[][])
                    n397 = Divide(x=w554, y="Data Reads (number of loops)") -> (x/y=w555:dbl)
                    n398 = for {
                      tunnel: w560 -> [w570] mode=indexing
                      tunnel: [w569] -> w561 mode=indexing
                      tunnel: w543 -> [w568] mode=indexing
                      tunnel: [w567] -> _ mode=indexing
                      tunnel: [w567] -> w540 mode=indexing
                      n399 = call-poly <vilib>:"Mean.vi"("X"=w570) -> ("mean"=w569:dbl)  [unwired: 1 out]
                      n400 = call-poly <vilib>:"Mean.vi"("X"=w568) -> ("mean"=w567:dbl)  [unwired: 1 out]
                    }
                    n401 = local read "bins"() -> (w528:u32)
                    n402 = Multiply(x=w555, y=60.0) -> (x*y=w518:dbl)
                    n403 = Array Subset(array=w540, index=w527, length=w528) -> (w541:dbl[])
                    "Off-Line Bin Readings 2" <- w541
                    n404 = Array Subset(array=w561, index=w527, length=w528) -> (w539:dbl[])
                    "Off-Line  Bin Readings" <- w539
                    n405 = Array Subset(array=w541, index=w500, length=w499) -> (w542:dbl[])
                    n406 = Array Subset(array=w539, index=w500, length=w499) -> (w559:dbl[])
                    n407 = local read "Smoothed Bins"() -> (w496:dbl)
                    n408 = call-poly <vilib>:"Mean.vi"("X"=w542) -> ("mean"=w506:dbl)  [unwired: 1 out]
                    n409 = call-poly <vilib>:"Mean.vi"("X"=w559) -> ("mean"=w507:dbl)  [unwired: 1 out]
                    n410 = local read "Index"() -> (w517:i32)
                    n411 = Subtract(x=w541, y=w506) -> (x-y=w519:dbl[])
                    n412 = Subtract(x=w539, y=w507) -> (x-y=w535:dbl[])
                    n413 = call "Ring Buffer Offline Far.vi"("Index"=w517, "Profiles to Average"=w537, "Input Array"=w535) -> ("AvgArray"=w557:dbl[], "RingBufferOut"=→"RingBuffer offline far":dbl[][])  [unwired: 7 in]
                    n414 = call "Ring Buffer Aerosol Far.vi"("Index"=w517, "Profiles to Average"=w518, "Input Array"=w535) -> ("AvgArray"=w553:dbl[], "RingBufferOut"=→"RingBuffer aerosol far":dbl[][])  [unwired: 7 in]
                    n415 = call "Ring Buffer Offline Near.vi"("Index"=w517, "Profiles to Average"=w537, "Input Array"=w519) -> ("AvgArray"=w538:dbl[], "RingBufferOut"=→"RingBuffer offline near":dbl[][])  [unwired: 7 in]
                    n416 = call "Ring Buffer Aerosol Near.vi"("Index"=w517, "Profiles to Average"=w518, "Input Array"=w519) -> ("AvgArray"=w515:dbl[], "RingBufferOut"=→"RingBuffer aerosol near":dbl[][])  [unwired: 7 in]
                    n417 = Reshape Array(w535, w527, w528) -> (→"raw counts":dbl[][])
                    n418 = Reshape Array(w519, w527, w528) -> (→"raw counts near":dbl[][])
                    n419 = call "Smooth Arrray.vi"("smooth size"=w496, "Raw Array"=w557) -> ("Smoothed Array"=→"Off-Line Smoothed":dbl[])  [unwired: 9 in]
                    n420 = call "Smooth Arrray.vi"("smooth size"=w496, "Raw Array"=w553) -> ("Smoothed Array"=w526:dbl[])  [unwired: 9 in]
                    "Aerosol Smoothed" <- w526
                    n421 = call "Smooth Arrray.vi"("smooth size"=w496, "Raw Array"=w538) -> ("Smoothed Array"=→"HSRL combined":dbl[])  [unwired: 9 in]
                    n422 = call "Smooth Arrray.vi"("smooth size"=w496, "Raw Array"=w515) -> ("Smoothed Array"=w498:dbl[])  [unwired: 9 in]
                    "HSRL combined Smoothed" <- w498
                    n423 = local read "Time Resolution Per Bin(ns)"() -> (w493:u32)
                    n424 = local read "Number of Accumulates"() -> (w502:u32)
                    n425 = local read "Temperature (C)"() -> (w549:dbl)
                    n426 = local read "Pressure (mb)"() -> (w548:dbl)
                    n427 = script code="%accum_num=10000;     % scaler card setting number of accumulations\nt_bin = t_bin/1e9                 % scaler card setting time per bin\n%t_d = 37.3e-9;                % APD dead time from spec sheet\n\n% conversion from accumulated counts to count rate  (c/s)\nc_convert = 1./t_bin./accum_num;\nCR_far = p_raw_far.*c_convert;\nCR_near = p_raw_near.*c_convert;\nCR_total_far = (p_raw_far+b_far).*c_convert;\nCR_total_near = (p_raw_near+b_near).*c_convert;\nb_CR_far =b_far.*c_convert;\nb_CR_near =b_near.*c_convert;\n    \n%APD correction factor\n D_far = 1./(1-(t_d*CR_total_far));\n D_near = 1./(1-(t_d*CR_total_near));\n\n %Calculating normalize relative backscatter profile\n nrb_far = CR_far.*D_far.*r.^2.*1e-6;\n nrb_near = CR_near.*D_near.*r.^2.*1e-6;"("E"=6.0 ("Real"), "temp"=w549, "press"=w548, "p_raw_far"=w526, "b_far"=w507, "b_near"=w506, "p_raw_near"=w498, "accum_num"=w502, "t_d"="dead time", "t_bin"=w493) -> ("nrb_far"=w521:cdb[], "D_far"=w512:dbl[], "nrb_near"=w520:cdb[], "D_near"=w511:dbl[], "b_CR_far"=w504:dbl, "b_CR_near"=w503:dbl)  [unwired: 1 in, 1 out]
                    n428 = local read "bins"() -> (w530:u32)
                    n429 = local read "Altitude Array (km)"() -> (w523:dbl[])
                    n430 = Bundle(w504, w503) -> (→"?":cluster{dbl, dbl})  [unwired: 1 in]
                    n431 = Build Array(w521, w520) -> (w525:cdb[][])
                    n432 = Build Array(w512, w511) -> (w510:dbl[][])
                    n433 = Reshape Array(w520, w531, w530) -> (→"NRB 2":cdb[][])
                    n434 = Reshape Array(w521, w531, w530) -> (→"NRB":cdb[][])
                    n435 = Build Array(w523, w523) -> (w522:dbl[][])
                    n436 = call "Convert to Dynamic Data7"("2D Array"=w510) -> ("Dynamic Data Type"=w509:dynamicdata)  [unwired: 3 in]
                    n437 = call "Convert to Dynamic Data3"("2D Array"=w525) -> ("Dynamic Data Type"=w524:dynamicdata)  [unwired: 3 in]
                    n438 = call "Convert to Dynamic Data4"("2D Array"=w522) -> ("Dynamic Data Type"=w513:dynamicdata)  [unwired: 3 in]
                    n439 = call "Build XY Graph2"("Y Input"=w513, "X Input"=w524) -> ("XY Graph"=→"NRB plot":cluster{"Y":dbl[], "Y":dbl[]}[])  [unwired: 3 in, 6 out]
                    n440 = call "Build XY Graph4"("Y Input"=w513, "X Input"=w509) -> ("XY Graph"=→"Correction":cluster{"Y":dbl[], "Y":dbl[]}[])  [unwired: 3 in, 6 out]
                  }
                  frame #4 {
                    # "REPLACE WITH NEW AGILTRON TASK!"
                    # "Toggle Agiltron switch to online DBR"
                    n441 = disable-structure shown="Disabled" {
                      frame Disabled {
                        # "ABSORBING"
                        n442 = flat-sequence {
                          frame #0 {
                            # "Third one"
                            # "Command the switch to switch to position 1\ncorresponding to the online DBR"
                            # "Hex string command \ncorrespond to online"
                            n443 = local read "Switch Comm Port"() -> (w574:refnum<visa-resource-name>)
                            n444 = VISA Write(VISA resource name=w574, write buffer="\u0001\u0012\u0000\u0002") -> ()  [unwired: 1 in, 3 out]
                          }
                        }
                        n445 = Build Array(FALSE ("Boolean")) -> (w573:bool[])
                        n446 = call-poly <vilib>:"DAQmx Write.vi"("task/channels in"=refnum<k21> "AgiltronSwitch", "data"=w573) -> ()  [unwired: 11 in, 3 out]
                      }
                      frame Enabled {
                      }
                    }
                  }
                  frame #5 {
                    # "If 'Save Data?' is true, save all relavant offline info"
                    n447 = local read "Save Data?"() -> (w576:bool)
                    n448 = case shown="True" w576 {
                      frame False {
                        # "'Save Data?' is false, do nothing"
                      }
                      frame True {
                        # "Write only one data file at this time"
                        # "Retrive Julian Date"
                        # "'Save Data?' is true, save offline data to the Data Disk"
                        n449 = local read "Lambda Off DBR Current"() -> (w598:dbl)
                        n450 = local read "Off-Line Bin Readings 2"() -> (w595:dbl[])
                        n451 = local read "Lambda Off Read (nm)"() -> (w597:dbl)
                        n452 = local read "Off-Line  Bin Readings"() -> (w603:dbl[])
                        n453 = local read "Relative Humdity (%)"() -> (w602:dbl)
                        n454 = local read "Offline Pulse Energy"() -> (w599:dbl)
                        n455 = local read "Temperature (C)"() -> (w600:dbl)
                        n456 = local read "Pressure (mb)"() -> (w601:dbl)
                        n457 = call "Julian_Date_2.vi"() -> ("Julian Date"=w596:dbl)  [unwired: 11 in]
                        n458 = Build Array (concatenate)(w596, w597, w598, w599, w600, w601, w602, w603) -> (w581:dbl[])
                        n459 = Build Array (concatenate)(w596, w597, w598, w599, w600, w601, w602, w595) -> (w578:dbl[])
                        n460 = local read "FF_Off_Ref"() -> (w583:refnum<file>)
                        n461 = local read "NF_Off_Ref"() -> (w580:refnum<file>)
                        n462 = local read "FF_Off_Ptr"() -> (w582:i64)
                        n463 = local read "NF_Off_Ptr"() -> (w579:i64)
                        n464 = Set File Position(offset (in bytes) (0)=w582, refnum=w583) -> (refnum out=w594:refnum<file>, error out=w592:errorcluster)  [unwired: 2 in]
                        n465 = Set File Position(offset (in bytes) (0)=w579, refnum=w580) -> (refnum out=w590:refnum<file>, error out=w588:errorcluster)  [unwired: 2 in]
                        n466 = Write to Binary File(file (use dialog)=w594, data=w581, error in=w592, 5:FALSE ("prepend array or string size? (T)")) -> (refnum out=w593:refnum<file>, error out=w591:errorcluster)  [unwired: 2 in, 1 out]
                        n467 = Write to Binary File(file (use dialog)=w590, data=w578, error in=w588, 5:FALSE ("prepend array or string size? (T)")) -> (refnum out=w589:refnum<file>, error out=w587:errorcluster)  [unwired: 2 in, 1 out]
                        n468 = Get File Position(4:w591, 7:w593) -> (2:w584:i64)  [unwired: 2 out]
                        n469 = Get File Position(4:w587, 7:w589) -> (2:w577:i64)  [unwired: 2 out]
                        n470 = local write "FF_Off_Ptr"(w584) -> ()
                        n471 = local write "NF_Off_Ptr"(w577) -> ()
                      }
                    }
                  }
                }
              }
              frame #4 {
                n472 = First Call?() -> (First Call?: T/F=w606:bool)
                n473 = Or(x="calculate absorption cross sections", y=w606) -> (x .or. y?=w604:bool)
                n474 = case shown="True" w604 {
                  frame False {
                  }
                  frame True {
                    # "calculate absorption cross sections from HITRAN data base"
                  }
                }
              }
              frame #5 {
                # "Data Processing Far Channel"
                # "Calculating the range resolved water vapor number density and plotting"
              }
            }
          }
        }
        "L_Count" <- w132
      }
    }
  }
  n475 = case shown="True" w3 {
    frame False {
    }
    frame True {
      # "close data files"
      n476 = local read "NF_Off_Ref"() -> (w608:refnum<file>)
      n477 = local read "NF_On_Ref"() -> (w609:refnum<file>)
      n478 = local read "FF_Off_Ref"() -> (w610:refnum<file>)
      n479 = local read "FF_On_Ref"() -> (w611:refnum<file>)
      n480 = local read "WS_On/Off"() -> (w607:bool)
      n481 = case shown="True" w607 {
        frame False {
        }
        frame True {
          n482 = local read "WS visa"() -> (w612:refnum<visa-resource-name>)
          n483 = call "T_RH_P.vi"("VISA in"=w612, "WS_Commands"=enum16{"OpenWS", "ReadTRHP", "CloseWS"}."CloseWS") -> ()  [unwired: 11 in, 3 out]
        }
      }
      n484 = Close File(refnum=w611) -> ()  [unwired: 1 in, 2 out]
      n485 = Close File(refnum=w610) -> ()  [unwired: 1 in, 2 out]
      n486 = Close File(refnum=w609) -> ()  [unwired: 1 in, 2 out]
      n487 = Close File(refnum=w608) -> ()  [unwired: 1 in, 2 out]
    }
  }
  "FileHour" <- -1 ("FileHour")
  "DataOpen" <- FALSE
